vi "ConvertGoop3ToGoop4.vi"() -> (0 "error out":errorcluster)   [LabVIEW 2020]
uses:
  <resource>/Framework/Providers/Open_GDS/ClassProviders/Common/ConvertGoop3ToGoop4_SubVIs/ConvertGoop3ToGoop4_ClassType.ctl
  <resource>/Framework/Providers/Open_GDS/ClassProviders/Common/LvClass_class/GDSLvCLass_ClassSettingsType.ctl
  <resource>/Framework/Providers/Open_GDS/ClassProviders/Common/LvClass_class/GDSLvClass_PlugIn.ctl
  <resource>/Framework/Providers/Open_GDS/ClassProviders/Common/LvClass_class/GDSLvClass_PlugInTypes.ctl
  <vilib>/Utility/miscctls.llb/LVPositionTypeDef.ctl
  <resource>/Framework/Providers/Open_GDS/ClassProviders/Provider_BaseClassInterface/CreateClassData.ctl
  <resource>/Framework/Providers/Open_GDS/ClassProviders/Provider_EndevoGOOP300/Templates/EndevoTemplateNames.ctl
  <resource>/Framework/Providers/Open_GDS/ClassProviders/Provider_EndevoGOOP400/Templates/EndevoG4TemplateNames.ctl
  <resource>/Framework/Providers/Open_GDS/ClassProviders/Provider_EndevoGOOP400/ClassWriterGOOP400_class/ClassWriterGOOP400.lvclass
  <resource>/Framework/Providers/Open_GDS/ClassProviders/Common/ScriptingFunctions/Scripting_ConnectorPanePatternType.ctl
  <resource>/Framework/Providers/Open_GDS/ClassProviders/Provider_BaseClassInterface/AddDesignPatternData.ctl
  <resource>/Framework/Providers/Open_GDS/ClassProviders/Common/CommonVIs/CommonVIs_AttributeDataType.ctl
  <resource>/Framework/Providers/Open_GDS/ClassProviders/Provider_BaseClassInterface/ClassWriter_class/ClassWriter.lvclass
  <vilib>/Utility/miscctls.llb/LVPointTypeDef.ctl
  <vilib>/Utility/error.llb/DialogType.ctl
  <resource>/Framework/Providers/Open_GDS/ClassProviders/Common/ConvertGoop3ToGoop4_SubVIs/ConvertGoop3ToGoop4_LogType.ctl
  <vilib>/regexp/Match Regular Expression.xnode
panel:
  in  "Cancel":bool
  in  "Next":bool
  out "Tab":T1(tab)
  out "ErrorMessage":string
  in  "Current GOOP3 top directory":path
  in  "Toggle":bool
  in  "GOOP3 classes found":i32[](listbox)
  in  "ApplyDebuggingSupport":bool
  in  "ApplyPersistentPattern":bool
  in  "Project":path caption="This project will be created and used to update the classes in."
  in  "Progress":i32(listbox)=-1
  in  "Done":bool
  out "State":string="Idle"
  out "Timer":string
  # "1."
  # "Select Top folder to start a recursive search for GOOP3 classes and application VIs."
  # "2."
  # "These classes\nhave been found.\n\nDo you want to convert them?"
  # "3."
  # "Have you backed up all your VIs in the selected folder?"
  # "Have you checked that all files in\nthe selected folder are writeable?"
  # "4."
  # "Save VI dialog boxes!?!\nIt might pop up dialog boxes that asks you to save VIs that will be unloaded from memory, JUST press cancel for those."
  # "Revert dialog boxes!?!\nIt might pop up dialog boxes that prompts that changes has been done on disk, JUST press cancel for those."
  # "5."
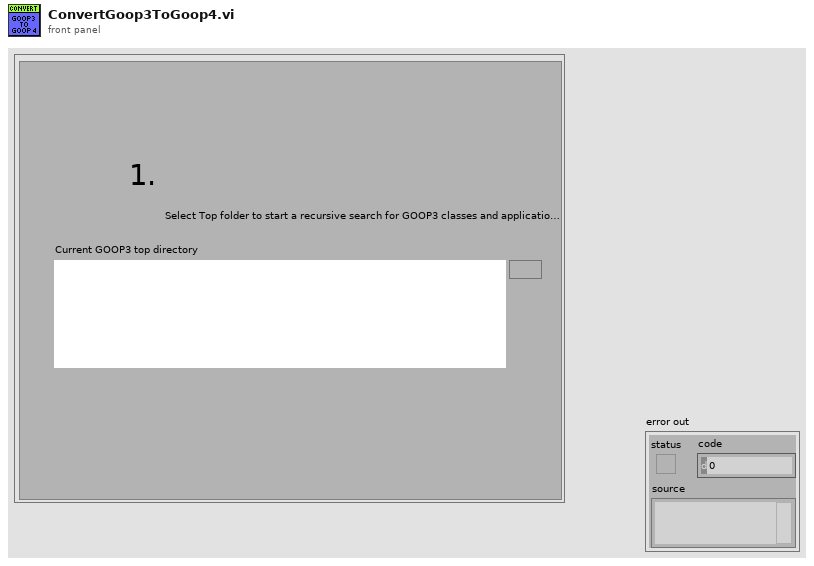
[diagram p1: front panel]
types:
  T1 = enum32{"SelectDir", "ClassesFound", "BackedUp", "Start?", "Converting"}
  T2 = typedef "ConvertGoop3ToGoop4_ClassType.ctl" = cluster{"NoOfInheritance":i32, "LvClassPath":path, "ClassName":string, "ClassPrefix":string, "IsLLB":bool, "ClassFolder":path, "ViRefs":refnum<vi>[], "ClassRef":refnum<vi>, "InheritsFrom":path, "RootClass":path, "ViPathes":path[], "AllInheritanceClasses":path[], "TemplateVersionUsed":string, "UsingClassAttributes":bool, "ClassSettings":T3, "HeaderIcon":u8[][], "GetAttViRefs":refnum<vi>[], "VIsModiifingData":refnum<vi>[], "Singleton":bool, "BrokenVIs":string[], "ObjectStatusUsed":bool, "DestrotCleanUpViName":string}
  T3 = typedef "GDSLvCLass_ClassSettingsType.ctl" = cluster{"ClassProviderName":string, "ClassTemplateUsed":string, "ClassTemplateVersion":string, "ClassDescription":string, "PlugIns":T4[], "ConnectorPanePattern":string}
  T4 = typedef "GDSLvClass_PlugIn.ctl" = cluster{"Type":T5, "ID":string, "Version":string, "Path":path, "Name":string, "Data":variant}
  T5 = typedef "GDSLvClass_PlugInTypes.ctl" = enum16{"DesignPattern", "MethodTypes"}
  T6 = typedef "LVPositionTypeDef.ctl" = cluster{"Left":i32, "Top":i32}
  T7 = cluster{"TopFolderPath":path, "Classes":T2[], "error":errorcluster, "Project":path, "ProjectRef":refnum<vi>, "My Computer":refnum<vi>, "AppRef":refnum<vi>, "CallParentMethod":cluster{"VIRef":refnum<vi>, "Position":T6}[], "CopyClasses":path, "TemplateVersions":string[], "LLBsToDelete":path[], "CopyClassesRef":refnum<vi>[], "CopyClassPaths":path[], "Deselect":bool, "SelectedClasses":i32[], "DeleteTheseFiles":path[], "Log":bool}
  T8 = enum8{"Enabled", "Disabled", "Disabled and Grayed Out"}
  T9 = cluster{"Current GOOP3 top directory":path, i32[]}
  T10 = typedef "ClassWriter.lvclass/CreateClassData.ctl" = cluster{"ClassName":string, "ClassFolder":path, "ClassDescription":string, "ClassTemplateOptions":string, "BaseClass(ProjectStringPath or LvClassFilePath)":variant, "ExtraCreateParameters":variant, "FolderSuffix":string}
  T11 = typedef "EndevoG4TemplateNames.ctl" = enum16{"G4BaseTemplate_Simple_4x4x4", "G4SubTemplate_Simple_4x4x4", "G4BaseTemplate_Simple_6x8x6", "G4SubTemplate_Simple_6x8x6", "G4BaseTemplate_Singleton_4x4x4", "G4SubTemplate_Singleton_4x4x4", "G4BaseTemplate_Singleton_6x8x6", "G4SubTemplate_Singleton_6x8x6", "G4InterfaceTemplate_6x8x6", "G4InterfaceTemplate_4x4x4", "G4BaseTemplate_Simple_5x6x5", "G4BaseTemplate_Singleton_5x6x5", "G4InterfaceTemplate_5x6x5", "G4SubTemplate_Simple_5x6x5", "G4SubTemplate_Singleton_5x6x5"}
  T12 = typedef "EndevoTemplateNames.ctl" = enum16{"BaseTemplate", "SubTemplate", "BaseTemplate_4x4x4", "SubTemplate_4x4x4", "SingletonTemplate"}
  T13 = cluster{"ID":string, "Path":path, "Name":string, "Desc":string, "Version":string, "DependenciesID":string[], "OnlyOne":bool}[]
  T14 = typedef "CommonVIs_AttributeDataType.ctl" = enum16{"UINT8", "INT8", "UINT16", "INT16", "UINT32", "INT32", "UINT64", "INT64", "SGL", "DBL", "EXT", "CSG", "CDB", "CXT", "TimeStamp", "STRING", "PATH", "BOOL", "ENUM", "RefNum", "VIRefNum", "LabVIEW Class", "Cluster", "Variant", "TypeDef", "Waveform", "LabVIEW Object", "Other", "void"}
  T15 = cluster{"ProcessName":cluster{"Name":string, "Array?":u16, "AttributeDataType":T14, "GetMethod":bool, "SetMethod":bool}[]}
  T16 = typedef "LVPointTypeDef.ctl" = cluster{"Horizontal":i16, "Vertical":i16}
  T17 = enum32{"invalid scope", "public", "private", "protected", "community"}
  T18 = typedef "ConvertGoop3ToGoop4_LogType.ctl" = enum16{"Enter", "Read"}
  T19 = typedef "eventvkey.ctl" = enum16{"ASCII", "Enter", "Return", "Shift", "Ctrl", "Alt", "Cmd", "Opt", "Caps", "NumLock", "Clear", "Break", "Up", "Down", "Left", "Right", "Insert", "Delete", "Home", "End", "PageUp", "PageDown", "Escape", "Help", "Pause", "ScrollLock", "F1", "F2", "F3", "F4", "F5", "F6", "F7", "F8", "F9", "F10", "F11", "F12", "F13", "F14", "F15", "F16", "F17", "F18", "F19", "F20", "F21", "F22", "F23", "F24", "Play", "VolumeUp", "VolumeDown", "Mute", "Two Byte Char"}
  T20 = enum32{"Bad", "Idle", "Run top level", "Running"}
  T21 = enum16{"Left Button", "Center Button", "Right Button", "Window Close"}
  T22 = typedef "Scripting_ConnectorPanePatternType.ctl" = u16
  T23 = typedef "GOOP_WireConfigurationType.ctl" = cluster{"Edge thickness":i32, "Edge color":u32, "Center thickness":i32, "Center pattern":T24, "CenterColor1":u32, "CenterColor2":u32, "Tunnels and terminals colors":u32}
  T24 = typedef "GOOP_WirePattern.ctl" = enum16{"Solid", "Large dash", "Small dash"}
  T25 = typedef "DesignPatternsData.ctl" = cluster{"Type":string, "Patterns":cluster{"ID":string, "Path":path, "Name":string, "Desc":string, "Version":string, "DependenciesID":string[], "OnlyOne":bool}[]}
  T26 = cluster{"ID":string, "Path":path, "Name":string, "Desc":string, "Version":string, "DependenciesID":string[], "OnlyOne":bool}
  T27 = typedef "AddDesignPatternData.ctl" = cluster{"Type":string, "ID":string, "Version":string, "VIPath":path, "Name":string, "Data":variant}
  T28 = enum32{"invalid VI type", "Standard VI", "Control VI", "Global VI", "Polymorphic VI", "Configuration VI", "SubSystem", "Facade VI", "Method VI", "Statechart Diagram VI"}
  T29 = typedef "DialogType.ctl" = u16
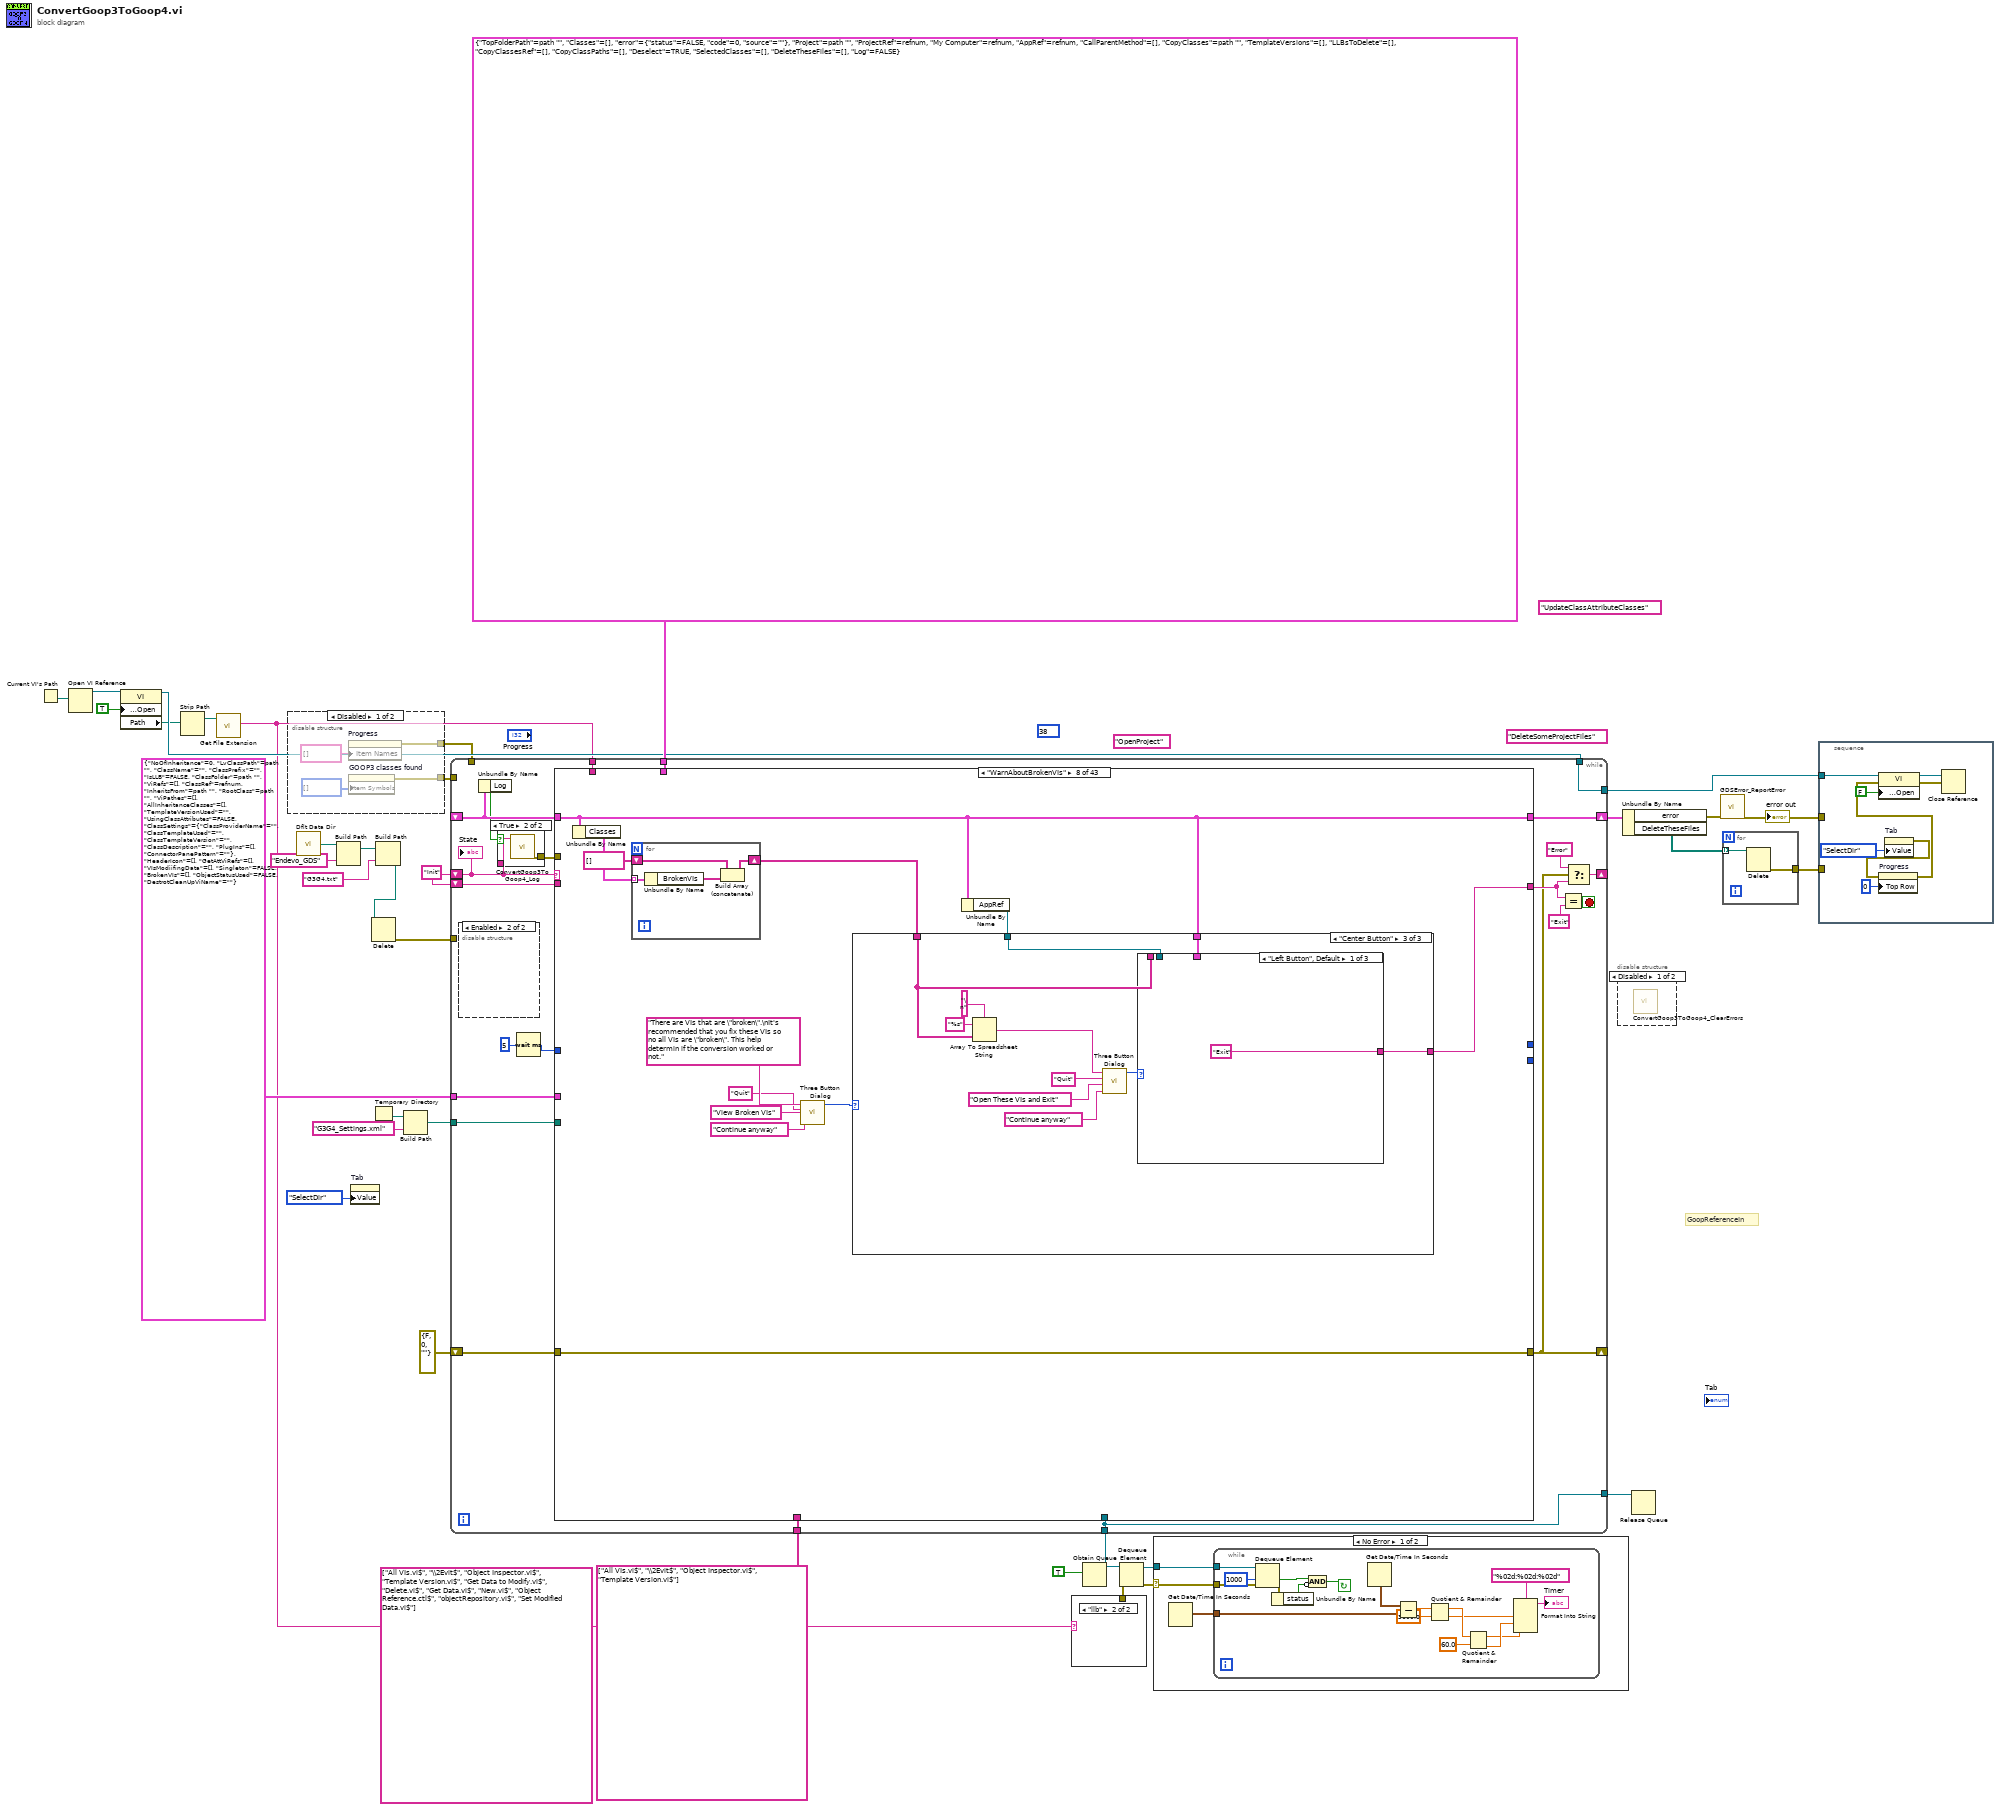
[diagram p0: block diagram]
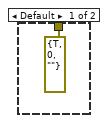
[diagram p2: hidden frame]
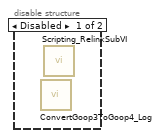
[diagram p7: hidden frame]
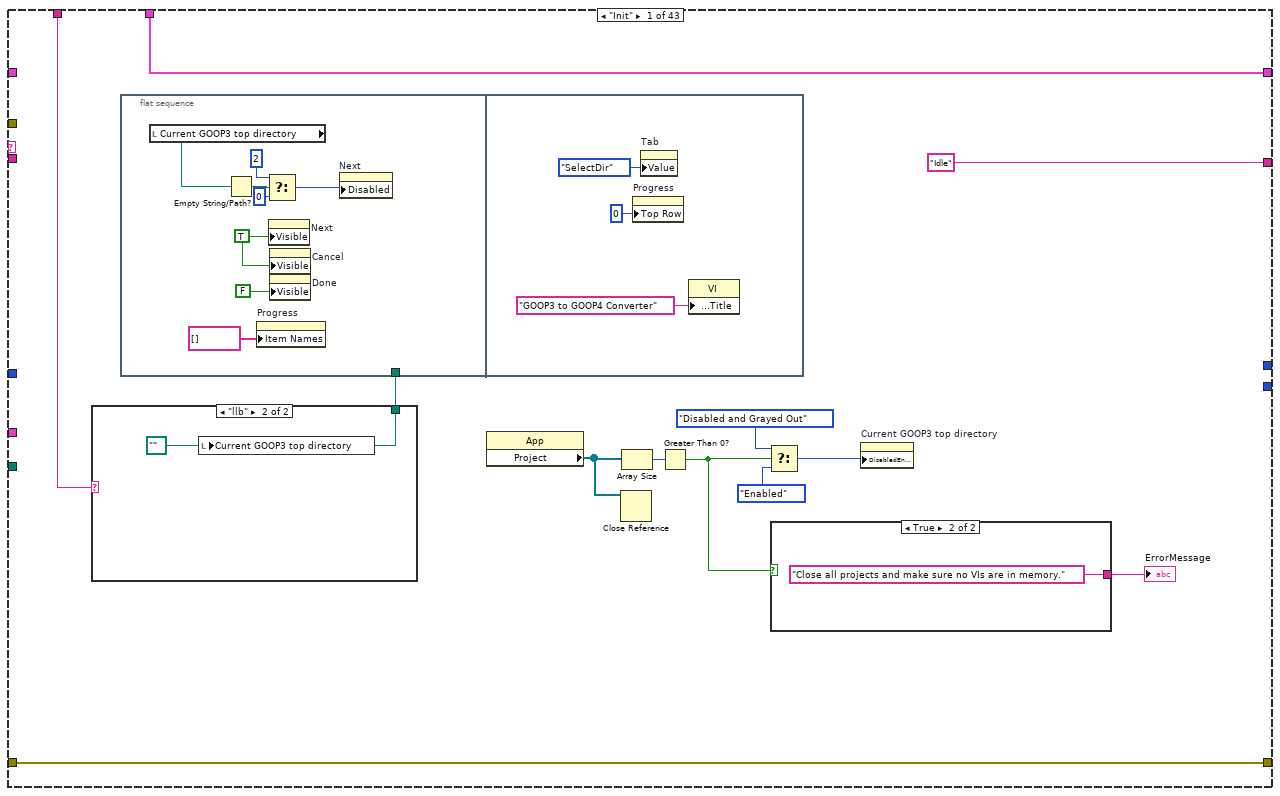
[diagram p8: hidden frame]
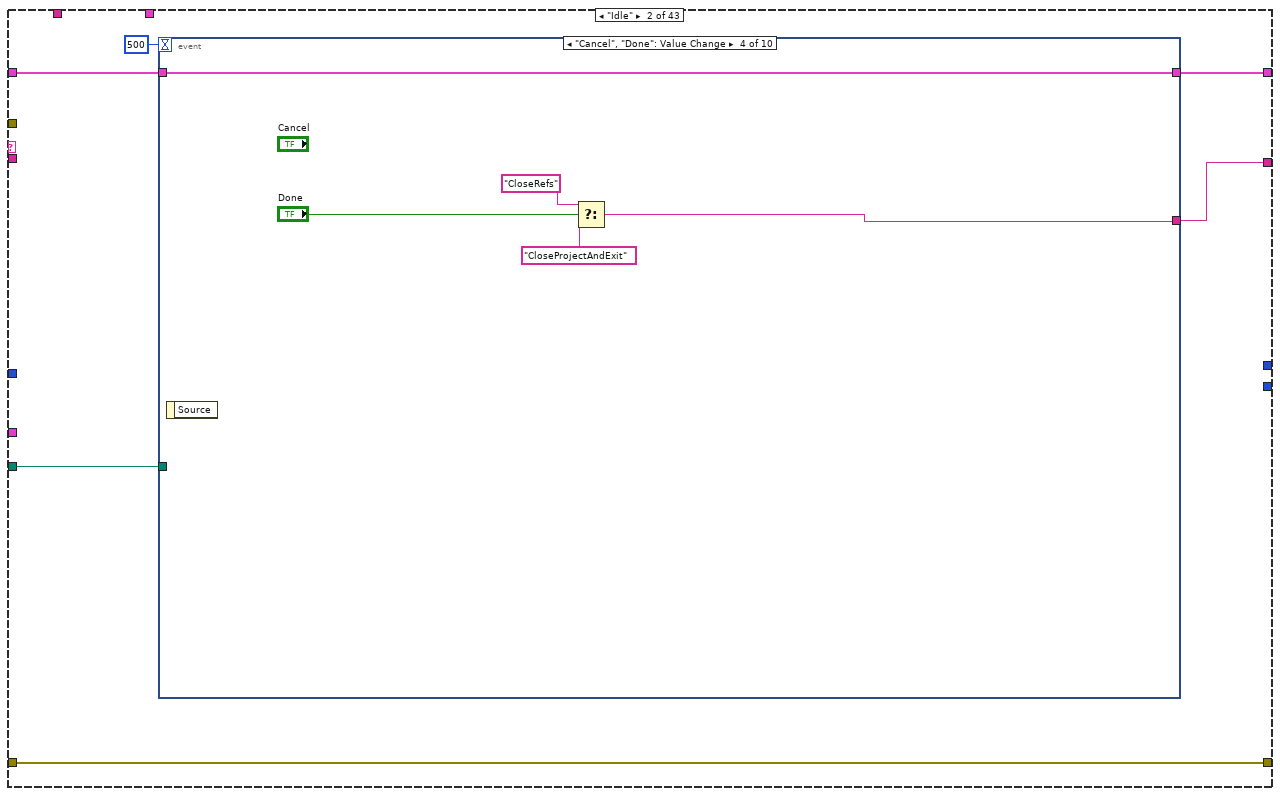
[diagram p11: hidden frame]
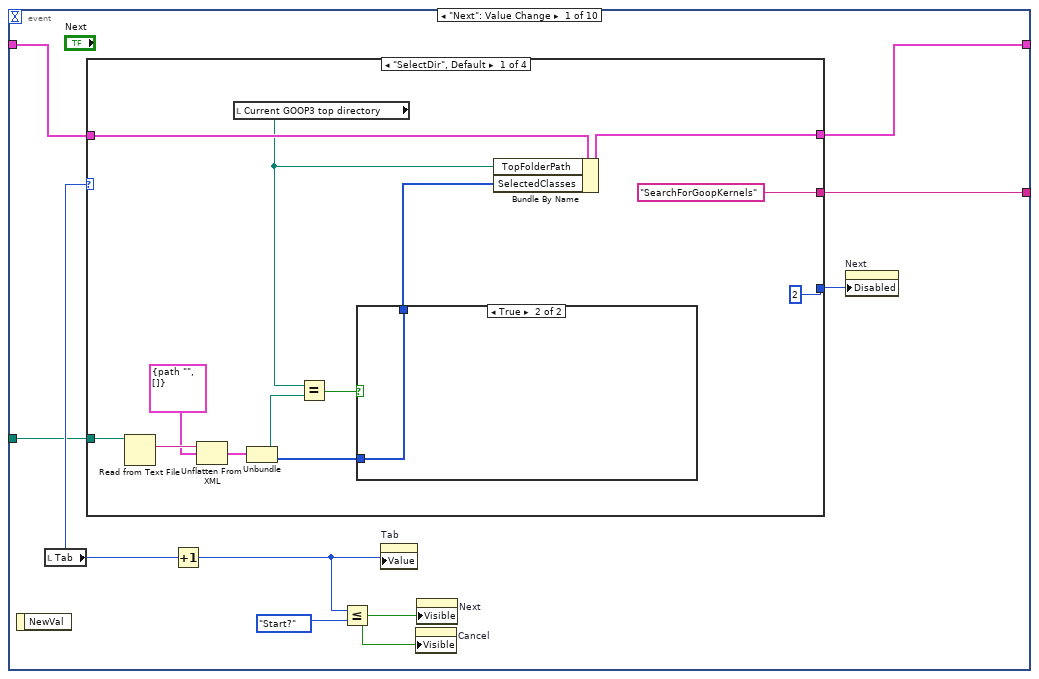
[diagram p12: hidden frame]
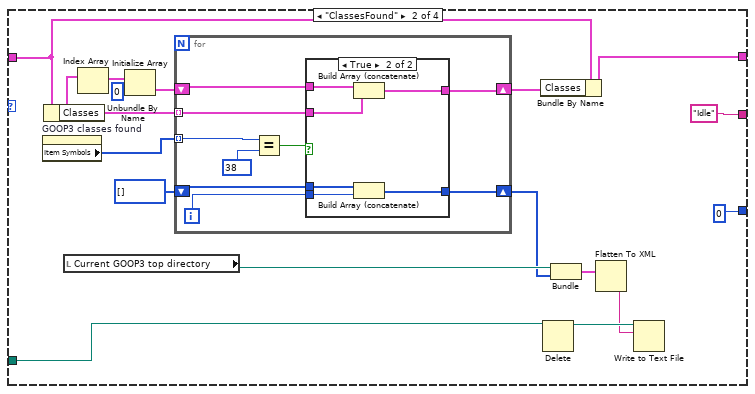
[diagram p14: hidden frame]
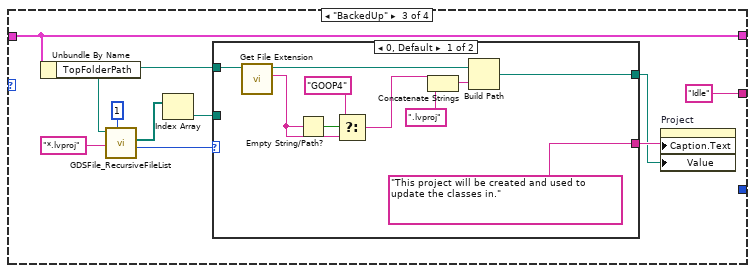
[diagram p16: hidden frame]
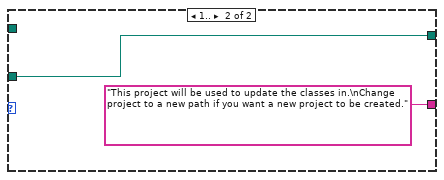
[diagram p17: hidden frame]
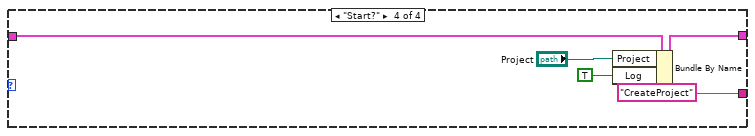
[diagram p18: hidden frame]
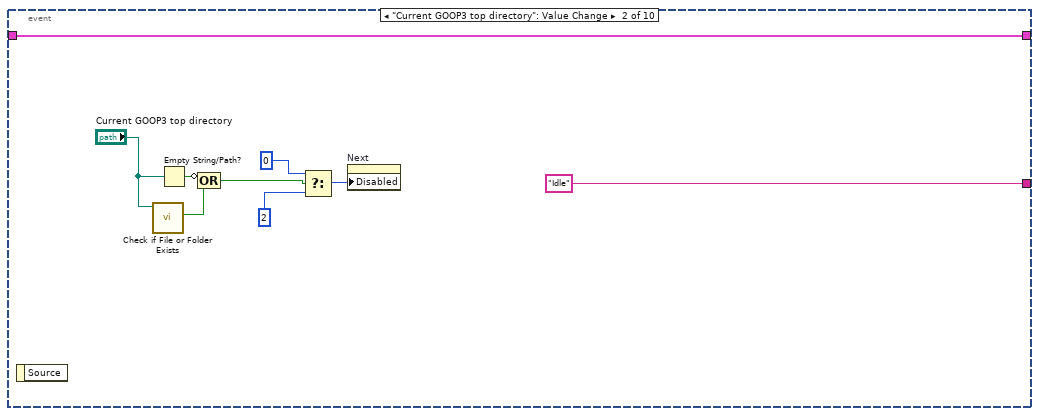
[diagram p19: hidden frame]
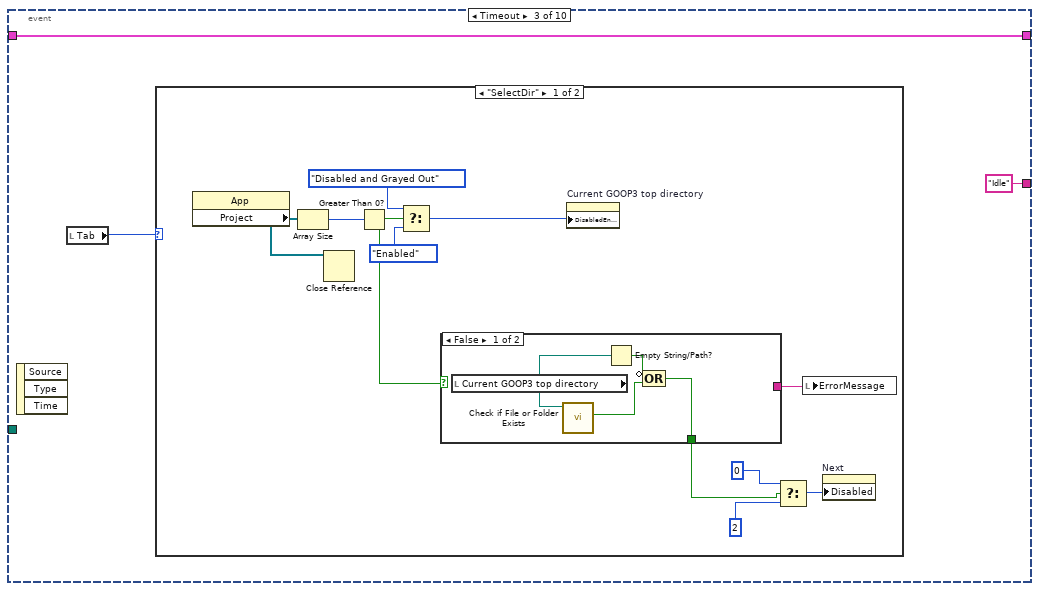
[diagram p20: hidden frame]
diagram:
  (unwired) "DeleteSomeProjectFiles"
  (unwired) "OpenProject"
  (unwired) 38
  (unwired) "UpdateClassAttributeClasses"
  (unwired) string[] ["All VIs.vi$", "\\2Evit$", "Object Inspector.vi$", "Template Version.vi$", "Get Data to Modify.vi$", "Delete.vi$", "Get Data.vi$", "New.vi$", "Object Reference.ctl$", "objectRepository.vi$", "Set Modified Data.vi$"] ("file names")
  w33 = "Init"
  # "GoopReferenceIn"
  n1 = Current VI's Path() -> (path=w29:path)
  n2 = Open VI Reference(vi path=w29) -> (vi reference=w28:refnum<vi>)  [unwired: 5 in, 1 out]
  n3 = property class="VI"(reference=w28, "Front Panel.Open"=TRUE ("Front Panel Window:Open")) -> (reference out=w27:refnum<vi>, "Path"=w15:path)  [unwired: 1 in, 1 out]
  n4 = Strip Path(path=w15) -> (stripped path=w14:path)  [unwired: 1 out]
  n5 = call <vilib>:"Get File Extension.vi"("file"=w14) -> ("lowercase file extension"=w3:string)  [unwired: 6 in, 4 out]
  n6 = disable-structure shown="Disabled" {
    disable-tunnel: [w38 _] -> w13
    disable-tunnel: [w37 _] -> w12
    frame Disabled {
      n7 = property on="Progress" class="LstBox (strict)"("Item Names"=string[] []) -> (error out=w37:errorcluster)  [unwired: 2 in, 1 out]
      n8 = property on="GOOP3 classes found" class="LstBox (strict)"("Item Symbols"=i32[] []) -> (error out=w38:errorcluster)  [unwired: 2 in, 1 out]
    }
    frame Enabled {
    }
  }
  n9 = call <vilib>:"Dflt Data Dir.vi"() -> ("App:Default Data Directory"=w9:path)
  n10 = Build Path(base path=w9, name or relative path="Endevo_GDS") -> (appended path=w7:path)
  n11 = property on="Tab" class="TabCtl (strict)"("Value"=T1."SelectDir" ("Tab")) -> ()  [unwired: 2 in, 2 out]
  n12 = Temporary Directory() -> (w22:path)
  n13 = Build Path(base path=w7, name or relative path="G3G4.txt") -> (appended path=w5:path)
  n14 = Delete(path (use dialog)=w5) -> (error out=w31:errorcluster)  [unwired: 4 in, 2 out]
  n15 = Build Path(base path=w22, name or relative path="G3G4_Settings.xml") -> (appended path=w21:path)
  n16 = case shown="\"llb\"" w3 {
    tunnel: [errorcluster {"status"=TRUE, "code"=0, "source"=""} ("error in (no error)") _] -> w4
    frame Default {
    }
    frame "llb" {
    }
  }
  n17 = Obtain Queue(element data type=TRUE) -> (queue out=w19:refnum<queue>)  [unwired: 4 in, 2 out]
  n18 = while {
    shift-right: [w51] -> _
    shift-left: errorcluster {"status"=FALSE, "code"=0, "source"=""} ("error IO") -> [w50]
    shift-right: [w63] -> _
    shift-left: w33 -> [w44]
    shift-right: [w58] -> w32
    shift-left: _ -> [w43]
    tunnel: T7 {"TopFolderPath"=path "", "Classes"=[], "error"={"status"=FALSE, "code"=0, "source"=""}, "Project"=path "", "ProjectRef"=refnum, "My Computer"=refnum, "AppRef"=refnum, "CallParentMethod"=[], "CopyClasses"=path "", "TemplateVersions"=[], "LLBsToDelete"=[], "CopyClassesRef"=[], "CopyClassPaths"=[], "Deselect"=TRUE, "SelectedClasses"=[], "DeleteTheseFiles"=[], "Log"=FALSE} -> [w57]
    tunnel: string[] ["All VIs.vi$", "\\2Evit$", "Object Inspector.vi$", "Template Version.vi$"] ("file names") -> [w56]
    shift-left: w33 -> [w55]
    tunnel: w31 -> [_]
    tunnel: w27 -> [w52]
    tunnel: [w52] -> w25
    tunnel: T2 {"NoOfInheritance"=0, "LvClassPath"=path "", "ClassName"="", "ClassPrefix"="", "IsLLB"=FALSE, "ClassFolder"=path "", "ViRefs"=[], "ClassRef"=refnum, "InheritsFrom"=path "", "RootClass"=path "", "ViPathes"=[], "AllInheritanceClasses"=[], "TemplateVersionUsed"="", "UsingClassAttributes"=FALSE, "ClassSettings"={"ClassProviderName"="", "ClassTemplateUsed"="", "ClassTemplateVersion"="", "ClassDescription"="", "PlugIns"=[], "ConnectorPanePattern"=""}, "HeaderIcon"=[], "GetAttViRefs"=[], "VIsModiifingData"=[], "Singleton"=FALSE, "BrokenVIs"=[], "ObjectStatusUsed"=FALSE, "DestrotCleanUpViName"=""} ("output cluster") -> [w49]
    tunnel: w21 -> [w48]
    tunnel: w19 -> [w46]
    tunnel: [w46] -> w18
    tunnel: w13 -> [_]
    tunnel: w12 -> [_]
    tunnel: w3 -> [w45]
    stop <- w62 stop-if-true
    n19 = disable-structure shown="Enabled" {
      frame Disabled {
        n20 = call <resource>:"ConvertGoop3ToGoop4_Log.vi"() -> ()  [unwired: 9 in, 3 out]
        n21 = call <resource>:"Scripting_RelinkSubVI.vi"() -> ()  [unwired: 10 in, 2 out]
      }
      frame Enabled {
      }
    }
    n22 = Unbundle By Name(w43) -> ("Log"=w42:bool)
    n23 = case shown="True" w42 {
      tunnel: [_ w65] -> w47
      tunnel: w44 -> [_ w64]
      frame False {
      }
      frame True {
        n24 = call <resource>:"ConvertGoop3ToGoop4_Log.vi"("Object"=w64) -> ("error out"=w65:errorcluster)  [unwired: 8 in, 2 out]
      }
    }
    n25 = Wait (ms)(milliseconds to wait=u32 5) -> (millisecond timer value=w53:u32)
    n26 = case shown="\"WarnAboutBrokenVIs\"" w44 {
      selector: w44 -> [_ _ _ _ _ _ _ _ _ _ _ _ _ _ _ _ _ _ _ _ _ _ _ _ _ _ _ _ _ _ _ _ _ _ _ _ _ _ _ _ _ _ w2354]
      tunnel: [w76 w93 w332 w506 w517 w554 w621 w714 w756 w786 w844 w897 w953 w1018 w1058 w1160 w1222 w1330 w1359 w1417 w1478 w1485 w1508 w1538 w1620 w1703 w1762 w1804 w1810 w1850 w1887 w1959 w1994 w2050 w2092 w2154 w2235 w2269 w2273 w2310 w2319 w2326 errorcluster {"status"=FALSE, "code"=0, "source"=""} ("error IO")] -> w51
      tunnel: ["Idle" w94 w327 "Idle" "AddClassesToProject" "AnalyseClasses" w612 w717 "FindGetObjectStatus" "FindGetAttributes" "FindNewVIs" "RenameVIsIfNeeded" "SaveAndCloseProject" "CreateGOOP4Classes" "RenameDestory" "ApplyDesignPatterns" "CloseCopyClasses" "CopyNewClassVIsToOldClasses" "ModifyClassPrivateData" "OpenMainProjectAgain" "Idle" "OpenClassReferences" "ReplaceGetAttToModifyToGetAttribute" "RewireGetAttributes" "RewireGetObjectStatus" "RemoveGetObjectStatus" "UpdateSubClass-GetAttributesWithUnbundleByName" "Exit" "CreateIP-Nodes" "UpdateObjectAttributes" "MakeVIsProtected" "UpdateNewViCallers" "UpdateDestory" "DeleteNotUsedClassItems" "DeleteSomeProjectFiles" "OpenProject" "Done" "CheckForBrokenVIs" w2276 "Idle" "Idle" "Exit" "Exit"] -> w59
      tunnel: [w75 w95 w349 w508 w531 w565 w622 w713 w760 w781 w846 w899 w948 w1030 w1068 w1155 w1219 w1341 w1363 w1419 w1480 w1502 w1514 w1534 w1618 w1699 w1764 w1806 w1812 w1852 w1889 w1961 w1996 w2052 w2088 w2157 w2234 w2268 w2279 w2306 w2321 w2327 w2343] -> w58
      tunnel: w43 -> [_ w96 w350 w508 w532 w561 w623 w713 w762 w782 w846 w899 w949 w1030 w1069 w1155 w1220 w1341 w1363 w1419 w1480 w1503 w1510 w1535 w1619 w1700 w1764 w1806 w1812 w1852 w1889 w1961 w1996 w2052 w2089 w2157 w2234 w2268 w2280 w2306 w2321 w2327 w2351]
      tunnel: w57 -> [w75 _ _ _ _ _ _ _ _ _ _ _ _ _ _ _ _ _ _ _ _ _ _ _ _ _ _ _ _ _ _ _ _ _ _ _ _ _ _ _ _ _ _]
      tunnel: w56 -> [_ _ _ _ _ _ _ _ _ _ _ _ _ _ _ _ _ _ _ _ _ _ _ _ _ _ _ _ _ _ _ _ _ _ _ _ _ _ _ _ _ _ _]
      tunnel: w55 -> [_ _ _ _ _ _ _ _ _ _ _ _ _ _ _ _ _ _ _ _ _ _ _ _ _ _ _ _ _ _ _ _ _ _ _ _ _ _ _ _ _ _ w2353]
      tunnel: w53 -> [_ _ _ _ _ _ _ _ _ _ _ _ _ _ _ _ _ _ _ _ _ _ _ _ _ _ _ _ _ _ _ _ _ _ _ _ _ _ _ _ _ _ _]
      tunnel: w50 -> [w76 w93 w348 w506 w520 w557 w621 w714 w756 w787 w845 w898 w954 w1026 w1059 w1154 w1226 w1348 w1360 w1418 w1478 w1492 w1507 w1539 w1621 w1704 w1763 w1804 w1811 w1851 w1888 w1960 w1995 w2051 w2093 w2156 w2241 w2269 w2273 w2310 w2319 w2326 w2331]
      tunnel: w49 -> [_ _ w340 _ _ _ _ _ _ _ _ _ _ _ _ _ _ _ _ _ _ _ _ _ _ _ _ _ _ _ _ _ _ _ _ _ _ _ _ _ _ _ _]
      tunnel: w48 -> [_ w92 _ _ _ _ _ _ _ _ _ _ _ _ _ _ _ _ _ _ _ _ _ _ _ _ _ _ _ _ _ _ _ _ _ _ _ _ _ _ _ _ _]
      tunnel: [_ _ _ _ w512 _ _ _ _ _ _ _ _ _ _ _ _ _ _ _ _ _ _ _ _ _ _ _ _ _ _ _ _ _ _ _ _ _ _ _ _ _ _] -> _
      tunnel: [_ _ _ _ _ _ _ _ _ _ _ _ _ _ _ _ _ _ _ _ _ w1482 _ _ _ _ _ _ _ _ _ _ _ _ _ _ _ _ _ _ _ _ _] -> _
      tunnel: w47 -> [_ _ _ _ _ _ _ _ _ _ _ _ _ _ _ _ _ _ _ _ _ _ _ _ _ _ _ _ _ _ _ _ _ _ _ _ _ _ _ _ _ _ _]
      tunnel: w46 -> [_ _ _ _ w511 _ _ _ _ _ _ _ _ _ _ _ _ _ _ _ _ _ _ _ _ _ _ _ _ _ _ _ _ _ _ _ _ w2259 _ _ _ _ w2333]
      tunnel: w45 -> [w74 _ _ _ _ _ _ _ _ _ _ _ _ _ _ _ _ _ _ _ _ _ _ _ _ _ _ _ _ _ _ _ _ _ _ _ _ _ _ _ _ _ _]
      frame "Init" {
        n27 = case shown="\"llb\"" w74 {
          tunnel: [_ w79] -> w73
          frame Default {
          }
          frame "llb" {
            w79 = path "" ("Current GOOP3 top directory")
            n28 = local write "Current GOOP3 top directory"(w79) -> ()
          }
        }
        n29 = flat-sequence {
          tunnel: w73 -> [_]
          frame #0 {
            w87 = TRUE ("Visible")
            n30 = local read "Current GOOP3 top directory"() -> (w84:path)
            n31 = Empty String/Path?(string/path=w84) -> (empty?=w83:bool)
            n32 = property on="Progress" class="LstBox (strict)"("Item Names"=string[] []) -> ()  [unwired: 2 in, 2 out]
            n33 = Select(t=u8 2 ("Disabled"), s=w83, f=u8 0) -> (s? t:f=w81:u8)
            n34 = property on="Next" class="Bool"("Visible"=w87) -> ()  [unwired: 2 in, 2 out]
            n35 = property on="Cancel" class="Bool"("Visible"=w87) -> ()  [unwired: 2 in, 2 out]
            n36 = property on="Done" class="Bool"("Visible"=FALSE) -> ()  [unwired: 2 in, 2 out]
            n37 = property on="Next" class="Bool"("Disabled"=w81) -> ()  [unwired: 2 in, 2 out]
          }
          frame #1 {
            n38 = property on="Progress" class="LstBox (strict)"("Top Row"=0) -> ()  [unwired: 2 in, 2 out]
            n39 = property on="Tab" class="TabCtl (strict)"("Value"=T1."SelectDir" ("Tab")) -> ()  [unwired: 2 in, 2 out]
            n40 = property class="VI"("Front Panel.Title"="GOOP3 to GOOP4 Converter" ("Front Panel Window:Title")) -> ()  [unwired: 2 in, 2 out]
          }
        }
        n41 = property class="App"() -> ("Project"=w72:refnum<vi>[])  [unwired: 2 in, 2 out]
        n42 = Close Reference(reference=w72) -> ()  [unwired: 1 in, 1 out]
        n43 = Array Size(array=w72) -> (size(s)=w71:i32)
        n44 = Greater Than 0?(x=w71) -> (x > 0?=w67:bool)
        n45 = Select(t=T8."Disabled and Grayed Out" ("Disabled"), s=w67, f=T8."Enabled" ("Disabled")) -> (s? t:f=w70:T8)
        n46 = case shown="True" w67 {
          tunnel: [_ "Close all projects and make sure no VIs are in memory."] -> w66
          frame False {
          }
          frame True {
          }
        }
        "ErrorMessage" <- w66
        n47 = property on="Current GOOP3 top directory" class="Path"("DisabledEnum"=w70) -> ()  [unwired: 2 in, 2 out]
      }
      frame "Idle" {
        n48 = event shown="[3] \"Cancel\", \"Done\": Value Change" {
          selector: _ -> [_ _ _ _ _ _ _ _ _ _]
          dyn-events: _ -> [_ _ _ _ _ _ _ _ _ _]
          timeout: 500 -> [_ _ _ _ _ _ _ _ _ _]
          tunnel: w96 -> [w103 w186 w191 w213 w216 w240 w262 w275 w318 w321]
          tunnel: [w102 w186 w191 w213 w215 w239 w261 w274 w318 w321] -> w95
          tunnel: [w101 "Idle" "Idle" ("t") w210 "Idle" "Idle" "Idle" "Idle" "Idle" "Idle"] -> w94
          tunnel: w92 -> [w97 _ _ _ _ _ _ _ _ _]
          event "Next": Value Change {
            n49 = event-data() -> ()  [unwired: 1 in, 1 out]
            n50 = local read "Tab"() -> (w104:T1)
            n51 = case shown="\"SelectDir\", Default" w104 {
              tunnel: w103 -> [w118 w128 w162 w177]
              tunnel: [w117 w134 w162 w180] -> w102
              tunnel: ["SearchForGoopKernels" "Idle" "Idle" "CreateProject"] -> w101
              tunnel: [u8 2 ("Disabled") u8 0 ("f") _ _] -> w100
              tunnel: w97 -> [w114 w122 _ _]
              frame "SelectDir", Default {
                n52 = Read from Text File(file (use dialog)=w114) -> (text=w113:string)  [unwired: 3 in, 3 out]
                n53 = Unflatten From XML(xml string=w113, type=T9 {"Current GOOP3 top directory"=path "", []} ("output cluster")) -> (value=w111:T9)  [unwired: 1 in, 1 out]
                n54 = local read "Current GOOP3 top directory"() -> (w110:path)
                n55 = Unbundle(w111) -> ("Current GOOP3 top directory"=w109:path, w106:i32[])
                n56 = Equal?(x=w110, y=w109) -> (x = y?=w108:bool)
                n57 = case shown="True" w108 {
                  tunnel: [_ w119] -> w107
                  tunnel: w106 -> [_ w119]
                  frame False {
                  }
                  frame True {
                  }
                }
                n58 = Bundle By Name(cluster=w118, "TopFolderPath"=w110, "SelectedClasses"=w107) -> (w117:T7)
              }
              frame "ClassesFound" {
                n59 = property on="GOOP3 classes found" class="LstBox (strict)"() -> ("Item Symbols"=w133:i32[])  [unwired: 2 in, 2 out]
                n60 = Unbundle By Name(w128) -> ("Classes"=w132:T2[])
                n61 = local read "Current GOOP3 top directory"() -> (w126:path)
                n62 = Index Array(array=w132) -> (element=w131:T2)  [unwired: 1 in]
                n63 = Initialize Array(w131, 0 ("dimension size")) -> (w129:T2[])
                n64 = for {
                  shift-right: [w142] -> w127
                  shift-left: w129 -> [w143]
                  tunnel: w132 -> [w141] mode=indexing
                  tunnel: w133 -> [w144] mode=indexing
                  shift-right: [w137] -> w124
                  shift-left: i32[] [] -> [w139]
                  i -> [w138]
                  n65 = Equal?(x=w144, y=38) -> (x = y?=w140:bool)
                  n66 = case shown="True" w140 {
                    tunnel: w143 -> [w147 w153]
                    tunnel: [w147 w152] -> w142
                    tunnel: w141 -> [_ w151]
                    tunnel: w139 -> [w146 w150]
                    tunnel: w138 -> [_ w149]
                    tunnel: [w146 w148] -> w137
                    frame False {
                    }
                    frame True {
                      n67 = Build Array (concatenate)(w153, w151) -> (w152:T2[])
                      n68 = Build Array (concatenate)(w150, w149) -> (w148:i32[])
                    }
                  }
                }
                n69 = Bundle By Name(cluster=w128, "Classes"=w127) -> (w134:T7)
                n70 = Delete(path (use dialog)=w122) -> (deleted path=w123:path)  [unwired: 4 in, 2 out]
                n71 = Bundle("Current GOOP3 top directory"=w126, w124) -> (w121:T9)  [unwired: 1 in]
                n72 = Flatten To XML(6:w121) -> (2:w120:string)
                n73 = Write to Text File(file (use dialog)=w123, text=w120) -> ()  [unwired: 2 in, 3 out]
              }
              frame "BackedUp" {
                n74 = Unbundle By Name(w162) -> ("TopFolderPath"=w156:path)
                n75 = call <resource>:"GDSFile_RecursiveFileList.vi"("pattern"="*.lvproj", "StopWhenNoOfFilesFound"=1, "Folder Path"=w156) -> ("Number of Files"=w158:i32, "All Files in Dir"=w159:path[])  [unwired: 4 in, 3 out]
                n76 = Index Array(array=w159) -> (element=w154:path)  [unwired: 1 in]
                n77 = case shown="0, Default" w158 {
                  tunnel: ["This project will be created and used to update the classes in." "This project will be used to update the classes in.\nChange project to a new path if you want a new project to be created."] -> w157
                  tunnel: w156 -> [w172 _]
                  tunnel: [w168 w174] -> w155
                  tunnel: w154 -> [_ w174]
                  frame 0, Default {
                    n78 = call <vilib>:"Get File Extension.vi"("file"=w172) -> ("lowercase file extension"=w166:string, "dup file"=w171:path)  [unwired: 6 in, 3 out]
                    n79 = Empty String/Path?(string/path=w166) -> (empty?=w167:bool)
                    n80 = Select(t="GOOP4", s=w167, f=w166) -> (s? t:f=w165:string)
                    n81 = Concatenate Strings(w165, ".lvproj" ("string")) -> (w169:string)
                    n82 = Build Path(base path=w171, name or relative path=w169) -> (appended path=w168:path)
                  }
                  frame 1.. {
                  }
                }
                n83 = property on="Project" class="Path"("Caption.Text"=w157, "Value"=w155) -> ()  [unwired: 2 in, 2 out]
              }
              frame "Start?" {
                n84 = Bundle By Name(cluster=w177, "Project"="Project", "Log"=TRUE) -> (w180:T7)
              }
            }
            n85 = Increment(x=w104) -> (x+1=w99:T1)
            n86 = Less Or Equal?(x=w99, y=T1."Start?" ("Tab")) -> (x <= y?=w105:bool)
            n87 = property on="Tab" class="TabCtl (strict)"("Value"=w99) -> ()  [unwired: 2 in, 2 out]
            n88 = property on="Cancel" class="Bool"("Visible"=w105) -> ()  [unwired: 2 in, 2 out]
            n89 = property on="Next" class="Bool"("Visible"=w105) -> ()  [unwired: 2 in, 2 out]
            n90 = property on="Next" class="Bool"("Disabled"=w100) -> ()  [unwired: 2 in, 2 out]
          }
          event "Current GOOP3 top directory": Value Change {
            n91 = event-data() -> ()  [unwired: 1 in, 1 out]
            n92 = call <vilib>:"Check if File or Folder Exists.vi"("path"="Current GOOP3 top directory") -> ("file or folder exists?"=w182:bool)  [unwired: 8 in, 2 out]
            n93 = Empty String/Path?(string/path="Current GOOP3 top directory") -> (empty?=w183:bool)
            n94 = Compound Arithmetic op=OR(invert w183, w182) -> (w181:bool)
            n95 = Select(t=u8 0, s=w181, f=u8 2 ("Disabled")) -> (s? t:f=w189:u8)
            n96 = property on="Next" class="Bool"("Disabled"=w189) -> ()  [unwired: 2 in, 2 out]
          }
          event Timeout {
            n97 = event-data() -> ()  [unwired: 1 in, 3 out]
            n98 = local read "Tab"() -> (w192:T1)
            n99 = case shown="\"SelectDir\"" w192 {
              frame "SelectDir" {
                n100 = property class="App"() -> ("Project"=w203:refnum<vi>[])  [unwired: 2 in, 2 out]
                n101 = Array Size(array=w203) -> (size(s)=w202:i32)
                n102 = Close Reference(reference=w203) -> ()  [unwired: 1 in, 1 out]
                n103 = Greater Than 0?(x=w202) -> (x > 0?=w197:bool)
                n104 = Select(t=T8."Disabled and Grayed Out" ("Disabled"), s=w197, f=T8."Enabled" ("Disabled")) -> (s? t:f=w201:T8)
                n105 = case shown="False" w197 {
                  tunnel: [_ "Close all projects and make sure no VIs are in memory."] -> w198
                  tunnel: [w204 _] -> w193
                  frame False {
                    n106 = local read "Current GOOP3 top directory"() -> (w206:path)
                    n107 = call <vilib>:"Check if File or Folder Exists.vi"("path"=w206) -> ("file or folder exists?"=w205:bool)  [unwired: 8 in, 2 out]
                    n108 = Empty String/Path?(string/path=w206) -> (empty?=w207:bool)
                    n109 = Compound Arithmetic op=OR(invert w207, w205) -> (w204:bool)
                  }
                  frame True {
                  }
                }
                n110 = property on="Current GOOP3 top directory" class="Path"("DisabledEnum"=w201) -> ()  [unwired: 2 in, 2 out]
                n111 = Select(t=u8 0, s=w193, f=u8 2 ("Disabled")) -> (s? t:f=w196:u8)
                n112 = local write "ErrorMessage"(w198) -> ()
                n113 = property on="Next" class="Bool"("Disabled"=w196) -> ()  [unwired: 2 in, 2 out]
              }
              frame Default {
              }
            }
          }
          event "Cancel", "Done": Value Change {
            n114 = event-data() -> ()  [unwired: 1 in, 1 out]
            n115 = Select(t="CloseRefs", s="Done", f="CloseProjectAndExit") -> (s? t:f=w210:string)
          }
          event "GOOP3 classes found": Value Change {
            n116 = event-data() -> ()  [unwired: 1 in, 6 out]
            n117 = property on="GOOP3 classes found" class="LstBox (strict)"() -> ("Item Symbols"=w227:i32[])  [unwired: 2 in, 2 out]
            n118 = Index Array(array="GOOP3 classes found") -> (element=w226:i32)  [unwired: 1 in]
            n119 = Empty Array?(array="GOOP3 classes found") -> (empty?=w225:bool)
            n120 = Select(t=T8."Enabled" ("Disabled"), s=w225, f=T8."Enabled" ("Disabled")) -> (s? t:f=w231:T8)
            n121 = Index Array(array=w227, index=w226) -> (element=w221:i32)
            n122 = Equal?(x=w221, y=38) -> (x = y?=w214:bool)
            n123 = Select(t="Deselect (Space)", s=w214, f="Select (Space)") -> (s? t:f=w217:string)
            n124 = Select(t="Select one or more classes", s=w225, f=w217) -> (s? t:f=w223:string)
            n125 = Build Array(w223) -> (w222:string[])
            n126 = Bundle By Name(cluster=w216, "Deselect"=w214) -> (w215:T7)
            n127 = property on="Toggle" class="Bool"("DisabledEnum"=w231, "Strings [4]"=w222) -> ()  [unwired: 2 in, 2 out]
          }
          event "Toggle": Value Change {
            n128 = event-data() -> ()  [unwired: 1 in, 6 out]
            n129 = local read "GOOP3 classes found"() -> (w245:i32[])
            n130 = Unbundle By Name(w240) -> ("Deselect"=w238:bool)
            n131 = property on="GOOP3 classes found" class="LstBox (strict)"() -> ("Item Symbols"=w246:i32[])  [unwired: 2 in, 2 out]
            n132 = Select(t=37, s=w238, f=38) -> (s? t:f=w242:i32)
            n133 = for {
              tunnel: w245 -> [w250] mode=indexing
              tunnel: w242 -> [w249]
              shift-right: [w248] -> w241
              shift-left: w246 -> [w251]
              n134 = in-place {
                in-place-border: w249 -> [w252]
                n135 = in-place-array #1(w251, w250) -> ()  [unwired: 1 out]
                n136 = in-place-array #1(w252) -> (w248:i32[])  [unwired: 1 out]
              }
            }
            n137 = Not(x=w238) -> (.not. x?=w235:bool)
            n138 = property on="GOOP3 classes found" class="LstBox (strict)"("Item Symbols"=w241) -> ()  [unwired: 2 in, 2 out]
            n139 = Select(t="Deselect (Space)", s=w235, f="Select (Space)") -> (s? t:f=w234:string)
            n140 = Build Array(w234) -> (w233:string[])
            n141 = Bundle By Name(cluster=w240, "Deselect"=w235) -> (w239:T7)
            n142 = property on="Toggle" class="Bool"("Strings [4]"=w233) -> ()  [unwired: 2 in, 2 out]
          }
          event "GOOP3 classes found": Double Click {
            n143 = event-data() -> ("Row"=w254:i32)  [unwired: 1 in]
            n144 = Unbundle By Name(w262) -> ("Deselect"=w260:bool)
            n145 = Build Array(w254) -> (w253:i32[])
            n146 = property on="GOOP3 classes found" class="LstBox (strict)"() -> ("Item Symbols"=w267:i32[])  [unwired: 2 in, 2 out]
            n147 = Select(t=37, s=w260, f=38) -> (s? t:f=w264:i32)
            n148 = for {
              tunnel: w253 -> [w271] mode=indexing
              tunnel: w264 -> [w270]
              shift-right: [w269] -> w263
              shift-left: w267 -> [w272]
              n149 = in-place {
                in-place-border: w270 -> [w273]
                n150 = in-place-array #2(w272, w271) -> ()  [unwired: 1 out]
                n151 = in-place-array #2(w273) -> (w269:i32[])  [unwired: 1 out]
              }
            }
            n152 = Not(x=w260) -> (.not. x?=w257:bool)
            n153 = property on="GOOP3 classes found" class="LstBox (strict)"("Item Symbols"=w263) -> ()  [unwired: 2 in, 2 out]
            n154 = Select(t="Deselect (Space)", s=w257, f="Select (Space)") -> (s? t:f=w256:string)
            n155 = Build Array(w256) -> (w255:string[])
            n156 = Bundle By Name(cluster=w262, "Deselect"=w257) -> (w261:T7)
            n157 = property on="Toggle" class="Bool"("Strings [4]"=w255) -> ()  [unwired: 2 in, 2 out]
          }
          event Key Down? {
            n158 = event-data() -> ("Char"=w276:i16, "VKey"=w277:T19)  [unwired: 1 in, 8 out]
            n159 = local read "Tab"() -> (w279:T1)
            n160 = case shown="\"ClassesFound\"" w279 {
              tunnel: w275 -> [_ w287]
              tunnel: [_ w284] -> w278
              tunnel: w277 -> [_ w286]
              tunnel: w276 -> [_ w285]
              tunnel: w275 -> [w281 w283]
              tunnel: [w281 w282] -> w274
              frame Default {
              }
              frame "ClassesFound" {
                n161 = case shown="\"ASCII\"" w286 {
                  tunnel: w287 -> [_ w293]
                  tunnel: w285 -> [_ w292]
                  tunnel: [_ w291] -> w284
                  tunnel: w283 -> [w288 w290]
                  tunnel: [w288 w289] -> w282
                  frame Default {
                  }
                  frame "ASCII" {
                    n162 = case shown="32" w292 {
                      tunnel: w293 -> [_ w310]
                      tunnel: [_ TRUE] -> w291
                      tunnel: w290 -> [w294 w297]
                      tunnel: [w294 w296] -> w289
                      frame 0, Default {
                      }
                      frame 32 {
                        n163 = local read "GOOP3 classes found"() -> (w308:i32[])
                        n164 = Unbundle By Name(w310) -> ("Deselect"=w295:bool)
                        n165 = property on="GOOP3 classes found" class="LstBox (strict)"() -> ("Item Symbols"=w309:i32[])  [unwired: 2 in, 2 out]
                        n166 = Select(t=37, s=w295, f=38) -> (s? t:f=w305:i32)
                        n167 = for {
                          tunnel: w308 -> [w313] mode=indexing
                          tunnel: w305 -> [w312]
                          shift-right: [w311] -> w304
                          shift-left: w309 -> [w314]
                          n168 = in-place {
                            in-place-border: w312 -> [w315]
                            n169 = in-place-array #3(w314, w313) -> ()  [unwired: 1 out]
                            n170 = in-place-array #3(w315) -> (w311:i32[])  [unwired: 1 out]
                          }
                        }
                        n171 = Not(x=w295) -> (.not. x?=w300:bool)
                        n172 = property on="GOOP3 classes found" class="LstBox (strict)"("Item Symbols"=w304) -> ()  [unwired: 2 in, 2 out]
                        n173 = Select(t="Deselect (Space)", s=w300, f="Select (Space)") -> (s? t:f=w299:string)
                        n174 = Build Array(w299) -> (w298:string[])
                        n175 = Bundle By Name(cluster=w297, "Deselect"=w300) -> (w296:T7)
                        n176 = property on="Toggle" class="Bool"("Strings [4]"=w298) -> ()  [unwired: 2 in, 2 out]
                      }
                    }
                  }
                }
              }
            }
            n177 = event-data("Discard?"=w278) -> ()  [unwired: 6 in, 1 out]
          }
          event "ApplyPersistentPattern": Value Change {
            n178 = event-data() -> ()  [unwired: 1 in, 6 out]
            n179 = case shown="False" "ApplyPersistentPattern" {
              selector: "ApplyPersistentPattern" -> [w319 _]
              frame False {
                n180 = local write "ApplyDebuggingSupport"(w319) -> ()
              }
              frame True {
              }
            }
          }
          event "ApplyDebuggingSupport": Value Change {
            n181 = event-data() -> ()  [unwired: 1 in, 6 out]
            n182 = case shown="True" "ApplyDebuggingSupport" {
              selector: "ApplyDebuggingSupport" -> [_ w323]
              frame False {
              }
              frame True {
                n183 = local write "ApplyPersistentPattern"(w323) -> ()
              }
            }
          }
        }
      }
      frame "SearchForGoopKernels" {
        n184 = Unbundle By Name(w350) -> ("TopFolderPath"=w352:path, "SelectedClasses"=w333:i32[])
        n185 = stacked-sequence {
          tunnel: w348 -> [w358]
          tunnel: [w358] -> w347
          frame #0 {
            n186 = property on="GOOP3 classes found" class="LstBox (strict)"("Item Names"=string[] ["Searching..."]) -> ()  [unwired: 2 in, 2 out]
          }
        }
        n187 = call <vilib>:"Recursive File List.vi"("pattern"="*GOOPKernel.vi", "error in (no error)"=w347, "Treat LLBs as Folders?"=TRUE, "Folder Path"=w352) -> ("error out"=w328:errorcluster, "All Files in Dir"=w346:path[])  [unwired: 3 in, 3 out]
        n188 = Sort 1D Array(array=w346) -> (sorted array=w341:path[])
        n189 = Unbundle By Name(w328) -> ("status"=w330:bool)
        n190 = for {
          tunnel: w341 -> [w390] mode=indexing
          tunnel: w340 -> [w385]
          tunnel: [w376] -> w339 mode=indexing
          tunnel: [w367] -> w338 mode=indexing
          tunnel: w333 -> [w374]
          shift-right: [w364] -> w325
          shift-left: T2[] [] -> [w365]
          i -> [w375]
          n191 = Strip Path(path=w390) -> (stripped path=w387:path, name=w362:string)
          n192 = Match Pattern(string=w362, regular expression="-DeleteMe-") -> (offset past match=w360:i32)  [unwired: 1 in, 3 out]
          n193 = xnode "Match Regular Expression"("input string"=w362, "regular expression"="GOOPKernel.vi$", "ignore case? (F)"=TRUE) -> ("before match"=w384:string)  [unwired: 3 in, 4 out]
          n194 = Empty Array?(array=w374) -> (empty?=w371:bool)
          n195 = Search 1D Array(1D array=w374, element=w375) -> (index of element=w373:i32)  [unwired: 1 in]
          n196 = Strip Path(path=w387) -> (stripped path=w386:path)  [unwired: 1 out]
          n197 = call <vilib>:"Has LLB Extension.vi"("path"=w387) -> ("path to VI library?"=w383:bool)
          n198 = Less Than 0?(x=w360) -> (x < 0?=w359:bool)
          n199 = Not(x=w371) -> (.not. x?=w366:bool)
          n200 = Less Than 0?(x=w373) -> (x < 0?=w372:bool)
          n201 = Match Pattern(string=w384, regular expression="[_\\s]$") -> (before substring=w376:string)  [unwired: 1 in, 3 out]
          n202 = Select(t=w387, s=w383, f=w386) -> (s? t:f=w379:path)
          n203 = And(x=w366, y=w372) -> (x .and. y?=w370:bool)
          n204 = List Folder(path=w379, pattern="*.lvclass") -> (filenames=w380:string[])  [unwired: 2 in, 3 out]
          n205 = Select(t=37, s=w370, f=38) -> (s? t:f=w367:i32)
          n206 = Index Array(array=w380) -> (element=w378:string)  [unwired: 1 in]
          n207 = Build Path(base path=w379, name or relative path=w378) -> (appended path=w377:path)
          n208 = Bundle By Name(cluster=w385, "LvClassPath"=w377, "ClassName"=w376, "ClassPrefix"=w384, "IsLLB"=w383, "ClassFolder"=w379) -> (w363:T2)
          n209 = case shown="True" w359 {
            tunnel: w365 -> [w391 w394]
            tunnel: [w391 w393] -> w364
            tunnel: w363 -> [_ w392]
            frame False {
            }
            frame True {
              n210 = Build Array (concatenate)(w394, w392) -> (w393:T2[])
            }
          }
        }
        n211 = Empty Array?(array=w341) -> (empty?=w331:bool)
        n212 = Or(x=w331, y=w330) -> (x .or. y?=w329:bool)
        n213 = Select(t=u8 2, s=w331, f=u8 0 ("Disabled")) -> (s? t:f=w342:u8)
        n214 = case shown="True" w329 {
          tunnel: [w354 _] -> w332
          tunnel: w328 -> [w354 _]
          tunnel: ["Idle" "Init"] -> w327
          frame False {
          }
          frame True {
            n215 = One Button Dialog(message="No classes found in that folder") -> ()  [unwired: 1 in, 1 out]
          }
        }
        n216 = property on="Next" class="Bool"("Disabled"=w342) -> ()  [unwired: 2 in, 2 out]
        n217 = Bundle By Name(cluster=w350, "Classes"=w325) -> (w349:T7)
        n218 = Build Array("Select one or more classes") -> (w335:string[])
        n219 = property on="GOOP3 classes found" class="LstBox (strict)"("Item Names"=w339, "Item Symbols"=w338, "Value"=i32[] [] ("GOOP3 classes found"), "Top Row"=0) -> ()  [unwired: 2 in, 2 out]
        n220 = property on="Toggle" class="Bool"("DisabledEnum"=T8."Disabled and Grayed Out" ("Disabled"), "Strings [4]"=w335) -> ()  [unwired: 2 in, 2 out]
      }
      frame "------ CONVERSION START -------" {
      }
      frame "CreateProject" {
        n221 = Unbundle By Name(w532) -> ("Project"=w523:path)
        n222 = Open Application Reference(8:w520) -> (0:w519:errorcluster, 3:w521:refnum<vi>)  [unwired: 3 in]
        n223 = call <vilib>:"Check if File or Folder Exists.vi"("path"=w523) -> ("file or folder exists?"=w522:bool)  [unwired: 8 in, 2 out]
        n224 = case shown="True" w522 {
          tunnel: [w539 w545] -> w529
          tunnel: [w538 w543] -> w528
          tunnel: [w537 w544] -> w524
          tunnel: w523 -> [w536 w547]
          tunnel: w521 -> [w535 w548]
          tunnel: w519 -> [w534 w546]
          tunnel: ["Creating New Project" "Open Existing Project"] -> w515
          frame False {
            n225 = invoke class="App" method="Project.New"(reference=w535, error in=w534) -> (reference out=w537:refnum<vi>, error out=w540:errorcluster, "Project:New"=w541:refnum<vi>)  [unwired: 1 in]
            n226 = invoke class="Project" method="Save"(reference=w541, error in=w540, "Path"=w536) -> (reference out=w538:refnum<vi>, error out=w539:errorcluster)  [unwired: 1 in, 2 out]
          }
          frame True {
            n227 = invoke class="App" method="Project.Open"(reference=w548, error in=w546, "Path"=w547) -> (reference out=w544:refnum<vi>, error out=w545:errorcluster, "Project:Open"=w543:refnum<vi>)  [unwired: 1 in, 1 out]
          }
        }
        n228 = control-ref of="Progress"() -> (w516:refnum<vi>)
        n229 = property class="Project"(reference=w528, error in=w529) -> (reference out=w527:refnum<vi>, error out=w526:errorcluster, "App Ref"=w514:refnum<vi>)
        n230 = call <resource>:"ConvertGoop3ToGoop4_UpdateProgressList.vi"("String"=w515, "Progress"=w516) -> ()  [unwired: 9 in, 1 out]
        n231 = Enqueue Element(queue=w511, element=TRUE) -> ()  [unwired: 2 in, 3 out]
        n232 = property class="App"(reference=w514) -> ("App.AllVIs"=w513:string[])  [unwired: 1 in, 2 out]
        n233 = property class="Project"(reference=w527, error in=w526) -> (error out=w518:errorcluster, "My Computer"=w525:refnum<vi>)  [unwired: 1 out]
        n234 = Array Size(array=w513) -> (size(s)=w512:i32)
        n235 = Bundle By Name(cluster=w532, "Log"=TRUE, "ProjectRef"=w527, "AppRef"=w514, "My Computer"=w525) -> (w531:T7)
        n236 = Close Reference(reference=w524, error in (no error)=w518) -> (error out=w517:errorcluster)
      }
      frame "AddClassesToProject" {
        w562 = TRUE ("ExcludeTargets")
        n237 = Unbundle By Name(w561) -> ("My Computer"=w555:refnum<vi>, "AppRef"=w549:refnum<vi>)
        n238 = Unbundle By Name(w561) -> ("Classes"=w560:T2[])
        n239 = invoke class="TargetItem" method="Get All Descendents"(reference=w555, error in=w557, "Type"="lvclass", "ExcludeBuilds"=w562, "ExcludeTargets"=w562) -> (error out=w558:errorcluster, "All Descendents"=w551:refnum<vi>[])  [unwired: 2 in, 5 out]
        n240 = for {
          tunnel: w551 -> [w575] mode=indexing
          tunnel: [w574] -> w559 mode=indexing
          shift-right: [w572] -> w556
          shift-left: w558 -> [w573]
          n241 = property class="ProjectItem"(reference=w575, error in=w573) -> (error out=w572:errorcluster, "Path"=w574:path)  [unwired: 1 out]
        }
        n242 = for {
          tunnel: w560 -> [w583] mode=indexing
          tunnel: w559 -> [w589]
          shift-right: [w580] -> w554
          shift-left: w556 -> [w587]
          tunnel: w555 -> [w586]
          tunnel: w551 -> [w584]
          tunnel: [w578] -> w553 mode=indexing
          tunnel: [w577] -> w550 mode=indexing
          tunnel: w549 -> [w576]
          n243 = Unbundle By Name(w583) -> ("LvClassPath"=w585:path)
          n244 = Search 1D Array(1D array=w589, element=w585) -> (index of element=w588:i32)  [unwired: 1 in]
          n245 = case shown="-1" w588 {
            selector: w588 -> [w591 _]
            tunnel: w587 -> [w593 w601]
            tunnel: [w593 w600] -> w582
            tunnel: w586 -> [_ w602]
            tunnel: w585 -> [_ w598]
            tunnel: w584 -> [w592 _]
            tunnel: [w590 w597] -> w579
            tunnel: w576 -> [_ w599]
            frame 0, Default {
              n246 = Index Array(array=w592, index=w591) -> (element=w590:refnum<vi>)
            }
            frame -1 {
              n247 = invoke class="TargetItem" method="AddFile"(reference=w602, error in=w601, "Path"=w598) -> (error out=w595:errorcluster, "AddFile"=w596:refnum<vi>)  [unwired: 1 in, 2 out]
              n248 = call <resource>:"CommonVIs_Wait.vi"("error in"=w595) -> ("error out"=w594:errorcluster)  [unwired: 9 in]
              n249 = case shown="No Error" w594 {
                selector: w594 -> [w604 _]
                tunnel: w601 -> [_ w609]
                tunnel: [w604 w605] -> w600
                tunnel: w599 -> [_ w608]
                tunnel: w598 -> [_ w607]
                tunnel: [w603 w606] -> w597
                tunnel: w596 -> [w603 _]
                frame No Error {
                }
                frame Error {
                  n250 = invoke class="App" method="LVClass.Open"(reference=w608, error in=w609, "Path"=w607) -> (error out=w605:errorcluster, "LVClass.Open"=w606:refnum<vi>)  [unwired: 1 in, 2 out]
                }
              }
            }
          }
          n251 = To More Specific Class(target class=refnum<vi> refnum ("ClassRef"), reference=w579, error in=w582) -> (specific class reference=w577:refnum<vi>, error out=w580:errorcluster)
          n252 = Bundle By Name(cluster=w583, "ClassRef"=w577) -> (w578:T2)
        }
        n253 = for {
          tunnel: w551 -> [w568] mode=indexing
          tunnel: w550 -> [w570]
          n254 = To More Specific Class(target class=refnum<vi> refnum ("ClassRef"), reference=w568) -> (specific class reference=w566:refnum<vi>)  [unwired: 1 in, 1 out]
          n255 = Search 1D Array(1D array=w570, element=w566) -> (index of element=w567:i32)  [unwired: 1 in]
          n256 = case shown="-1" w567 {
            tunnel: w566 -> [_ w571]
            frame Default {
            }
            frame -1 {
              n257 = Close Reference(reference=w571) -> ()  [unwired: 1 in, 1 out]
            }
          }
        }
        n258 = call <resource>:"ConvertGoop3ToGoop4_UpdateProgressList.vi"("String"="Adding classes to project if needed") -> ()  [unwired: 10 in, 1 out]
        n259 = Bundle By Name(cluster=w561, "Classes"=w553) -> (w565:T7)
      }
      frame "AnalyseClasses" {
        (unwired) "Base_GetObjectStatus.vi" ("Type")
        n260 = Unbundle By Name(w623) -> ("Classes"=w624:T2[])
        n261 = call <resource>:"ConvertGoop3ToGoop4_UpdateProgressList.vi"("String"="Analysing classes") -> ("error out"=w610:errorcluster)  [unwired: 10 in]
        n262 = for {
          tunnel: w624 -> [w642] mode=indexing
          tunnel: string[] ["GetObjectStatus.vi$"] ("file names") -> [w647]
          tunnel: string[] ["GetClassAttributes.vi$", "GetClassAttributesToModify.vi$", "SetModifiedClassAttributes.vi$"] ("file names") -> [w644]
          tunnel: [w640] -> w617 mode=indexing
          tunnel: [w626] -> w615 mode=indexing
          tunnel: w610 -> [_]
          n263 = Unbundle By Name(w642) -> ("ClassRef"=w639:refnum<vi>)
          n264 = property class="LVClassLibrary"(reference=w639) -> (reference out=w625:refnum<vi>, "Name"=w645:string)  [unwired: 1 in, 1 out]
          n265 = invoke class="LVClassLibrary" method="Get All Descendents"(reference=w639, "Type"="VI") -> ("All Descendents"=w648:refnum<vi>[])  [unwired: 5 in, 6 out]
          n266 = call <resource>:"GDSLvClass_ReadClassType.vi"("Class Refnum In"=w639) -> ("ClassSettings"=w633:T3)  [unwired: 16 in, 2 out]
          n267 = call <resource>:"GDSLvIcon_AnalyseViIcon.vi"("ViRef/LvCLassRef/LvLibRef/ViPath/2D_Image"=w639) -> ("HeaderIcon"=w638:u8[][])  [unwired: 6 in, 12 out]
          n268 = while {
            shift-right: [w652] -> w637
            shift-left: w625 -> [w658]
            shift-right: [w653] -> w635
            shift-left: path[] [] -> [w655]
            i -> [w650]
            stop <- w656 stop-if-true
            n269 = property class="LVClassLibrary"(reference=w658) -> (reference out=w651:refnum<vi>, error out=w657:errorcluster, "Parent"=w652:refnum<vi>)  [unwired: 1 in]
            n270 = case shown="1.." w650 {
              tunnel: w651 -> [_ w659]
              frame Default {
              }
              frame 1.. {
                n271 = Close Reference(reference=w659) -> ()  [unwired: 1 in, 1 out]
              }
            }
            n272 = property class="LVClassLibrary"(reference=w652, error in=w657) -> (error out=w656:errorcluster, "Path"=w654:path)  [unwired: 1 out]
            n273 = case shown="No Error" w656 {
              tunnel: w655 -> [w662 w663]
              tunnel: w654 -> [w661 _]
              tunnel: [w660 w663] -> w653
              frame No Error {
                n274 = Build Array (concatenate)(w662, w661) -> (w660:path[])
              }
              frame Error {
              }
            }
          }
          n275 = Close Reference(reference=w637) -> ()  [unwired: 1 in, 1 out]
          n276 = String Length(string=w645) -> (length=w646:i32)
          n277 = for {
            tunnel: w648 -> [w667] mode=indexing
            tunnel: w647 -> [w673]
            tunnel: w646 -> [w671]
            tunnel: w645 -> [w670]
            tunnel: w644 -> [w669]
            tunnel: [w668] -> w643 mode=indexing
            shift-right: [w666] -> w627
            shift-left: string[] [] -> [w665]
            n278 = property class="ProjectItem"(reference=w667) -> (reference out=w664:refnum<vi>, "Reference"=w676:refnum<vi>, "Name"=w674:string)  [unwired: 1 in, 1 out]
            n279 = for {
              tunnel: w674 -> [w712]
              tunnel: w673 -> [w711] mode=indexing
              tunnel: [w709] -> w675 mode=indexing
              n280 = Match Pattern(string=w712, regular expression=w711) -> (offset past match=w710:i32)  [unwired: 1 in, 3 out]
              n281 = Greater Or Equal To 0?(x=w710) -> (x >= 0?=w709:bool)
            }
            n282 = Or Array Elements(Boolean array=w675) -> (logical OR=w672:bool)
            n283 = Close Reference(reference=w664) -> ()  [unwired: 1 in, 1 out]
            n284 = case shown="False" w672 {
              tunnel: w676 -> [w689 w708]
              tunnel: w671 -> [w687 _]
              tunnel: w670 -> [w686 _]
              tunnel: w669 -> [w685 _]
              tunnel: [w683 _] -> w668
              tunnel: [w678 w707] -> w666
              tunnel: w665 -> [w677 w707]
              frame False {
                n285 = invoke class="VI" method="Get VI Dependencies"(reference=w689, "Include Standard VIs?"=TRUE) -> (reference out=w682:refnum<vi>, "Dependency Names"=w688:string[])  [unwired: 17 in, 17 out]
                n286 = for {
                  tunnel: w688 -> [w698] mode=indexing
                  tunnel: w687 -> [w701]
                  tunnel: w686 -> [w699]
                  tunnel: w685 -> [w697]
                  tunnel: [w694] -> w683
                  stop <- w694 stop-if-true
                  n287 = for {
                    tunnel: w698 -> [w706]
                    tunnel: w697 -> [w705] mode=indexing
                    tunnel: [w703] -> w696
                    stop <- w703 stop-if-true
                    n288 = Match Pattern(string=w706, regular expression=w705) -> (offset past match=w704:i32)  [unwired: 1 in, 3 out]
                    n289 = Greater Or Equal To 0?(x=w704) -> (x >= 0?=w703:bool)
                  }
                  n290 = String Subset(string=w698, length (rest)=w701) -> (substring=w700:string)  [unwired: 1 in]
                  n291 = Equal?(x=w699, y=w700) -> (x = y?=w695:bool)
                  n292 = case shown="True" w695 {
                    tunnel: w696 -> [_ w702]
                    tunnel: [_ w702] -> w694
                    frame False {
                    }
                    frame True {
                    }
                  }
                }
                n293 = property class="VI"(reference=w682) -> (reference out=w681:refnum<vi>, "Exec.State"=w680:T20, "Name"=w679:string)  [unwired: 1 in, 1 out]
                n294 = case shown="\"Bad\"" w680 {
                  tunnel: w679 -> [w692 _]
                  tunnel: [w691 w693] -> w678
                  tunnel: w677 -> [w690 w693]
                  frame "Bad" {
                    n295 = Build Array (concatenate)(w690, w692) -> (w691:string[])
                  }
                  frame "Idle", Default {
                  }
                }
                n296 = Close Reference(reference=w681) -> ()  [unwired: 1 in, 1 out]
              }
              frame True {
                n297 = Close Reference(reference=w708) -> ()  [unwired: 1 in, 1 out]
              }
            }
          }
          n298 = Unbundle By Name(w633) -> ("ClassTemplateUsed"=w632:string)
          n299 = Match Pattern(string=w632, regular expression="Singleton") -> (offset past match=w630:i32)  [unwired: 1 in, 3 out]
          n300 = Greater Or Equal To 0?(x=w630) -> (x >= 0?=w629:bool)
          n301 = Array Size(array=w635) -> (size(s)=w634:i32)
          n302 = Or Array Elements(Boolean array=w643) -> (logical OR=w641:bool)
          n303 = Bundle By Name(cluster=w642, "NoOfInheritance"=w634, "AllInheritanceClasses"=w635, "HeaderIcon"=w638, "ClassSettings"=w633, "Singleton"=w629, "UsingClassAttributes"=w641, "BrokenVIs"=w627) -> (w640:T2)
          n304 = Empty Array?(array=w627) -> (empty?=w626:bool)
        }
        n305 = Sort 1D Array(array=w617) -> (sorted array=w616:T2[])
        n306 = And Array Elements(Boolean array=w615) -> (logical AND=w614:bool)
        n307 = Select(t="UpdateClassAttributeClasses", s=w614, f="WarnAboutBrokenVIs") -> (s? t:f=w612:string)
        n308 = Bundle By Name(cluster=w623, "Classes"=w616) -> (w622:T7)
      }
      frame "WarnAboutBrokenVIs" {
        n309 = Unbundle By Name(w713) -> ("Classes"=w720:T2[])
        n310 = for {
          tunnel: w720 -> [w755] mode=indexing
          shift-right: [w753] -> w716
          shift-left: string[] [] -> [w752]
          n311 = Unbundle By Name(w755) -> ("BrokenVIs"=w754:string[])
          n312 = Build Array (concatenate)(w752, w754) -> (w753:string[])
        }
        n313 = call <vilib>:"Three Button Dialog.vi"("Right Button Text (\"Cancel\")"="Continue anyway" ("Right Button Text (\"Cancel\")"), "Center Button Text (\"No\")"="View Broken VIs" ("Center Button Text (\"No\")"), "Left Button Text (\"Yes\")"="Quit" ("Left Button Text (\"Yes\")"), "message"="There are VIs that are \"broken\".\nIt's recommended that you fix these VIs so no all VIs are \"broken\". This help determin if the conversion worked or not.") -> ("Which Button?"=w718:T21)  [unwired: 7 in]
        n314 = Unbundle By Name(w713) -> ("AppRef"=w715:refnum<vi>)
        n315 = case shown="\"Center Button\"" w718 {
          tunnel: ["Exit" "UpdateClassAttributeClasses" w730] -> w717
          tunnel: w716 -> [_ _ w728]
          tunnel: w715 -> [_ _ w729]
          tunnel: w713 -> [_ _ w727]
          frame "Left Button", Default {
          }
          frame "Right Button" {
          }
          frame "Center Button" {
            n316 = Array To Spreadsheet String(delimiter (Tab)="\n", array=w728, 3:"%s" ("format string")) -> (spreadsheet string=w732:string)
            n317 = call <vilib>:"Three Button Dialog.vi"("Right Button Text (\"Cancel\")"="Continue anyway" ("Right Button Text (\"Cancel\")"), "Center Button Text (\"No\")"="Open These VIs and Exit" ("Left Button Text (\"Yes\")"), "Left Button Text (\"Yes\")"="Quit" ("Left Button Text (\"Yes\")"), "message"=w732) -> ("Which Button?"=w731:T21)  [unwired: 7 in]
            n318 = case shown="\"Left Button\", Default" w731 {
              tunnel: ["Exit" "Exit" "UpdateClassAttributeClasses"] -> w730
              tunnel: w729 -> [_ w742 _]
              tunnel: w728 -> [_ w741 _]
              tunnel: w727 -> [_ w739 _]
              frame "Left Button", Default {
              }
              frame "Center Button" {
                n319 = for {
                  tunnel: w742 -> [w750]
                  tunnel: w741 -> [w749] mode=indexing
                  n320 = Open VI Reference(application reference (local)=w750, vi path=w749) -> (vi reference=w748:refnum<vi>, error out=w747:errorcluster)  [unwired: 4 in]
                  n321 = property class="VI"(reference=w748, error in=w747, "Front Panel.Open"=TRUE ("Front Panel Window:Open")) -> (reference out=w745:refnum<vi>, error out=w744:errorcluster)
                  n322 = Close Reference(reference=w745, error in (no error)=w744) -> ()  [unwired: 1 out]
                }
                n323 = Unbundle By Name(w739) -> ("ProjectRef"=w740:refnum<vi>)
                n324 = invoke class="Project" method="Open Window"(reference=w740) -> ()  [unwired: 2 in, 3 out]
              }
              frame "Right Button" {
              }
            }
          }
        }
      }
      frame "UpdateClassAttributeClasses" {
        n325 = Unbundle By Name(w762) -> ("Classes"=w759:T2[])
        n326 = for {
          tunnel: w759 -> [w768] mode=indexing
          shift-right: [w765] -> w757
          shift-left: path[] [] -> [w766]
          n327 = Unbundle By Name(w768) -> ("AllInheritanceClasses"=w764:path[], "UsingClassAttributes"=w767:bool)
          n328 = case shown="True" w767 {
            tunnel: w766 -> [w769 w772]
            tunnel: [w769 w771] -> w765
            tunnel: w764 -> [_ w770]
            frame False {
            }
            frame True {
              n329 = Build Array (concatenate)(w772, w770) -> (w771:path[])
            }
          }
        }
        n330 = for {
          tunnel: w759 -> [w780] mode=indexing
          tunnel: w757 -> [w778]
          tunnel: [w773] -> w761 mode=indexing
          n331 = Unbundle By Name(w780) -> ("LvClassPath"=w779:path, "UsingClassAttributes"=w775:bool)
          n332 = Search 1D Array(1D array=w778, element=w779) -> (index of element=w777:i32)  [unwired: 1 in]
          n333 = Greater Or Equal To 0?(x=w777) -> (x >= 0?=w776:bool)
          n334 = Or(x=w776, y=w775) -> (x .or. y?=w774:bool)
          n335 = Bundle By Name(cluster=w780, "UsingClassAttributes"=w774) -> (w773:T2)
        }
        n336 = Bundle By Name(cluster=w762, "Classes"=w761) -> (w760:T7)
      }
      frame "FindGetObjectStatus" {
        n337 = Unbundle By Name(w782) -> ("Classes"=w788:T2[])
        n338 = for {
          tunnel: w788 -> [w794] mode=indexing
          shift-right: [w796] -> w786
          shift-left: w787 -> [w797]
          tunnel: [w793] -> w783 mode=indexing
          n339 = Unbundle By Name(w794) -> ("ClassRef"=w798:refnum<vi>)
          n340 = invoke class="LVClassLibrary" method="Get All Descendents"(reference=w798, error in=w797, "Type"="VI") -> (error out=w795:errorcluster, "All Descendents"=w792:refnum<vi>[])  [unwired: 4 in, 5 out]
          n341 = for {
            tunnel: w792 -> [w811] mode=indexing
            shift-right: [w808] -> w796
            shift-left: w795 -> [w803]
            tunnel: [w803] -> w791
            shift-right: [w802] -> w789
            shift-left: FALSE -> [w800]
            n342 = property class="ProjectItem"(reference=w811, error in=w803) -> (error out=w809:errorcluster, "Reference"=w810:refnum<vi>, "Name"=w807:string)  [unwired: 1 out]
            n343 = Match Pattern(string=w807, regular expression="Destroy.vi$") -> (offset past match=w805:i32)  [unwired: 1 in, 3 out]
            n344 = Greater Or Equal To 0?(x=w805) -> (x >= 0?=w804:bool)
            n345 = case shown="False" w804 {
              tunnel: w810 -> [w819 w841]
              tunnel: w809 -> [w818 w842]
              tunnel: [w817 w842] -> w808
              tunnel: [w815 _] -> w801
              frame False {
                n346 = invoke class="VI" method="Get VI Dependencies"(reference=w819, error in=w818, "Include Standard VIs?"=TRUE) -> (reference out=w813:refnum<vi>, error out=w812:errorcluster, "Dependency Names"=w821:string[])  [unwired: 16 in, 16 out]
                n347 = for {
                  tunnel: w821 -> [w824] mode=indexing
                  tunnel: [w822] -> w814
                  tunnel: string[] ["GetObjectStatus.vi$"] -> [w823]
                  stop <- w822 stop-if-true
                  n348 = for {
                    tunnel: w824 -> [w827]
                    tunnel: w823 -> [w826] mode=indexing
                    tunnel: [w825] -> w822
                    stop <- w825 stop-if-true
                    n349 = Match Pattern(string=w827, regular expression=w826) -> (offset past match=w828:i32)  [unwired: 1 in, 3 out]
                    n350 = Greater Or Equal To 0?(x=w828) -> (x >= 0?=w825:bool)
                  }
                }
                n351 = case shown="True" w814 {
                  tunnel: w813 -> [w831 w834]
                  tunnel: [w830 w832] -> w817
                  tunnel: [_ w838] -> w815
                  tunnel: w812 -> [w829 w835]
                  frame False {
                    n352 = Close Reference(reference=w831, error in (no error)=w829) -> (error out=w830:errorcluster)
                  }
                  frame True {
                    n353 = call <resource>:"ConvertGoop3ToGoop4_Log.vi"("error in (no error)"=w835, "Object"=w834) -> ("error out"=w836:errorcluster)  [unwired: 7 in, 2 out]
                    n354 = call <resource>:"ConvertGoop3ToGoop4_UpdateGetObjectStatusCallers.vi"("error in (no error)"=w836, "RemoveWire"=TRUE, "ViRef"=w834) -> ("error out"=w840:errorcluster, "UsingObjectCallers"=w838:bool, "ViRefOut"=w839:refnum<vi>)  [unwired: 6 in]
                    n355 = Close Reference(reference=w839, error in (no error)=w840) -> (error out=w833:errorcluster)
                    n356 = call <resource>:"ConvertGoop3ToGoop4_ClearErrors.vi"("error in (no error)"=w833) -> ("error out"=w832:errorcluster)  [unwired: 9 in, 1 out]
                  }
                }
              }
              frame True {
                n357 = Close Reference(reference=w841) -> ()  [unwired: 1 in, 1 out]
              }
            }
            n358 = Or(x=w800, y=w801) -> (x .or. y?=w802:bool)
          }
          n359 = Close Reference(reference=w792, error in (no error)=w791) -> ()  [unwired: 1 out]
          n360 = Bundle By Name(cluster=w794, "ObjectStatusUsed"=w789) -> (w793:T2)
        }
        n361 = call <resource>:"ConvertGoop3ToGoop4_UpdateProgressList.vi"("String"="Find GetObjectStatus") -> ()  [unwired: 10 in, 1 out]
        n362 = Bundle By Name(cluster=w782, "Classes"=w783) -> (w781:T7)
      }
      frame "FindGetAttributes" {
        n363 = Unbundle By Name(w846) -> ("Classes"=w848:T2[])
        n364 = for {
          tunnel: w848 -> [w853] mode=indexing
          shift-right: [w851] -> w844
          shift-left: w845 -> [w850]
          n365 = Unbundle By Name(w853) -> ("ClassRef"=w852:refnum<vi>)
          n366 = invoke class="LVClassLibrary" method="Get All Descendents"(reference=w852, error in=w850, "Type"="VI") -> (error out=w849:errorcluster, "All Descendents"=w854:refnum<vi>[])  [unwired: 4 in, 5 out]
          n367 = for {
            tunnel: w854 -> [w865] mode=indexing
            shift-right: [w860] -> w851
            shift-left: w849 -> [w861]
            n368 = property class="ProjectItem"(reference=w865, error in=w861) -> (reference out=w864:refnum<vi>, error out=w862:errorcluster, "Reference"=w863:refnum<vi>, "Name"=w859:string)
            n369 = Match Pattern(string=w859, regular expression="GetObjectStatus.vi$") -> (offset past match=w857:i32)  [unwired: 1 in, 3 out]
            n370 = Greater Or Equal To 0?(x=w857) -> (x >= 0?=w856:bool)
            n371 = Close Reference(reference=w864) -> ()  [unwired: 1 in, 1 out]
            n372 = case shown="False" w856 {
              tunnel: w863 -> [w872 w894]
              tunnel: w862 -> [w871 w895]
              tunnel: [w870 w895] -> w860
              frame False {
                n373 = invoke class="VI" method="Get VI Dependencies"(reference=w872, error in=w871, "Include Standard VIs?"=TRUE) -> (reference out=w867:refnum<vi>, error out=w866:errorcluster, "Dependency Names"=w874:string[])  [unwired: 16 in, 16 out]
                n374 = for {
                  tunnel: w874 -> [w877] mode=indexing
                  tunnel: [w875] -> w869
                  tunnel: string[] ["GetAttributes\\2Evi$", "GetAttributesToModify\\2Evi$", "GetClassAttributes\\2Evi$", "GetClassAttributesToModify\\2Evi$"] -> [w876]
                  stop <- w875 stop-if-true
                  n375 = for {
                    tunnel: w877 -> [w880]
                    tunnel: w876 -> [w879] mode=indexing
                    tunnel: [w878] -> w875
                    stop <- w878 stop-if-true
                    n376 = Match Pattern(string=w880, regular expression=w879) -> (offset past match=w881:i32)  [unwired: 1 in, 3 out]
                    n377 = Greater Or Equal To 0?(x=w881) -> (x >= 0?=w878:bool)
                  }
                }
                n378 = case shown="True" w869 {
                  tunnel: w866 -> [w883 w889]
                  tunnel: w867 -> [w884 w887]
                  tunnel: [w882 w885] -> w870
                  frame False {
                    n379 = Close Reference(reference=w884, error in (no error)=w883) -> (error out=w882:errorcluster)
                  }
                  frame True {
                    n380 = call <resource>:"ConvertGoop3ToGoop4_Log.vi"("error in (no error)"=w889, "Object"=w887) -> ("error out"=w888:errorcluster)  [unwired: 7 in, 2 out]
                    n381 = call <resource>:"ConvertGoop3ToGoop4_InsertNodeAfterGetAttributes.vi"("error in (no error)"=w888, "ViRef"=w887) -> ("error out"=w892:errorcluster, "ViRefOut"=w893:refnum<vi>)  [unwired: 8 in]
                    n382 = invoke class="VI" method="Save.Instrument"(reference=w893, error in=w892) -> (reference out=w891:refnum<vi>, error out=w890:errorcluster)  [unwired: 4 in, 4 out]
                    n383 = Close Reference(reference=w891, error in (no error)=w890) -> (error out=w886:errorcluster)
                    n384 = call <resource>:"ConvertGoop3ToGoop4_ClearErrors.vi"("error in (no error)"=w886) -> ("error out"=w885:errorcluster)  [unwired: 9 in, 1 out]
                  }
                }
              }
              frame True {
                n385 = Close Reference(reference=w894) -> ()  [unwired: 1 in, 1 out]
              }
            }
          }
        }
        n386 = call <resource>:"ConvertGoop3ToGoop4_UpdateProgressList.vi"("String"="FindGetAttributeVIs") -> ()  [unwired: 10 in, 1 out]
      }
      frame "FindNewVIs" {
        n387 = Unbundle By Name(w899) -> ("Classes"=w901:T2[])
        n388 = for {
          tunnel: w901 -> [w906] mode=indexing
          shift-right: [w904] -> w897
          shift-left: w898 -> [w903]
          n389 = Unbundle By Name(w906) -> ("ClassRef"=w905:refnum<vi>)
          n390 = invoke class="LVClassLibrary" method="Get All Descendents"(reference=w905, error in=w903, "Type"="VI") -> (error out=w902:errorcluster, "All Descendents"=w907:refnum<vi>[])  [unwired: 4 in, 5 out]
          n391 = for {
            tunnel: w907 -> [w918] mode=indexing
            shift-right: [w913] -> w904
            shift-left: w902 -> [w914]
            n392 = property class="ProjectItem"(reference=w918, error in=w914) -> (reference out=w917:refnum<vi>, error out=w915:errorcluster, "Reference"=w916:refnum<vi>, "Name"=w912:string)
            n393 = Match Pattern(string=w912, regular expression="GetObjectStatus.vi$") -> (offset past match=w910:i32)  [unwired: 1 in, 3 out]
            n394 = Greater Or Equal To 0?(x=w910) -> (x >= 0?=w909:bool)
            n395 = Close Reference(reference=w917) -> ()  [unwired: 1 in, 1 out]
            n396 = case shown="False" w909 {
              tunnel: w916 -> [w925 w945]
              tunnel: w915 -> [w924 w946]
              tunnel: [w923 w946] -> w913
              frame False {
                n397 = invoke class="VI" method="Get VI Dependencies"(reference=w925, error in=w924, "Include Standard VIs?"=TRUE) -> (reference out=w920:refnum<vi>, error out=w919:errorcluster, "Dependency Names"=w927:string[])  [unwired: 16 in, 16 out]
                n398 = for {
                  tunnel: w927 -> [w930] mode=indexing
                  tunnel: "New\\2Evi$" -> [w929]
                  tunnel: [w928] -> w922
                  stop <- w928 stop-if-true
                  n399 = Match Pattern(string=w930, regular expression=w929) -> (offset past match=w931:i32)  [unwired: 1 in, 3 out]
                  n400 = Greater Or Equal To 0?(x=w931) -> (x >= 0?=w928:bool)
                }
                n401 = case shown="True" w922 {
                  tunnel: w919 -> [w933 w939]
                  tunnel: w920 -> [w934 w937]
                  tunnel: [w932 w935] -> w923
                  frame False {
                    n402 = Close Reference(reference=w934, error in (no error)=w933) -> (error out=w932:errorcluster)
                  }
                  frame True {
                    n403 = call <resource>:"ConvertGoop3ToGoop4_Log.vi"("error in (no error)"=w939, "Object"=w937) -> ("error out"=w938:errorcluster)  [unwired: 7 in, 2 out]
                    n404 = call <resource>:"ConvertGoop3ToGoop4_UpdateNewVICallers.vi"("error in (no error)"=w938, "InsertAlwaysCopy"=TRUE, "ViRef"=w937) -> ("error out"=w943:errorcluster, "ViRefOut"=w944:refnum<vi>)  [unwired: 7 in]
                    n405 = invoke class="VI" method="Save.Instrument"(reference=w944, error in=w943) -> (reference out=w942:refnum<vi>, error out=w941:errorcluster)  [unwired: 4 in, 4 out]
                    n406 = Close Reference(reference=w942, error in (no error)=w941) -> (error out=w936:errorcluster)
                    n407 = call <resource>:"ConvertGoop3ToGoop4_ClearErrors.vi"("error in (no error)"=w936) -> ("error out"=w935:errorcluster)  [unwired: 9 in, 1 out]
                  }
                }
              }
              frame True {
                n408 = Close Reference(reference=w945) -> ()  [unwired: 1 in, 1 out]
              }
            }
          }
        }
        n409 = call <resource>:"ConvertGoop3ToGoop4_UpdateProgressList.vi"("String"="Find New VIs") -> ()  [unwired: 10 in, 1 out]
      }
      frame "RenameVIsIfNeeded" {
        n410 = Unbundle By Name(w949) -> ("Classes"=w955:T2[])
        n411 = call <resource>:"ConvertGoop3ToGoop4_UpdateProgressList.vi"("String"="Rename VIs if needed") -> ("error out"=w950:errorcluster)  [unwired: 10 in]
        n412 = for {
          tunnel: w955 -> [w959] mode=indexing
          shift-right: [w963] -> w953
          shift-left: w954 -> [w962]
          tunnel: w950 -> [_]
          tunnel: [w958] -> w947 mode=indexing
          n413 = Unbundle By Name(w959) -> ("ClassRef"=w960:refnum<vi>)
          n414 = invoke class="LVClassLibrary" method="Get All Descendents"(reference=w960, error in=w962, "Type"="VI") -> (error out=w961:errorcluster, "All Descendents"=w964:refnum<vi>[])  [unwired: 4 in, 5 out]
          n415 = for {
            tunnel: w964 -> [w981] mode=indexing
            shift-right: [w976] -> w963
            shift-left: w961 -> [w977]
            tunnel: w960 -> [w974]
            shift-right: [w966] -> w956
            shift-left: "" ("Name") -> [w967]
            n416 = property class="ProjectItem"(reference=w981, error in=w977) -> (reference out=w980:refnum<vi>, error out=w978:errorcluster, "Reference"=w979:refnum<vi>, "Path"=w975:path, "Name"=w968:string)
            n417 = for {
              tunnel: string[] ["Destroy.vi$", "CleanUp.vi$"] -> [w983] mode=indexing
              tunnel: [w982] -> w969
              tunnel: w968 -> [w984]
              stop <- w982 stop-if-true
              n418 = Match Pattern(string=w984, regular expression=w983) -> (offset past match=w985:i32)  [unwired: 1 in, 3 out]
              n419 = Greater Or Equal To 0?(x=w985) -> (x >= 0?=w982:bool)
            }
            n420 = for {
              tunnel: w968 -> [w993]
              tunnel: string[] ["ObjectAttributes.ctl$", "ClassAttributes.ctl$"] -> [w992] mode=indexing
              tunnel: [w987] -> w972
              tunnel: [w986] -> w971
              stop <- w987 stop-if-true
              n421 = Match Pattern(string=w993, regular expression=w992) -> (before substring=w989:string, match substring=w986:string, offset past match=w988:i32)  [unwired: 1 in, 1 out]
              n422 = Greater Or Equal To 0?(x=w988) -> (x >= 0?=w991:bool)
              n423 = Empty String/Path?(string/path=w989) -> (empty?=w990:bool)
              n424 = Compound Arithmetic op=AND(invert w990, w991) -> (w987:bool)
            }
            n425 = Close Reference(reference=w980) -> ()  [unwired: 1 in, 1 out]
            n426 = Select(t=w968, s=w969, f=w967) -> (s? t:f=w966:string)
            n427 = case shown="True" w972 {
              tunnel: w979 -> [w994 w1001]
              tunnel: w978 -> [w995 w1003]
              tunnel: [w995 w1006] -> w976
              tunnel: w975 -> [_ w996]
              tunnel: w974 -> [_ w998]
              tunnel: w971 -> [_ w1004]
              frame False {
                n428 = Close Reference(reference=w994) -> ()  [unwired: 1 in, 1 out]
              }
              frame True {
                n429 = Strip Path(path=w996) -> (stripped path=w1008:path)  [unwired: 1 out]
                n430 = call <resource>:"ConvertGoop3ToGoop4_Log.vi"("error in (no error)"=w1003, "Object"=w1001) -> ("error out"=w1002:errorcluster)  [unwired: 7 in, 2 out]
                n431 = Build Path(base path=w1008, name or relative path=w1004) -> (appended path=w1007:path)
                n432 = invoke class="VI" method="Save.Instrument"(reference=w1001, error in=w1002, "Path to saved file"=w1007) -> (reference out=w1009:refnum<vi>, error out=w1000:errorcluster)  [unwired: 3 in, 4 out]
                n433 = call <resource>:"CommonVIs_Wait.vi"("error in"=w1000) -> ("error out"=w1005:errorcluster)  [unwired: 9 in]
                n434 = Close Reference(reference=w1009, error in (no error)=w1005) -> (error out=w999:errorcluster)
                n435 = stacked-sequence {
                  tunnel: w999 -> [w1012]
                  tunnel: w998 -> [w1011]
                  tunnel: [w1011] -> w997
                  tunnel: w996 -> [w1010]
                  frame #0 {
                    n436 = Delete(path (use dialog)=w1010, error in=w1012) -> ()  [unwired: 3 in, 3 out]
                  }
                }
                n437 = invoke class="LVClassLibrary" method="Save"(reference=w997, error in=w999) -> (error out=w1006:errorcluster)  [unwired: 2 in, 3 out]
              }
            }
          }
          n438 = Bundle By Name(cluster=w959, "DestrotCleanUpViName"=w956) -> (w958:T2)
        }
        n439 = Bundle By Name(cluster=w949, "Classes"=w947) -> (w948:T7)
      }
      frame "SaveAndCloseProject" {
        n440 = Unbundle By Name(w1030) -> ("ProjectRef"=w1035:refnum<vi>, "AppRef"=w1020:refnum<vi>, "My Computer"=w1029:refnum<vi>, "Classes"=w1028:T2[])
        n441 = property class="App"(reference=w1020, error in=w1026) -> (error out=w1025:errorcluster, "App.AllVIs"=w1024:string[])  [unwired: 1 out]
        n442 = Array Size(array=w1024) -> (size(s)=w1023:i32)
        n443 = call <resource>:"ConvertGoop3ToGoop4_UpdateProgressList.vi"("String"="Save and close object") -> ("error out"=w1016:errorcluster)  [unwired: 10 in]
        n444 = for {
          tunnel: w1028 -> [w1042] mode=indexing
          tunnel: w1025 -> [w1037]
          tunnel: w1023 -> [_]
          tunnel: w1016 -> [_]
          tunnel: [w1038] -> w1015 mode=indexing
          tunnel: [w1037] -> w1014
          n445 = Unbundle By Name(w1042) -> ("ClassRef"=w1038:refnum<vi>)
          n446 = invoke class="LVClassLibrary" method="Get All Descendents"(reference=w1038, "Type"="VI") -> ("All Descendents"=w1039:refnum<vi>[])  [unwired: 5 in, 6 out]
          n447 = for {
            tunnel: w1039 -> [w1048] mode=indexing
            tunnel: [w1044] -> w1040
            n448 = property class="ProjectItem"(reference=w1048) -> (error out=w1046:errorcluster, "Reference"=w1047:refnum<vi>)  [unwired: 1 in, 1 out]
            n449 = invoke class="VI" method="Save.Instrument"(reference=w1047, error in=w1046) -> (reference out=w1043:refnum<vi>, error out=w1045:errorcluster)  [unwired: 4 in, 4 out]
            n450 = Close Reference(reference=w1043, error in (no error)=w1045) -> (error out=w1044:errorcluster)
          }
          n451 = Close Reference(reference=w1039, error in (no error)=w1040) -> ()  [unwired: 1 out]
        }
        n452 = Close Reference(reference=w1015, error in (no error)=w1014) -> (error out=w1013:errorcluster)
        n453 = Close Reference(reference=w1029, error in (no error)=w1013) -> (error out=w1027:errorcluster)
        n454 = invoke class="Project" method="Save"(reference=w1035, error in=w1027) -> (reference out=w1034:refnum<vi>, error out=w1033:errorcluster)  [unwired: 2 in, 2 out]
        n455 = Close Reference(reference=w1034, error in (no error)=w1033) -> (error out=w1032:errorcluster)
        n456 = stacked-sequence {
          tunnel: w1032 -> [w1049]
          tunnel: [w1049] -> w1021
          frame #0 {
            n457 = Wait (ms)(milliseconds to wait=u32 500) -> ()  [unwired: 1 out]
          }
        }
        n458 = property class="App"(reference=w1020, error in=w1021) -> (error out=w1018:errorcluster, "App.AllVIs"=w1022:string[])  [unwired: 1 out]
        n459 = Array Size(array=w1022) -> (size(s)=w1019:i32)
        n460 = stacked-sequence {
          tunnel: w1019 -> [_]
          frame #0 {
            n461 = Wait (ms)(milliseconds to wait=u32 500) -> ()  [unwired: 1 out]
          }
        }
      }
      frame "CreateGOOP4Classes" {
        (unwired) EndevoG4TemplateNames."G4BaseTemplate_Simple_4x4x4" ("TemplateNames")
        (unwired) EndevoTemplateNames."SubTemplate" ("TemplateNames")
        n462 = Unbundle By Name(w1069) -> ("Classes"=w1055:T2[], "AppRef"=w1060:refnum<vi>)
        n463 = Temporary Directory() -> (w1079:path)
        n464 = invoke class="App" method="Project.New"(reference=w1060, error in=w1059) -> (error out=w1072:errorcluster, "Project:New"=w1080:refnum<vi>)  [unwired: 1 in, 1 out]
        n465 = for {
          tunnel: w1055 -> [w1083] mode=indexing
          tunnel: [w1082] -> w1054 mode=indexing
          tunnel: [w1081] -> w1053 mode=indexing
          n466 = Unbundle By Name(w1083) -> ("ClassFolder"=w1081:path, "LvClassPath"=w1082:path)
        }
        n467 = Build Path(base path=w1079, name or relative path="G3G4_folder") -> (appended path=w1077:path)
        n468 = Delete(path (use dialog)=w1077, entire hierarchy (F)=TRUE) -> (deleted path=w1074:path)  [unwired: 3 in, 2 out]
        n469 = Create Folder(path (use dialog)=w1074, error in=w1072) -> (created path=w1056:path, error out=w1071:errorcluster)  [unwired: 1 in, 1 out]
        n470 = Build Path(base path=w1056, name or relative path="G3G4_Temp.lvproj") -> (appended path=w1066:path)
        n471 = invoke class="Project" method="Save"(reference=w1080, error in=w1071, "Path"=w1066) -> (reference out=w1064:refnum<vi>, error out=w1063:errorcluster)  [unwired: 1 in, 2 out]
        n472 = property class="Project"(reference=w1064, error in=w1063) -> (reference out=w1057:refnum<vi>, error out=w1062:errorcluster, "My Computer"=w1061:refnum<vi>)
        n473 = call <resource>:"ConvertGoop3ToGoop4_UpdateProgressList.vi"("String"="Create GOOP4 classes") -> ("error out"=w1051:errorcluster)  [unwired: 10 in]
        n474 = for {
          tunnel: T10 {"ClassName"="", "ClassFolder"=path "", "ClassDescription"="", "ClassTemplateOptions"="", "BaseClass(ProjectStringPath or LvClassFilePath)"=variant, "ExtraCreateParameters"=variant, "FolderSuffix"=""} ("CreateClassData") -> [w1122]
          tunnel: w1061 -> [w1121]
          tunnel: w1055 -> [w1120] mode=indexing
          shift-right: [w1091] -> w1058
          shift-left: w1062 -> [w1094]
          tunnel: w1056 -> [w1118]
          tunnel: [w1116] -> w1067 mode=indexing
          tunnel: [w1115] -> w1065 mode=indexing
          tunnel: w1056 -> [w1105]
          tunnel: w1054 -> [w1104]
          tunnel: w1053 -> [w1103]
          tunnel: w1051 -> [_]
          (unwired) T22 2 items=["4x4x4", "5x6x5", "6x8x6"] ("PatternIn")
          (unwired) T22 0 items=["4x4x4", "5x6x5", "6x8x6"] ("PatternIn")
          w1114 = refnum<class "ClassWriterGOOP400.lvclass"> refnum  # ClassWriterGOOP400.lvclass
          (unwired) 0 ("y")
          n475 = Unbundle By Name(w1120) -> ("ClassName"=w1112:string, "ClassFolder"=w1088:path, "ClassSettings.ClassTemplateUsed"=w1087:string, "HeaderIcon"=w1113:u8[][], "AllInheritanceClasses"=w1106:path[])
          n476 = Empty Array?(array=w1106) -> (empty?=w1107:bool)
          n477 = Match Pattern(string=w1087, regular expression="Singelton") -> (offset past match=w1085:i32)  [unwired: 1 in, 3 out]
          n478 = call <resource>:"BaseProvider_ConfigurationMemory.vi"("error in (no error)"=w1094, "Action"=enum16{"Read", "Load", "Save", "Set"}."Read") -> ("PatternOut"=w1099:T22, "WireConfigurationOut"=w1095:T23, "IconOut"=w1096:string, "error out"=w1097:errorcluster)  [unwired: 11 in, 3 out]
          n479 = Format Into String(format string="Creating Copy Class: %s", w1112) -> (resulting string=w1102:string)  [unwired: 2 in, 1 out]
          n480 = Strip Path(path=w1088) -> (name=w1119:string)  [unwired: 1 out]
          n481 = call <resource>:"ConvertGoop3ToGoop4_UpdateProgressList.vi"("String"=w1102) -> ("error out"=w1084:errorcluster)  [unwired: 10 in]
          n482 = case shown="-1" w1085 {
            tunnel: [EndevoG4TemplateNames."G4BaseTemplate_Singleton_6x8x6" ("TemplateNames") w1128] -> w1110
            tunnel: [w1125 w1127] -> w1090
            tunnel: w1087 -> [_ w1126]
            tunnel: w1084 -> [_ _]
            frame 0, Default {
              w1125 = T22 2 items=["4x4x4", "5x6x5", "6x8x6"] ("PatternIn")
            }
            frame -1 {
              n483 = Scan From String(input string=w1126, default 1=EndevoTemplateNames."BaseTemplate" ("TemplateNames")) -> (output 1=w1129:T12)  [unwired: 3 in, 3 out]
              n484 = case shown="\"SingletonTemplate\"" w1129 {
                tunnel: [EndevoG4TemplateNames."G4BaseTemplate_Simple_6x8x6" ("TemplateNames") EndevoG4TemplateNames."G4BaseTemplate_Singleton_6x8x6" ("TemplateNames") EndevoG4TemplateNames."G4SubTemplate_Simple_6x8x6" ("TemplateNames") EndevoG4TemplateNames."G4BaseTemplate_Simple_4x4x4" ("TemplateNames") EndevoG4TemplateNames."G4SubTemplate_Simple_4x4x4" ("TemplateNames")] -> w1128
                tunnel: [w1131 w1133 w1135 w1137 w1139] -> w1127
                frame "BaseTemplate", Default {
                  w1131 = T22 2 items=["4x4x4", "5x6x5", "6x8x6"] ("PatternIn")
                }
                frame "SingletonTemplate" {
                  w1133 = T22 2 items=["4x4x4", "5x6x5", "6x8x6"] ("PatternIn")
                }
                frame "SubTemplate" {
                  w1135 = T22 2 items=["4x4x4", "5x6x5", "6x8x6"] ("PatternIn")
                }
                frame "BaseTemplate_4x4x4" {
                  w1137 = T22 0 items=["4x4x4", "5x6x5", "6x8x6"] ("PatternIn")
                }
                frame "SubTemplate_4x4x4" {
                  w1139 = T22 0 items=["4x4x4", "5x6x5", "6x8x6"] ("PatternIn")
                }
              }
            }
          }
          n485 = call <resource>:"BaseProvider_ConfigurationMemory.vi"("WireConfiguration"=w1095, "Icon"=w1096, "error in (no error)"=w1097, "Action"=enum16{"Read", "Load", "Save", "Set"}."Set", "PatternIn"=w1090) -> ("error out"=w1093:errorcluster)  [unwired: 8 in, 6 out]
          n486 = Format Into String(w1110) -> (resulting string=w1101:string)  [unwired: 3 in, 1 out]
          n487 = Build Path(base path=w1118, name or relative path=w1119) -> (appended path=w1111:path)
          n488 = Bundle By Name(cluster=w1122, "ClassName"=w1112, "ClassFolder"=w1111, "ClassTemplateOptions"=w1101) -> (w1109:T10)
          n489 = case shown="True" w1107 {
            tunnel: w1109 -> [w1151 w1152]
            tunnel: [w1150 w1152] -> w1108
            tunnel: w1106 -> [w1149 _]
            tunnel: w1105 -> [w1148 _]
            tunnel: w1104 -> [w1147 _]
            tunnel: w1103 -> [w1145 _]
            frame False {
              n490 = Index Array(array=w1149) -> (element=w1146:path)  [unwired: 1 in]
              n491 = Search 1D Array(1D array=w1147, element=w1146) -> (index of element=w1144:i32)  [unwired: 1 in]
              n492 = Index Array(array=w1145, index=w1144) -> (element=w1143:path)
              n493 = Strip Path(path=w1143) -> (name=w1142:string)  [unwired: 1 out]
              n494 = Build Path(base path=w1148, name or relative path=w1142) -> (appended path=w1141:path)
              n495 = Bundle By Name(cluster=w1151, "BaseClass(ProjectStringPath or LvClassFilePath)"=w1141) -> (w1150:T10)
            }
            frame True {
            }
          }
          n496 = call-dynamic "CreateClass.vi"("ClassWriterGOOP400.lvclass"=w1114, "ProjectTreePosition(String or Project Item Ref)"=w1121, "CreateClassData"=w1108, "error in (no error)"=w1093, "KeepLvClassRefOpen(False)"=TRUE, "HeaderToApply (take from VIRef or /use 2D-8bit header, Ignored if not wired)"=w1113) -> ("LVClassLibraryRefnum"=w1115:refnum<vi>, "TemplateVersionUsed"=w1116:string, "error out"=w1092:errorcluster)  [unwired: 10 in, 1 out]
          n497 = call <resource>:"BaseProvider_ConfigurationMemory.vi"("WireConfiguration"=w1095, "Icon"=w1096, "error in (no error)"=w1092, "Action"=enum16{"Read", "Load", "Save", "Set"}."Set", "PatternIn"=w1099) -> ("error out"=w1091:errorcluster)  [unwired: 8 in, 6 out]
        }
        n498 = Bundle By Name(cluster=w1069, "CopyClasses"=w1056, "CopyClassesRef"=w1065, "TemplateVersions"=w1067, "ProjectRef"=w1057) -> (w1068:T7)
        n499 = Close Reference(reference=w1061, error in (no error)=w1058) -> ()  [unwired: 1 out]
      }
      frame "RenameDestory" {
        (unwired) EndevoG4TemplateNames."G4BaseTemplate_Simple_4x4x4" ("TemplateNames")
        (unwired) EndevoTemplateNames."SubTemplate" ("TemplateNames")
        n500 = Unbundle By Name(w1155) -> ("Classes"=w1159:T2[], "CopyClassesRef"=w1153:refnum<vi>[])
        n501 = call <resource>:"ConvertGoop3ToGoop4_UpdateProgressList.vi"("String"="Rename Class Clone Destroy?") -> ("error out"=w1157:errorcluster)  [unwired: 10 in]
        n502 = for {
          tunnel: T10 {"ClassName"="", "ClassFolder"=path "", "ClassDescription"="", "ClassTemplateOptions"="", "BaseClass(ProjectStringPath or LvClassFilePath)"=variant, "ExtraCreateParameters"=variant, "FolderSuffix"=""} ("CreateClassData") -> [_]
          tunnel: w1159 -> [w1170] mode=indexing
          shift-right: [w1168] -> w1160
          shift-left: w1154 -> [w1164]
          tunnel: w1157 -> [_]
          tunnel: w1153 -> [w1169] mode=indexing
          n503 = Unbundle By Name(w1170) -> ("DestrotCleanUpViName"=w1162:string)  [unwired: 1 out]
          n504 = for {
            tunnel: string[] ["Destroy.vi$", "CleanUp.vi$"] -> [w1174] mode=indexing
            tunnel: [w1173] -> w1167
            tunnel: [w1171] -> w1166
            tunnel: w1162 -> [w1175]
            stop <- w1173 stop-if-true
            n505 = Match Pattern(string=w1175, regular expression=w1174) -> (before substring=w1172:string, offset past match=w1176:i32)  [unwired: 1 in, 2 out]
            n506 = Greater Or Equal To 0?(x=w1176) -> (x >= 0?=w1173:bool)
            n507 = Empty String/Path?(string/path=w1172) -> (empty?=w1171:bool)
          }
          n508 = Compound Arithmetic op=AND(w1167, invert w1166) -> (w1163:bool)
          n509 = case shown="True" w1163 {
            tunnel: w1164 -> [w1177 w1190]
            tunnel: w1169 -> [_ w1180]
            tunnel: w1162 -> [_ w1181]
            tunnel: [w1177 w1178] -> w1168
            frame False {
            }
            frame True {
              n510 = invoke class="LVClassLibrary" method="Get All Descendents"(reference=w1180, error in=w1190) -> (error out=w1188:errorcluster, "All Descendents"=w1182:refnum<vi>[])  [unwired: 5 in, 5 out]
              n511 = for {
                tunnel: w1182 -> [w1212] mode=indexing
                shift-right: [w1210] -> w1184
                shift-left: w1188 -> [w1211]
                tunnel: [w1208] -> w1187
                tunnel: [w1207] -> w1186
                tunnel: [w1206] -> w1183
                stop <- w1207 stop-if-true
                n512 = property class="ProjectItem"(reference=w1212, error in=w1211) -> (reference out=w1206:refnum<vi>, error out=w1210:errorcluster, "Name"=w1208:string)
                n513 = for {
                  tunnel: string[] ["Destroy.vi$", "CleanUp.vi$"] -> [w1214] mode=indexing
                  tunnel: [w1213] -> w1207
                  tunnel: w1208 -> [w1215]
                  stop <- w1213 stop-if-true
                  n514 = Match Pattern(string=w1215, regular expression=w1214) -> (offset past match=w1216:i32)  [unwired: 1 in, 3 out]
                  n515 = Greater Or Equal To 0?(x=w1216) -> (x >= 0?=w1213:bool)
                }
              }
              n516 = Format Into String(format string="Rename %s to %s", w1187, w1181) -> (resulting string=w1185:string)  [unwired: 2 in, 1 out]
              n517 = case shown="True" w1186 {
                tunnel: w1185 -> [_ w1205]
                tunnel: w1184 -> [w1191 w1204]
                tunnel: w1183 -> [_ w1203]
                tunnel: w1181 -> [_ w1198]
                tunnel: w1180 -> [_ w1195]
                tunnel: [w1191 w1192] -> w1179
                frame False {
                }
                frame True {
                  n518 = property class="ProjectItem"(reference=w1203, error in=w1204) -> (error out=w1201:errorcluster, "Reference"=w1202:refnum<vi>, "Path"=w1200:path)  [unwired: 1 out]
                  n519 = call <resource>:"ConvertGoop3ToGoop4_UpdateProgressList.vi"("String"=w1205) -> ()  [unwired: 10 in, 1 out]
                  n520 = Strip Path(path=w1200) -> (stripped path=w1199:path)  [unwired: 1 out]
                  n521 = Build Path(base path=w1199, name or relative path=w1198) -> (appended path=w1197:path)
                  n522 = invoke class="VI" method="Save.Instrument"(reference=w1202, error in=w1201, "Path to saved file"=w1197) -> (reference out=w1193:refnum<vi>, error out=w1196:errorcluster)  [unwired: 3 in, 4 out]
                  n523 = invoke class="LVClassLibrary" method="Save"(reference=w1195, error in=w1196) -> (error out=w1194:errorcluster)  [unwired: 2 in, 3 out]
                  n524 = Close Reference(reference=w1193, error in (no error)=w1194) -> (error out=w1192:errorcluster)
                }
              }
              n525 = Close Reference(reference=w1182, error in (no error)=w1179) -> (error out=w1178:errorcluster)
            }
          }
        }
      }
      frame "ApplyDesignPatterns" {
        n526 = call <resource>:"BaseProvider_DesignPattern_GetPatterns.vi"("error in (no error)"=w1226) -> ("DesignPatterns"=w1238:T25[], "error out"=w1225:errorcluster)  [unwired: 17 in]
        n527 = Unbundle By Name(w1220) -> ("CopyClassesRef"=w1239:refnum<vi>[], "Classes"=w1240:T2[])
        n528 = for {
          tunnel: w1238 -> [w1247] mode=indexing
          shift-right: [w1244] -> w1229
          shift-left: string[] [] -> [w1245]
          shift-right: [w1243] -> w1233
          shift-left: T13 [] -> [w1242]
          n529 = Unbundle By Name(w1247) -> ("Patterns"=w1246:T13)
          n530 = for {
            tunnel: w1246 -> [w1250] mode=indexing
            shift-right: [w1253] -> w1244
            shift-left: w1245 -> [w1252]
            shift-right: [w1248] -> w1243
            shift-left: w1242 -> [w1249]
            n531 = Unbundle By Name(w1250) -> ("ID"=w1251:string)
            n532 = Build Array (concatenate)(w1252, w1251) -> (w1253:string[])
            n533 = Build Array (concatenate)(w1249, w1250) -> (w1248:T13)
          }
        }
        n534 = Search 1D Array(1D array=w1229, element="ClassAttributeEndevoGOOP4") -> (index of element=w1234:i32)  [unwired: 1 in]
        n535 = Search 1D Array(1D array=w1229, element="PersistentEndevoGOOP4") -> (index of element=w1231:i32)  [unwired: 1 in]
        n536 = Search 1D Array(1D array=w1229, element="DebuggingEndevoGOOP4") -> (index of element=w1227:i32)  [unwired: 1 in]
        n537 = Index Array(array=w1233, index #1=w1234, index #2=w1231, index #3=w1227) -> (element #1=w1232:T26, element #2=w1224:T26, element #3=w1223:T26)
        n538 = call <resource>:"ConvertGoop3ToGoop4_UpdateProgressList.vi"("String"="Apply design pattern") -> ("error out"=w1217:errorcluster)  [unwired: 10 in]
        n539 = for {
          tunnel: w1240 -> [w1282] mode=indexing
          tunnel: w1239 -> [w1267] mode=indexing
          tunnel: w1232 -> [w1287]
          tunnel: w1224 -> [w1278]
          tunnel: w1223 -> [w1273]
          shift-right: [w1269] -> w1222
          shift-left: w1225 -> [w1261]
          tunnel: [w1266] -> w1221 mode=indexing
          tunnel: w1217 -> [_]
          w1272 = T27 {"Type"="", "ID"="", "Version"="", "VIPath"=path "", "Name"="", "Data"=variant} ("AddDesignPatternData")
          n540 = local read "ApplyPersistentPattern"() -> (w1264:bool)
          n541 = Unbundle By Name(w1282) -> ("ObjectStatusUsed"=w1262:bool, "UsingClassAttributes"=w1283:bool, "ClassName"=w1260:string)
          n542 = Concatenate Strings(w1260, ":" ("string")) -> (w1257:string)
          n543 = Unbundle By Name(w1287) -> ("ID"=w1258:string, "Version"=w1284:string, "Path"=w1285:path, "Name"=w1286:string)
          n544 = Or(x=w1264, y=w1262) -> (x .or. y?=w1263:bool)
          n545 = Bundle By Name(cluster=w1272, "ID"=w1258, "Version"=w1284, "VIPath"=w1285, "Name"=w1286, "Data"=T15 {"ProcessName"=[]} ("output cluster")) -> (w1288:T27)
          n546 = case shown="True" w1283 {
            tunnel: w1261 -> [w1317 w1322]
            tunnel: w1267 -> [_ w1326]
            tunnel: w1288 -> [_ w1324]
            tunnel: [w1317 w1323] -> w1277
            tunnel: w1257 -> [_ w1320]
            tunnel: w1258 -> [_ w1319]
            frame False {
            }
            frame True {
              n547 = Concatenate Strings(w1320, w1319) -> (w1318:string)
              n548 = call <resource>:"ConvertGoop3ToGoop4_Log.vi"("error in (no error)"=w1322, "Object"=w1318) -> ("error out"=w1321:errorcluster)  [unwired: 7 in, 2 out]
              n549 = call-dynamic "AddDesignPattern.vi"("ClassWriter.lvclass"=refnum<class "ClassWriter.lvclass"> refnum, "ClassItemRefIn"=w1326, "AddDesignPatternData"=w1324, "error in (no error)"=w1321) -> ("error out"=w1323:errorcluster)  [unwired: 13 in, 2 out]
            }
          }
          n550 = Unbundle By Name(w1278) -> ("ID"=w1256:string, "Version"=w1281:string, "Path"=w1280:path, "Name"=w1279:string)
          n551 = Bundle By Name(cluster=w1272, "ID"=w1256, "Version"=w1281, "VIPath"=w1280, "Name"=w1279, "Data"=cluster{"StartAsPersitent":bool} {"StartAsPersitent"=FALSE} ("output cluster")) -> (w1276:T27)
          n552 = Unbundle By Name(w1273) -> ("ID"=w1254:string, "Version"=w1255:string, "Path"=w1274:path, "Name"=w1275:string)
          n553 = Bundle By Name(cluster=w1272, "ID"=w1254, "Version"=w1255, "VIPath"=w1274, "Name"=w1275, "Data"=cluster{"Settings":bool} {"Settings"=FALSE} ("output cluster")) -> (w1271:T27)
          n554 = case shown="True" w1263 {
            tunnel: w1277 -> [w1289 w1294]
            tunnel: w1276 -> [_ w1305]
            tunnel: [w1289 w1301] -> w1269
            tunnel: w1267 -> [_ w1304]
            tunnel: w1271 -> [_ w1299]
            tunnel: w1262 -> [_ w1298]
            tunnel: w1257 -> [_ w1291]
            tunnel: w1256 -> [_ w1292]
            tunnel: w1254 -> [_ w1290]
            frame False {
            }
            frame True {
              n555 = Concatenate Strings(w1291, w1292) -> (w1295:string)
              n556 = local read "ApplyDebuggingSupport"() -> (w1297:bool)
              n557 = call <resource>:"ConvertGoop3ToGoop4_Log.vi"("error in (no error)"=w1294, "Object"=w1295) -> ("error out"=w1293:errorcluster)  [unwired: 7 in, 2 out]
              n558 = Or(x=w1297, y=w1298) -> (x .or. y?=w1296:bool)
              n559 = call-dynamic "AddDesignPattern.vi"("ClassWriter.lvclass"=refnum<class "ClassWriter.lvclass"> refnum, "ClassItemRefIn"=w1304, "AddDesignPatternData"=w1305, "error in (no error)"=w1293) -> ("ClassWriter.lvclass"=w1302:refnum<class "ClassWriter.lvclass">, "ClassItemRefOut"=w1303:refnum<vi>, "error out"=w1300:errorcluster)  [unwired: 13 in]
              n560 = case shown="True" w1296 {
                tunnel: w1303 -> [_ w1316]
                tunnel: w1302 -> [_ w1315]
                tunnel: [w1307 w1314] -> w1301
                tunnel: w1300 -> [w1307 w1311]
                tunnel: w1299 -> [_ w1313]
                tunnel: w1291 -> [_ w1309]
                tunnel: w1290 -> [_ w1308]
                frame False {
                }
                frame True {
                  n561 = Concatenate Strings(w1309, w1308) -> (w1312:string)
                  n562 = call <resource>:"ConvertGoop3ToGoop4_Log.vi"("error in (no error)"=w1311, "Object"=w1312) -> ("error out"=w1310:errorcluster)  [unwired: 7 in, 2 out]
                  n563 = call-dynamic "AddDesignPattern.vi"("ClassWriter.lvclass"=w1315, "ClassItemRefIn"=w1316, "AddDesignPatternData"=w1313, "error in (no error)"=w1310) -> ("error out"=w1314:errorcluster)  [unwired: 13 in, 2 out]
                }
              }
            }
          }
          n564 = property class="LVClassLibrary"(reference=w1267) -> ("Path"=w1266:path)  [unwired: 1 in, 2 out]
        }
        n565 = Bundle By Name(cluster=w1220, "CopyClassPaths"=w1221) -> (w1219:T7)
      }
      frame "CloseCopyClasses" {
        n566 = Unbundle By Name(w1341) -> ("ProjectRef"=w1335:refnum<vi>, "AppRef"=w1327:refnum<vi>, "CopyClassesRef"=w1350:refnum<vi>[])
        n567 = property class="App"(reference=w1327, error in=w1348) -> (error out=w1347:errorcluster, "App.AllVIs"=w1349:string[])  [unwired: 1 out]
        n568 = Close Reference(reference=w1350, error in (no error)=w1347) -> (error out=w1346:errorcluster)
        n569 = Array Size(array=w1349) -> (size(s)=w1343:i32)
        n570 = stacked-sequence {
          tunnel: w1346 -> [w1354]
          tunnel: [w1354] -> w1344
          tunnel: w1343 -> [_]
          frame #0 {
            n571 = Wait (ms)(milliseconds to wait=u32 500) -> ()  [unwired: 1 out]
          }
        }
        n572 = property class="App"(reference=w1327, error in=w1344) -> (error out=w1337:errorcluster, "App.AllVIs"=w1345:string[])  [unwired: 1 out]
        n573 = invoke class="Project" method="Save"(reference=w1335, error in=w1337) -> (reference out=w1338:refnum<vi>, error out=w1339:errorcluster)  [unwired: 2 in, 2 out]
        n574 = Array Size(array=w1345) -> (size(s)=w1342:i32)
        n575 = Close Reference(reference=w1338, error in (no error)=w1339) -> (error out=w1336:errorcluster)
        n576 = stacked-sequence {
          tunnel: w1336 -> [w1352]
          tunnel: [w1352] -> w1333
          tunnel: w1342 -> [_]
          frame #0 {
            n577 = Wait (ms)(milliseconds to wait=u32 500) -> ()  [unwired: 1 out]
          }
        }
        n578 = call <resource>:"ConvertGoop3ToGoop4_UpdateProgressList.vi"("String"="Close copy classes") -> ()  [unwired: 10 in, 1 out]
        n579 = property class="App"(reference=w1327, error in=w1333) -> (reference out=w1329:refnum<vi>, error out=w1331:errorcluster, "App.AllVIs"=w1334:string[])
        n580 = Close Reference(reference=w1329, error in (no error)=w1331) -> (error out=w1330:errorcluster)
        n581 = Array Size(array=w1334) -> (size(s)=w1332:i32)
        n582 = stacked-sequence {
          tunnel: w1332 -> [_]
          frame #0 {
            n583 = Wait (ms)(milliseconds to wait=u32 500) -> ()  [unwired: 1 out]
          }
        }
      }
      frame "CopyNewClassVIsToOldClasses" {
        n584 = Unbundle By Name(w1363) -> ("Classes"=w1362:T2[], "CopyClassPaths"=w1361:path[])
        n585 = call <resource>:"ConvertGoop3ToGoop4_UpdateProgressList.vi"("String"="Copy new class VIs to main project") -> ("error out"=w1356:errorcluster)  [unwired: 10 in]
        n586 = for {
          tunnel: w1362 -> [w1379] mode=indexing
          tunnel: w1361 -> [w1368] mode=indexing
          shift-right: [w1370] -> w1359
          shift-left: w1360 -> [w1372]
          tunnel: w1356 -> [_]
          n587 = Unbundle By Name(w1379) -> ("IsLLB"=w1374:bool, "LvClassPath"=w1366:path, "UsingClassAttributes"=w1364:bool)
          n588 = Strip Path(path=w1368) -> (stripped path=w1367:path)  [unwired: 1 out]
          n589 = case shown="True" w1364 {
            tunnel: [string[] ["New.vi$", "GetObjectStatus.vi$", "GetAttributes.vi$", "CreateReference.vi$", "GetClassAttributes.vi$"] ("VINames") string[] ["New.vi$", "GetObjectStatus.vi$", "GetAttributes.vi$", "CreateReference.vi$"] ("VINames")] -> w1377
            frame True {
            }
            frame False {
            }
          }
          n590 = call <vilib>:"Recursive File List.vi"("pattern"="*.vi", "error in (no error)"=w1372, "Folder Path"=w1367) -> ("error out"=w1371:errorcluster, "All Files in Dir"=w1375:path[])  [unwired: 4 in, 3 out]
          n591 = To Lower Case(string=w1377) -> (all lower case string=w1376:string[])
          n592 = Strip Path(path=w1366) -> (stripped path=w1365:path)  [unwired: 1 out]
          n593 = for {
            tunnel: w1375 -> [w1399]
            tunnel: w1376 -> [w1405] mode=indexing
            tunnel: w1375 -> [w1404]
            tunnel: [w1403] -> w1369 mode=indexing
            n594 = for {
              tunnel: w1405 -> [w1411]
              tunnel: [w1409] -> w1402 mode=indexing
              tunnel: w1399 -> [w1408] mode=indexing
              n595 = Strip Path(path=w1408) -> (name=w1407:string)  [unwired: 1 out]
              n596 = To Lower Case(string=w1407) -> (all lower case string=w1406:string)
              n597 = Match Pattern(string=w1406, regular expression=w1411) -> (offset past match=w1410:i32)  [unwired: 1 in, 3 out]
              n598 = Greater Or Equal To 0?(x=w1410) -> (x >= 0?=w1409:bool)
            }
            n599 = Search 1D Array(1D array=w1402, element=TRUE) -> (index of element=w1400:i32)  [unwired: 1 in]
            n600 = Index Array(array=w1404, index=w1400) -> (element=w1403:path)
          }
          n601 = case shown="False" w1374 {
            tunnel: w1365 -> [w1397 w1398]
            tunnel: [w1395 w1398] -> w1373
            frame False {
              n602 = Build Path(base path=w1397, name or relative path="utils") -> (appended path=w1395:path)
            }
            frame True {
            }
          }
          n603 = for {
            tunnel: w1373 -> [w1386]
            shift-right: [w1384] -> w1370
            shift-left: w1371 -> [w1385]
            tunnel: w1369 -> [w1383] mode=indexing
            n604 = Empty String/Path?(string/path=w1383) -> (empty?=w1382:bool)
            n605 = case shown="False" w1382 {
              tunnel: w1386 -> [w1389 _]
              tunnel: w1385 -> [w1393 w1394]
              tunnel: [w1392 w1394] -> w1384
              tunnel: w1383 -> [w1390 _]
              frame False {
                w1391 = u16 0 items=["overwrite", "ask first", "don't overwrite"] ("overwrite")
                n606 = Strip Path(path=w1390) -> (name=w1387:string)  [unwired: 1 out]
                n607 = Build Path(base path=w1389, name or relative path=w1387) -> (appended path=w1388:path)
                n608 = call <vilib>:"Librarian Copy.vi"("source"=w1390, "error in (no error)"=w1393, "overwrite"=w1391, "destination"=w1388) -> ("error out"=w1392:errorcluster)  [unwired: 6 in, 1 out]
              }
              frame True {
              }
            }
          }
        }
      }
      frame "ModifyClassPrivateData" {
        n609 = Unbundle By Name(w1419) -> ("Classes"=w1416:T2[], "CopyClassPaths"=w1412:path[])
        n610 = call <resource>:"ConvertGoop3ToGoop4_UpdateProgressList.vi"("String"="Modify Class Private Data") -> ("error out"=w1414:errorcluster)  [unwired: 10 in]
        n611 = for {
          shift-right: [w1432] -> w1417
          shift-left: w1418 -> [w1428]
          tunnel: w1416 -> [w1436] mode=indexing
          tunnel: w1414 -> [_]
          tunnel: w1412 -> [w1429] mode=indexing
          w1421 = string[] ["<Property Name=\"EndevoGOOP_ClassProvider\" Type=\"Str\">", "<Property Name=\"EndevoGOOP_TemplateUsed\" Type=\"Str\">", "<Property Name=\"EndevoGOOP_TemplateVersion\" Type=\"Str\">", "<Property Name=\"EndevoGOOP_PlugIns\" Type=\"Bin\">"]
          (unwired) "<Property Name=\"EndevoGOOP_TemplateVersion\" Type=\"Str\">1.0.0.4</Property>" ("regular expression")
          (unwired) "<Property Name=\"EndevoGOOP_TemplateUsed\" Type=\"Str\">G4BaseTemplate_Simple_4x4x4</Property>" ("regular expression")
          (unwired) "<Property Name=\"EndevoGOOP_ClassProvider\" Type=\"Str\">EndevoGOOP400</Property>" ("regular expression")
          n612 = Unbundle By Name(w1436) -> ("LvClassPath"=w1430:path, "IsLLB"=w1434:bool)
          n613 = Read from Text File(file (use dialog)=w1429, error in=w1428) -> (text=w1426:string, error out=w1427:errorcluster)  [unwired: 2 in, 2 out]
          n614 = case shown="True" w1434 {
            tunnel: w1430 -> [w1470 w1474]
            tunnel: w1427 -> [w1471 w1476]
            tunnel: [w1471 w1475] -> w1435
            tunnel: [w1470 w1473] -> w1431
            frame False {
            }
            frame True {
              n615 = call <vilib>:"Generate Temporary File Path.vi"("Temporary File Extension (tmp)"="lvclass") -> ("Unique Temporary File Path"=w1473:path)  [unwired: 9 in, 1 out]
              n616 = call <vilib>:"Copy In Or Out Of VI Library.vi"("source"=w1474, "destination"=w1473, "error in (no error)"=w1476, "safe copy (T)"=FALSE) -> ("error out"=w1475:errorcluster)  [unwired: 2 in, 5 out]
            }
          }
          n617 = for {
            tunnel: w1421 -> [w1459] mode=indexing
            tunnel: w1426 -> [w1461]
            tunnel: [w1456] -> w1420 mode=indexing
            w1457 = "</Property>" ("regular expression")
            n618 = Match Pattern(string=w1461, regular expression=w1459) -> (after substring=w1460:string)  [unwired: 1 in, 3 out]
            n619 = Match Pattern(string=w1460, regular expression=w1457) -> (before substring=w1458:string)  [unwired: 1 in, 3 out]
            n620 = Concatenate Strings(w1459, w1458, w1457) -> (w1456:string)
          }
          n621 = Read from Text File(file (use dialog)=w1431, error in=w1435) -> (text=w1441:string, error out=w1437:errorcluster)  [unwired: 2 in, 2 out]
          n622 = Build Array (concatenate)("<Property Name=\"NI.LVClass.FlattenedPrivateDataCTL\"" ("regular expression"), w1421) -> (w1424:string[])
          n623 = Build Array (concatenate)("<Property Name=\"NI.LVClass.FlattenedPrivateDataCTL\" Type=\"Bin\">#1#!!!!!!!)!\"1!&amp;!!!-!%!!!@````]!!!!\"!!%!!\"=F5F.31QU+!!.-6E.$4%*76Q!!%S1!!!1\"!!!!)!!!%Q1!!!!2!!!!!1R#98.F,GRW9WRB=X-!!!!!!!\"Y#1#!!!!Q!!!I!!!!!!!!\"!!$!$Q!P!!@1)!#!!!!!!%!!1!'`````Q!!!!!!!!!!!!!!!+!W1#RZ#Z6+LKP@)9*Q0O%!!!!-!!!!%!!!!!$\"M+DSX:XB4I\"H;IY+&lt;R:FV\"W-W9]!MA4JA!G9\\0B#@A!!1!!!!!!!!!!!%!!!!!!!!!!!!!!!!!!!!!!!!!!`!!&amp;-6E.$&amp;5*B=W5O&lt;(:D&lt;'&amp;T=TJ#98.F,G.U&lt;!!!!!!!!1!#6EF-1A!!!!\"16%AQ!!!!\"1!\"!!%!!!!!!A!$!!!!!!)!!1!!!!!!'A!,!!)1!\"!\"%!!1\"\"!!-!!1#\"!!%!A1!\"!!!!!!!!\"$!!!\"&amp;(C=9W$!\"0_\"!%AR-D!Q.Q\"J6H4R`V#!23P&amp;!.F=&lt;(91&lt;S]D5\"X4%S#$'9B:Q.ZB90I!R$_164&amp;DU1E!\"?!A4!!!!!!E!!&amp;73524&amp;5*B=W5O&lt;(:D&lt;'&amp;T=TJ#98.F,G.U&lt;!!!!!!!!!!$!!!!J!!!!/RYH+NE9'$).,9QW]#!!-HZ+;EA_A91PW;)DYO+D)Y^0#'U/U?&amp;)TAQ+#S]OU2&amp;J&lt;N'2;/8L&lt;0V!$-$1S^\\:_M2).W^&amp;=4LXANGWX?&lt;7@\\&lt;Q1AUII2V\"]CU5F9Q$YNRJ1Q\\N)!SH7Y;/Z4!N-//3D$N%PI#J,-X295&amp;JGU\"E(]1;!\\)K0^!!**H:'\"G;'@I:ZC/Z!&gt;H@R&gt;8*#\\9,Q$:'$HQ!!!!#QE!A#1!!!-Z,D!!!!!!!)$`````A!!!!9('/Y'\"+5)\"A=]T!9%J#A'\"S8/\"A!!!!@````_!!!!\"A!!!!9!!!!'!!!!\"A!!!!9!!!!'!!!)\"A!!/!9!!0A'!!(Y\"A!$_!9!!`A'!!0Y\"A!$_!9!!`A'!!0TBA!$R_9!!R_'!!\"`\"A!\"`!9!!0!'!!!!\"`````Q!!!A$`````````````````````]2%2%2%2%2%2%2%2%2%2(`%2%2``%2`R%@`R``%2%2`R%2%@%@(R(R]2%@%2%2%@]2%2(`]2``]2`R(`%2%2(`%2%2]2]@%@%2(R]2%2%2`R%2%@`R(R(R``%@`R%2%@]2%2%2%2%2%2%2%2%2%2(``````````````````````T-T-T-T-T-T-T-T-T-T-`]T-T-T-T-T%4-T-T-T-T0`-T-T-T-T'\\OR-T-T-T-T`T-T-T-T'\\%2'\\%T-T-T-`]T-T-T'\\%2%2%&lt;M4-T-T0`-T-T/\\%2%2%2%2OT-T-T`T-T-TOR%2%2%2%@MT-T-`]T-T-\\O\\%2%2%@`\\-T-T0`-T-T/\\O\\M2%@``_T-T-T`T-T-TO\\O\\O\\````MT-T-`]T-T-\\O\\O\\P````\\-T-T0`-T-T/\\O\\O\\````_T-T-T`T-T-TO\\O\\O`````MT-T-`]T-T-\\O\\O\\P````\\-T-T0`-T-T/\\O\\O\\````_T-T-T`T-T-TO\\O\\O````\\P`]T-`]T-T-TO\\O\\P``\\O````T0`-T-T-T/\\O\\`\\O````T-T`T-T-T-T-\\O\\M@````-T-`]T-T-T-T-TM@````-T-T0`-T-T-T-T-T-```-T-T-T`T-T-T-T-T-T-T-T-T-T-``````````````````````Q!!\"!$```````````````````````````````````````````]&amp;\"15&amp;\"15&amp;\"15&amp;\"15&amp;\"15&amp;\"15&amp;\"15&amp;\"15&amp;\"15&amp;\"18``Q5&amp;\"15&amp;\"@```Q5&amp;\"@``\"15&amp;````\"@```Q5&amp;\"15&amp;\"@``\"15&amp;\"15&amp;`Q5&amp;`Q8`\"18`\"@]&amp;\"15&amp;`Q5&amp;\"15&amp;\"15&amp;``]&amp;\"15&amp;\"18```]&amp;\"@````]&amp;\"@``\"18``Q5&amp;\"15&amp;\"18``Q5&amp;\"15&amp;\"@]&amp;\"@]&amp;`Q5&amp;`Q5&amp;\"18`\"@]&amp;\"15&amp;\"15&amp;\"@``\"15&amp;\"15&amp;````\"18`\"18`\"@```Q5&amp;````\"15&amp;\"15&amp;``]&amp;\"15&amp;\"15&amp;\"15&amp;\"15&amp;\"15&amp;\"15&amp;\"15&amp;\"15&amp;\"15&amp;\"18`````````````````````````````````````````````$Q]0$Q]0$Q]0$Q]0$Q]0$Q]0$Q]0$Q]0$Q]0$Q]0``]0$Q]0$Q]0$Q]0$Q]0$Q5&amp;$Q]0$Q]0$Q]0$Q]0$Q```Q]0$Q]0$Q]0$Q]0$Q6:,VF:\"1]0$Q]0$Q]0$Q]0$```$Q]0$Q]0$Q]0$Q6:,Q5&amp;\"16:7150$Q]0$Q]0$Q]0``]0$Q]0$Q]0$Q6:,Q5&amp;\"15&amp;\"15&amp;76E&amp;$Q]0$Q]0$Q```Q]0$Q]0$Q^:,Q5&amp;\"15&amp;\"15&amp;\"15&amp;\"6F:$Q]0$Q]0$```$Q]0$Q]0$S]P\"15&amp;\"15&amp;\"15&amp;\"15&amp;L6E0$Q]0$Q]0``]0$Q]0$Q]0,VF:,Q5&amp;\"15&amp;\"15&amp;L;WN,Q]0$Q]0$Q```Q]0$Q]0$Q]P76F:73]&amp;\"15&amp;L;WNL;UP$Q]0$Q]0$```$Q]0$Q]0$S^:76F:76EP7;WNL;WNL3]0$Q]0$Q]0``]0$Q]0$Q]0,VF:76F:76GNL;WNL;WN,Q]0$Q]0$Q```Q]0$Q]0$Q]P76F:76F:7;WNL;WNL;UP$Q]0$Q]0$```$Q]0$Q]0$S^:76F:76F:L;WNL;WNL3]0$Q]0$Q]0``]0$Q]0$Q]0,VF:76F:76GNL;WNL;WN,Q]0$Q]0$Q```Q]0$Q]0$Q]P76F:76F:7;WNL;WNL;UP$Q]0$Q]0$```$Q]0$Q]0$VF:76F:76F:L;WNL;WN76GML+Q0$Q]0``]0$Q]0$Q]0$S]P76F:76GNL;WN76EPL+SML+SM$Q```Q]0$Q]0$Q]0$Q]P76F:7;WN76EPL+SML+SM$Q]0$```$Q]0$Q]0$Q]0$Q]0,VF:76E&amp;L+SML+SML!]0$Q]0``]0$Q]0$Q]0$Q]0$Q]0$S]&amp;L+SML+SML!]0$Q]0$Q```Q]0$Q]0$Q]0$Q]0$Q]0$Q]0L+SML!]0$Q]0$Q]0$```$Q]0$Q]0$Q]0$Q]0$Q]0$Q]0$Q]0$Q]0$Q]0$Q]0````````````````````````````````````````````!!!!!A!\"!!!!!!!E!!&amp;'5%B1&amp;5*B=W5O&lt;(:D&lt;'&amp;T=TJ#98.F,G.U&lt;!!!!!!!!!!$!!!$CQ!!\"Z^YH+V647M4523^&lt;T+NEZD3FVKVQ&gt;:]]*)7.4&lt;YV1^K'X5C6&amp;3U6&gt;'K;'R3&amp;=2)%[5L&gt;4%)821%I23FY+J&lt;&amp;VXIIAO2\\';D&amp;13L%0U(CB1,&gt;D,?._FE*EFN2=TC]:,==_ZZ^ZRZ!\\$B'7U3#H\"@!U)8=8.=!V&gt;3*1#ZC!1L(XK7`!,3[#5;R+3T^*.1)-U;O*.K7)L+Y`!.3`8H?CO]*]0U+Z&lt;75C]SO43I4[J&lt;0=&gt;9HL)8T7S]RK3EM*V/E)*QHPF_3B.+'LO\"UM:84Y15A-A\"563#JR+X5QLDPTIDEN?A&gt;'J!:&lt;6OF/6&lt;E2&amp;&lt;PT%IB:UE+039F)#5&lt;4!\\/WO\"0%61W*$2C2A3\"#\"\\B:VL9\"JEN38$]LM-D-P!9*_^:B`:6XD#N8.1*834L&amp;+%)GZMZ=A=;_+UW+KY'RIUMPRBS3N^43[1ON0+3S\"!=F=E`:6_D_-^*\\E,2GU$'M&amp;5%OIG&gt;\"#`$GKQ1V'&amp;K]!HL/P9LQ_G$#&gt;%UYE?\\M22QQGH0%\\\"MG*K(3NE-2&gt;M/8,L&lt;C;&lt;'P7H2`T$NR+:D0`/[-V\\C7T+HURE%^5G(:26&lt;Q=@!'^GZ!-;191?[,=00!UT-T-Y!VQN;#^#N\\*]#5?2/A9H3E.07M0D8;XB^?(QZ+5TV`E!1^W#,&lt;-$6G&lt;X9'9^N&amp;*477&lt;X```-(M!IX;`),-3B$=[NE&lt;_/)MD+,.9$&gt;%&amp;]$5QH9B\\9-YO9/',/L:`:LKL-=GR&amp;:C=H*SMTWVX+L%B)-&lt;0+7XV:8_&lt;*8&gt;:`Q$Y9MC8X&amp;.KBK,&amp;;[O\"2`9Z&gt;P.C&amp;'\\$\"./$]([/[?7U(`,8!YZI-$K2'+ETYIM'&amp;J#J[^\\#]KSS5,G\"QS$SF\\D&amp;//4]`D[@%V?161!H!1V&amp;1'0`6'6'SI7DHW!KV7Y-BT'QPSQM'=^118+]PQD9=22LGZO;1$6?0$U]J5#]J/0QZ8`&amp;-&lt;H!L@K-EQ&amp;=;8,&amp;J7!JS_OJ3\\E#!L_7F4J_FZC+K16==.D8.K+&lt;NX^6=_XMVV]L5&lt;.4A%KL\"K&gt;=8T8RN0H9-8+DGY]*H6(0XU80WG\"C#;HA84L15,89U^OWW`7\\&lt;0G,N@\\[TN=5Y8V\\F'L(F_=`8S!4G/81\"1E-A,QWYCZ?*)_S(=%!0\"\\(/?&gt;,W`%G@J-&amp;1KY0*?N5@.)Z]$T49,\"^J?%X\\_1-A^5NR/IU8%&gt;Z*7[2J;4(XI@4?T\"UPP7W6NY,I;'&gt;0@6,4&lt;U\\V*&lt;5!!!!!\"!!!!#I!!!!!!!!!!!!!!!!!!!!E!!&amp;#2%B1&amp;5*B=W5O&lt;(:D&lt;'&amp;T=TJ#98.F,G.U&lt;!!!!!!!!!!$!!!!9A!!!(*YH'.A9-A4E'$[RV$XFY&amp;*Y#O1)@W8A6H1D`%X!Q/HH]\"B)-UI)!E5FPX,Q#[I$2&lt;70K,,Q1!&amp;KGS-(*)=BQ5ZQ$)=,2I-````Z`B[Z\"J=R2%@/&amp;.FFDS(\"!!59BE!!!!!!!!%!!!!\"Q!!!FU!!!!(!!!!)6^O;6^-98.U3WZP&gt;WZ0&gt;WZJ&lt;G&gt;-6E.M98.T1WRV=X2F=AE!A!!!!!!\"!!A!-0````]!!1!!!!!!01!!!!)!#5!(!!.3:79!,%\"1!!%!!#.(.%*B=W65:7VQ&lt;'&amp;U:6^4;7VQ&lt;'6@.HAY?$9O&lt;(:D&lt;'&amp;T=Q!\"!!%!!!!!!!!!'ER71WRB=X.1=GFW982F2'&amp;U962B9E^S:'6S#1#!!!!!!!)!\"1!(!!!-!%!!!@````]!!!!\"!!%!!!!\"!!!!!!!!!!!!!!!&lt;4&amp;:$&lt;'&amp;T=V\"S;8:B&gt;'6%982B6'FN:8.U97VQ#1#!!!!!!!%!\"1!(!!!\"!!$);&lt;$K!!!!!!!!!#:-6E.M98.T5(*J&gt;G&amp;U:52B&gt;'&amp;-98.U18\"Q&lt;'FF:&amp;2J&lt;76T&gt;'&amp;N=!E!A!!!!!!\"!!5!\"Q!!!1!!S'GQ[A!!!!!!!!!;4&amp;:$&lt;'&amp;T=V\"S;8:B&gt;'6%982B6(FQ:52F=W-*!)!!!!!!!1!)!$$`````!!%!!!!!!$U!!!!#!!F!\"Q!$5G6G!#R!5!!\"!!!D2T2#98.F6'6N='RB&gt;'6@5WFN='RF8T:Y/(AW,GRW9WRB=X-!!1!\"!!!!!!!!!\"Z-6E.M98.T5(*J&gt;G&amp;U:52B&gt;'&amp;%:GRU2'&amp;U96.J?G5*!)!!!!!!!1!&amp;!!-!!!%!!!!!!!1!!!!!!!!!'ER71WRB=X.1=GFW982F2'&amp;U952G&lt;(2%982B#1#!!!!!!!)!#5!(!!.3:79!,%\"1!!%!!#.(.%*B=W65:7VQ&lt;'&amp;U:6^4;7VQ&lt;'6@.HAY?$9O&lt;(:D&lt;'&amp;T=Q!\"!!%!!!!!!!!!!!!!!!!!!!1!!Q!.!!!!\"!!!!)U!!!!I!!!!!A!!\"!!!!!!5!!!!!!!!!!!!!!!!!!!!!!!!!!!!!!!!!!!!!!!!!)!!!!!!!1!!!!!!!!!!!!!!!!!!!)!-EAE!!!!!!!.-!F66B5!!4A!*!!!!!A!!!!!!!!!!!!!!!!!!!!!!!!!!!!!!!!!!!!!!!!!!!!!!!!!!!!!!!!!!!!!!!+OK+D[LKCI_K[IK0KOK+DY!!!!!!!.-!A!!!$]!!!!!!!!!!!!!!E%!!!/0?*S.5MNSUU!1&lt;&amp;O7XY\\NR#'1&amp;_96)%\"Y\"/[KW/8#\"R+8&lt;?#+MLN+K7KN&amp;&gt;J6SK9Y]%F]\"N`#D4M(2J+./8,;G:[?W&gt;\\:\"P!'&amp;;=%;SQ]P-7P(`\\XHQ$S^4.8CR.ZT;3L&gt;4F.G*%Y&gt;E&lt;)!1=^'7MDIK\\SOCGD'U&lt;_N7N%F\\P'225-S0UGJAU,F();_:,#-DZ26#&gt;EB$Q+6%[JO%H56)5HLV\"WPFFK&lt;$*!+!]NOD4JL;\"KR&gt;T$U8_*M&amp;'CKV*KQ_)?`RO&lt;_4J7=BW,O=%G#3OC2B)XU%1,\\;8!L]2I/HG5/60$A)MZ5(/+M0WQJQ+U(2MVP1B9X^?B&gt;\"&gt;%N6'B?:(\\8AN/6\"M&amp;4\\I';$AZ&amp;*E+TO.:EFAI%8\\6HVSME_G\\)869+(!^_1*M58/&gt;=`5R]IXI+3[!09)[\"*U,1:TY]M.Q9NT)R#%S+&lt;YGD4ZTD9J3+76@4ZALX3C::K'OQDZN[-,TN$\"*CY7;_1@:);!NZI)FW-B%3TA6++4J*\\);.,&lt;%6,A9C]`J_WSJ[!L[.0JS4[A-#`L_4'?;%OYI5GT)Z^AG9#-\"\"J';D5W19#GL/P-VEQ.;AA&lt;*M.'+AZAW/0#F&amp;.(:QIB-&lt;F8(F^.&amp;+*+^9&gt;&gt;*4&amp;6I-8+$GP6I\\/JF_VFF=VW:KF8N-+NVVL6%T+LKE!]/U-%W&lt;G#(\\(E,O^D$0G'(O)UO\\O!O\\O%_(O!)$`%)DX'-*XC+:TD\"=\\R97DZ(JM`]5[#Y1'?4TDQZL%2/W])L]NEJI;&gt;Y46%&gt;_!-ZA=&amp;7!!!!!!!!8Q!\"!!)!!Q!%!!!!3!!/\"!!!!!!/!/=!VA!!!%]!$A1!!!!!$A$H!.9!!!\"7!!Y%!!!!!!Y!ZQ$7!!!!89!!B!#!!!!/!/=!VA:597BP&lt;7%'6'&amp;I&lt;WVB\"F2B;'^N91%Q!&amp;*45E-.#A!$4&amp;:$1UR#6F=!!\"-E!!!%!1!!!#!!!\"-%!!!!!!!!!!!!!!!A!!!!.!!!!`A!!!!&gt;4%F#4A!!!!!!!!&amp;M4&amp;:45A!!!!!!!!'!5F242Q!!!!!!!!'54%FW;1!!!!!!!!'I1U^/5!!!!!!!!!']6%UY-!!!!!!!!!(12%:%5Q!!!!!!!!(E4%FE=Q!!!!!!!!(Y6EF$2!!!!!!!!!)-&gt;G6S=Q!!!!!!!!)A35.04A!!!!!!!!)U;7.M.!!!!!!!!!*);7.M/!!!!!!!!!*=1V\"$-A!!!!!!!!*Q4%FG=!!!!!!!!!+%2F\")9A!!!!!!!!+92F\"421!!!!!!!!+M36\"45A!!!!!!!!,!1UZ46!!!!!!!!!,54&amp;\"*4A!!!!!!!!,I4%FC:!!!!!!!!!,]1E2)9A!!!!!!!!-11E2421!!!!!!!!-E6EF55Q!!!!!!!!-Y2&amp;2)5!!!!!!!!!.-466*2!!!!!!!!!.A3%F46!!!!!!!!!.U5&amp;*5)!!!!!!!!!/)6E.55!!!!!!!!!/=2F2\"1A!!!!!!!!/Q!!!!!0````]!!!!!!!!!!!!!!!!!!!!!!!!!!!!!!!!!!!!9!!!!!!!!!!$`````!!!!!!!!!*1!!!!!!!!!!0````]!!!!!!!!!K!!!!!!!!!!!`````Q!!!!!!!!$M!!!!!!!!!!$`````!!!!!!!!!01!!!!!!!!!!0````]!!!!!!!!\"&amp;!!!!!!!!!!!`````Q!!!!!!!!&amp;=!!!!!!!!!!$`````!!!!!!!!!91!!!!!!!!!\"0````]!!!!!!!!#,!!!!!!!!!!!`````Q!!!!!!!!)]!!!!!!!!!!$`````!!!!!!!!!M!!!!!!!!!!!0````]!!!!!!!!%R!!!!!!!!!!!`````Q!!!!!!!!D)!!!!!!!!!!$`````!!!!!!!!#.!!!!!!!!!!!0````]!!!!!!!!)_!!!!!!!!!!!`````Q!!!!!!!!S)!!!!!!!!!!$`````!!!!!!!!$*!!!!!!!!!!!0````]!!!!!!!!-F!!!!!!!!!!!`````Q!!!!!!!!S9!!!!!!!!!!$`````!!!!!!!!$*Q!!!!!!!!!!0````]!!!!!!!!-R!!!!!!!!!!!`````Q!!!!!!!!UM!!!!!!!!!!$`````!!!!!!!!$41!!!!!!!!!!0````]!!!!!!!!0G!!!!!!!!!!!`````Q!!!!!!!!_A!!!!!!!!!!$`````!!!!!!!!$[A!!!!!!!!!!0````]!!!!!!!!0V!!!!!!!!!!!`````Q!!!!!!!\"\"9!!!!!!!!!)$`````!!!!!!!!%K!!!!!!#%*B=W5O9X2M!!!!!!</Property>", w1420) -> (w1422:string[])
          n624 = for {
            tunnel: w1424 -> [w1445] mode=indexing
            tunnel: w1422 -> [w1444] mode=indexing
            shift-right: [w1446] -> w1438
            shift-left: w1441 -> [w1442]
            n625 = Match Pattern(string=w1442, regular expression=w1445) -> (before substring=w1447:string, after substring=w1448:string, offset past match=w1443:i32)  [unwired: 1 in, 1 out]
            n626 = case shown="Default" w1443 {
              tunnel: w1448 -> [_ w1455]
              tunnel: w1447 -> [_ w1454]
              tunnel: [w1449 w1452] -> w1446
              tunnel: w1444 -> [_ w1450]
              tunnel: w1442 -> [w1449 _]
              frame -1 {
              }
              frame Default {
                n627 = Match Pattern(string=w1455, regular expression="</Property>") -> (after substring=w1453:string)  [unwired: 1 in, 3 out]
                n628 = Concatenate Strings(w1454, w1450, w1453) -> (w1452:string)
              }
            }
          }
          n629 = Delete(path (use dialog)=w1431, error in=w1437) -> (deleted path=w1439:path, error out=w1440:errorcluster)  [unwired: 3 in, 1 out]
          n630 = Write to Text File(file (use dialog)=w1439, text=w1438, error in=w1440) -> (error out=w1433:errorcluster)  [unwired: 1 in, 2 out]
          n631 = case shown="True" w1434 {
            tunnel: w1433 -> [w1462 w1469]
            tunnel: [w1462 w1463] -> w1432
            tunnel: w1431 -> [_ w1465]
            tunnel: w1430 -> [_ w1468]
            frame False {
            }
            frame True {
              w1466 = u16 0 items=["overwrite", "ask first", "don't overwrite"] ("overwrite")
              n632 = call <vilib>:"Copy In Or Out Of VI Library.vi"("source"=w1465, "destination"=w1468, "error in (no error)"=w1469, "safe copy (T)"=FALSE, "overwrite"=w1466, "remove original (F)"=TRUE) -> ("error out"=w1463:errorcluster)  [unwired: 5 out]
            }
          }
        }
      }
      frame "-------------------------------------------" {
      }
      frame "OpenMainProjectAgain" {
        n633 = Unbundle By Name(w1503) -> ("Project"=w1483:path)
        n634 = call <resource>:"ConvertGoop3ToGoop4_UpdateProgressList.vi"("error in (no error)"=w1492, "String"="Open Main project") -> ("error out"=w1491:errorcluster)  [unwired: 9 in]
        n635 = Open Application Reference(8:w1491) -> (0:w1495:errorcluster, 3:w1496:refnum<vi>)  [unwired: 3 in]
        n636 = invoke class="App" method="Project.Open"(reference=w1496, error in=w1495, "Path"=w1483) -> (reference out=w1497:refnum<vi>, error out=w1500:errorcluster, "Project:Open"=w1488:refnum<vi>)  [unwired: 1 in, 1 out]
        n637 = disable-structure shown="Enabled" {
          disable-tunnel: w1488 -> [w1505 w1506]
          disable-tunnel: [w1504 w1506] -> w1487
          frame Disabled {
            n638 = invoke class="Project" method="Open Window"(reference=w1505) -> (reference out=w1504:refnum<vi>)  [unwired: 2 in, 2 out]
          }
          frame Enabled {
          }
        }
        n639 = property class="Project"(reference=w1487, error in=w1500) -> (reference out=w1499:refnum<vi>, error out=w1498:errorcluster, "App Ref"=w1489:refnum<vi>)
        n640 = property class="App"(reference=w1489) -> ("App.AllVIs"=w1490:string[])  [unwired: 1 in, 2 out]
        n641 = Array Size(array=w1490) -> (size(s)=w1482:i32)
        n642 = property class="Project"(reference=w1499, error in=w1498) -> (error out=w1494:errorcluster, "My Computer"=w1486:refnum<vi>)  [unwired: 1 out]
        n643 = Bundle By Name(cluster=w1503, "ProjectRef"=w1499, "AppRef"=w1489, "My Computer"=w1486) -> (w1502:T7)
        n644 = Format Into String(format string="Project Opened:%s, %d VIs", w1483, w1482) -> (resulting string=w1481:string)  [unwired: 2 in, 1 out]
        n645 = Close Reference(reference=w1497, error in (no error)=w1494) -> (error out=w1485:errorcluster)
        n646 = call <resource>:"ConvertGoop3ToGoop4_Log.vi"("error in (no error)"=w1485, "Object"=w1481) -> ()  [unwired: 7 in, 3 out]
      }
      frame "OpenClassReferences" {
        n647 = Unbundle By Name(w1510) -> ("Classes"=w1516:T2[], "AppRef"=w1513:refnum<vi>)
        n648 = for {
          tunnel: w1516 -> [w1526] mode=indexing
          tunnel: [w1527] -> w1515 mode=indexing
          tunnel: w1513 -> [w1525]
          shift-right: [w1523] -> w1509
          shift-left: w1507 -> [w1522]
          n649 = Unbundle By Name(w1526) -> ("LvClassPath"=w1519:path, "ClassName"=w1520:string)
          n650 = invoke class="App" method="LVClass.Open"(reference=w1525, "Path"=w1519) -> (error out=w1521:errorcluster, "LVClass.Open"=w1524:refnum<vi>)  [unwired: 2 in, 2 out]
          n651 = case shown="Error" w1521 {
            tunnel: w1520 -> [_ w1530]
            tunnel: w1519 -> [_ w1528]
            frame No Error {
            }
            frame Error {
              n652 = Format Into String(format string="OpenClassError:%s,%s", w1530, w1528) -> (resulting string=w1529:string)  [unwired: 2 in, 1 out]
              n653 = call <resource>:"ConvertGoop3ToGoop4_Log.vi"("Object"=w1529) -> ()  [unwired: 8 in, 3 out]
            }
          }
          n654 = Bundle By Name(cluster=w1526, "ClassRef"=w1524) -> (w1527:T2)
          n655 = Select(t=w1521, s=w1521, f=w1522) -> (s? t:f=w1523:errorcluster)
        }
        n656 = Unbundle By Name(w1510) -> ("ProjectRef"=w1511:refnum<vi>)
        n657 = Bundle By Name(cluster=w1510, "Classes"=w1515) -> (w1514:T7)
        n658 = Merge Errors(w1507, w1509) -> (w1508:errorcluster)
        n659 = disable-structure shown="Disabled" {
          disable-tunnel: w1511 -> [w1518 _]
          disable-tunnel: w1508 -> [w1517 _]
          frame Disabled {
            n660 = invoke class="Project" method="Open Window"(reference=w1518, error in=w1517) -> ()  [unwired: 1 in, 3 out]
          }
          frame Enabled {
          }
        }
      }
      frame "ReplaceGetAttToModifyToGetAttribute" {
        n661 = Unbundle By Name(w1535) -> ("Classes"=w1540:T2[])
        n662 = call <resource>:"ConvertGoop3ToGoop4_UpdateProgressList.vi"("String"="Replace GetAttributyeToModify To GetAttribute") -> ("error out"=w1532:errorcluster)  [unwired: 10 in]
        n663 = for {
          tunnel: w1540 -> [w1548] mode=indexing
          shift-right: [w1555] -> w1538
          shift-left: w1539 -> [w1554]
          tunnel: [w1546] -> w1536 mode=indexing
          tunnel: w1532 -> [_]
          n664 = Unbundle By Name(w1548) -> ("ClassRef"=w1556:refnum<vi>)
          n665 = Unbundle By Name(w1548) -> ("LvClassPath"=w1552:path)
          n666 = invoke class="LVClassLibrary" method="Get All Descendents"(reference=w1556, error in=w1554, "Type"="VI") -> (error out=w1553:errorcluster, "All Descendents"=w1557:refnum<vi>[])  [unwired: 4 in, 5 out]
          n667 = Strip Path(path=w1552) -> (stripped path=w1544:path)  [unwired: 1 out]
          n668 = call <vilib>:"Recursive File List.vi"("pattern"="*GetAttributes.vi" ("regular expression"), "Folder Path"=w1544) -> ("All Files in Dir"=w1550:path[])  [unwired: 5 in, 4 out]
          n669 = call <vilib>:"Recursive File List.vi"("pattern"="*GetClassAttributes.vi" ("regular expression"), "Folder Path"=w1544) -> ("All Files in Dir"=w1543:path[])  [unwired: 5 in, 4 out]
          n670 = Index Array(array=w1550) -> (element=w1549:path)  [unwired: 1 in]
          n671 = Index Array(array=w1543) -> (element=w1542:path)  [unwired: 1 in]
          n672 = for {
            tunnel: w1557 -> [w1572] mode=indexing
            shift-right: [w1567] -> w1555
            shift-left: w1553 -> [w1568]
            tunnel: w1549 -> [w1562]
            shift-right: [w1561] -> w1547
            shift-left: refnum<vi>[] [] -> [w1560]
            tunnel: w1542 -> [w1559]
            n673 = property class="ProjectItem"(reference=w1572, error in=w1568) -> (reference out=w1571:refnum<vi>, error out=w1569:errorcluster, "Reference"=w1570:refnum<vi>, "Name"=w1566:string)
            n674 = Match Pattern(string=w1566, regular expression="GetObjectStatus.vi$") -> (offset past match=w1564:i32)  [unwired: 1 in, 3 out]
            n675 = Greater Or Equal To 0?(x=w1564) -> (x >= 0?=w1563:bool)
            n676 = Close Reference(reference=w1571) -> ()  [unwired: 1 in, 1 out]
            n677 = case shown="False" w1563 {
              tunnel: w1570 -> [w1584 w1612]
              tunnel: w1569 -> [w1583 w1613]
              tunnel: [w1580 w1613] -> w1567
              tunnel: w1562 -> [w1578 _]
              tunnel: [w1577 w1611] -> w1561
              tunnel: w1560 -> [w1576 w1611]
              tunnel: w1559 -> [w1573 _]
              frame False {
                n678 = invoke class="VI" method="Get VI Dependencies"(reference=w1584, error in=w1583, "Include Standard VIs?"=TRUE) -> (reference out=w1581:refnum<vi>, error out=w1582:errorcluster, "Dependency Names"=w1586:string[])  [unwired: 16 in, 16 out]
                n679 = for {
                  tunnel: w1586 -> [w1591] mode=indexing
                  tunnel: "GetAttributesToModify\\2Evi$" ("regular expression") -> [w1594]
                  tunnel: [w1589] -> w1579
                  tunnel: "GetClassAttributesToModify\\2Evi$" ("regular expression") -> [w1588]
                  stop <- w1589 stop-if-true
                  n680 = Match Pattern(string=w1591, regular expression=w1594) -> (offset past match=w1593:i32)  [unwired: 1 in, 3 out]
                  n681 = Match Pattern(string=w1591, regular expression=w1588) -> (offset past match=w1592:i32)  [unwired: 1 in, 3 out]
                  n682 = Greater Or Equal To 0?(x=w1593) -> (x >= 0?=w1587:bool)
                  n683 = Greater Or Equal To 0?(x=w1592) -> (x >= 0?=w1590:bool)
                  n684 = Or(x=w1587, y=w1590) -> (x .or. y?=w1589:bool)
                }
                n685 = case shown="True" w1579 {
                  tunnel: w1582 -> [w1597 w1603]
                  tunnel: w1581 -> [w1598 w1601]
                  tunnel: [w1596 w1599] -> w1580
                  tunnel: w1578 -> [_ w1605]
                  tunnel: [w1595 w1608] -> w1577
                  tunnel: w1576 -> [w1595 w1606]
                  tunnel: w1573 -> [_ w1604]
                  frame False {
                    n686 = Close Reference(reference=w1598, error in (no error)=w1597) -> (error out=w1596:errorcluster)
                  }
                  frame True {
                    n687 = call <resource>:"ConvertGoop3ToGoop4_Log.vi"("error in (no error)"=w1603, "Object"=w1601) -> ("error out"=w1602:errorcluster)  [unwired: 7 in, 2 out]
                    n688 = call <resource>:"ConvertGoop3ToGoop4_ReplaceGetAttToModify.vi"("error in (no error)"=w1602, "GetClassAttributeVI"=w1604, "GetAttributeVI"=w1605, "ViRef"=w1601) -> ("error out"=w1609:errorcluster, "ViRefOut"=w1610:refnum<vi>)  [unwired: 6 in]
                    n689 = invoke class="VI" method="Save.Instrument"(reference=w1610, error in=w1609) -> (reference out=w1607:refnum<vi>, error out=w1600:errorcluster)  [unwired: 4 in, 4 out]
                    n690 = Build Array (concatenate)(w1606, w1607) -> (w1608:refnum<vi>[])
                    n691 = call <resource>:"ConvertGoop3ToGoop4_ClearErrors.vi"("error in (no error)"=w1600) -> ("error out"=w1599:errorcluster)  [unwired: 9 in, 1 out]
                  }
                }
              }
              frame True {
                n692 = Close Reference(reference=w1612) -> ()  [unwired: 1 in, 1 out]
              }
            }
          }
          n693 = Bundle By Name(cluster=w1548, "VIsModiifingData"=w1547) -> (w1546:T2)
        }
        n694 = Bundle By Name(cluster=w1535, "Classes"=w1536) -> (w1534:T7)
      }
      frame "RewireGetAttributes" {
        n695 = Unbundle By Name(w1619) -> ("Classes"=w1622:T2[])
        n696 = call <resource>:"ConvertGoop3ToGoop4_UpdateProgressList.vi"("String"="Rewire GetAttribute VIs") -> ("error out"=w1615:errorcluster)  [unwired: 10 in]
        n697 = for {
          N -> [w1625]
          tunnel: w1622 -> [w1624] mode=indexing
          shift-right: [w1633] -> w1620
          shift-left: w1621 -> [w1632]
          tunnel: [w1628] -> w1617 mode=indexing
          tunnel: w1615 -> [_]
          i -> [w1627]
          n698 = Unbundle By Name(w1624) -> ("ClassName"=w1623:string)
          n699 = Unbundle By Name(w1624) -> ("ClassRef"=w1634:refnum<vi>)
          n700 = invoke class="LVClassLibrary" method="Get All Descendents"(reference=w1634, error in=w1632, "Type"="VI") -> (error out=w1631:errorcluster, "All Descendents"=w1635:refnum<vi>[])  [unwired: 4 in, 5 out]
          n701 = Increment(x=w1627) -> (x+1=w1626:i32)
          n702 = for {
            N -> [w1642]
            tunnel: w1635 -> [w1661] mode=indexing
            shift-right: [w1656] -> w1633
            shift-left: w1631 -> [w1657]
            shift-right: [w1650] -> w1629
            shift-left: refnum<vi>[] [] -> [w1652]
            tunnel: w1626 -> [w1641]
            tunnel: w1625 -> [w1640]
            tunnel: w1623 -> [w1639]
            i -> [w1643]
            n703 = property class="ProjectItem"(reference=w1661, error in=w1657) -> (reference out=w1660:refnum<vi>, error out=w1658:errorcluster, "Reference"=w1659:refnum<vi>, "Name"=w1651:string)
            n704 = Match Pattern(string=w1651, regular expression="GetObjectStatus.vi$") -> (offset past match=w1654:i32)  [unwired: 1 in, 3 out]
            n705 = Greater Or Equal To 0?(x=w1654) -> (x >= 0?=w1653:bool)
            n706 = Increment(x=w1643) -> (x+1=w1637:i32)
            n707 = Close Reference(reference=w1660) -> ()  [unwired: 1 in, 1 out]
            n708 = Divide(x=w1637, y=w1642) -> (x/y=w1649:dbl)
            n709 = Multiply(x=w1649, y=100.0) -> (x*y=w1645:dbl)
            n710 = Format Into String(format string="Rewire GetAttribute VIs %d of %d (%d%%) : %s", w1641, w1640, w1645, w1639) -> (resulting string=w1646:string)  [unwired: 2 in, 1 out]
            n711 = call <resource>:"ConvertGoop3ToGoop4_UpdateProgressList.vi"("UpdateLastLine(False)"=TRUE, "String"=w1646) -> ("error out"=w1638:errorcluster)  [unwired: 9 in]
            n712 = case shown="False" w1653 {
              tunnel: w1659 -> [w1672 w1696]
              tunnel: w1658 -> [w1671 w1697]
              tunnel: [w1668 w1697] -> w1656
              tunnel: w1652 -> [w1667 w1695]
              tunnel: [w1666 w1695] -> w1650
              tunnel: w1638 -> [_ _]
              frame False {
                n713 = invoke class="VI" method="Get VI Dependencies"(reference=w1672, error in=w1671, "Include Standard VIs?"=TRUE) -> (reference out=w1669:refnum<vi>, error out=w1670:errorcluster, "Dependency Names"=w1665:string[])  [unwired: 16 in, 16 out]
                n714 = for {
                  tunnel: w1665 -> [w1678] mode=indexing
                  tunnel: "GetAttributes.vi$" -> [w1681]
                  tunnel: [w1676] -> w1664
                  tunnel: "GetClassAttributes.vi$" -> [w1675]
                  stop <- w1676 stop-if-true
                  n715 = Match Pattern(string=w1678, regular expression=w1681) -> (offset past match=w1680:i32)  [unwired: 1 in, 3 out]
                  n716 = Match Pattern(string=w1678, regular expression=w1675) -> (offset past match=w1679:i32)  [unwired: 1 in, 3 out]
                  n717 = Greater Or Equal To 0?(x=w1680) -> (x >= 0?=w1674:bool)
                  n718 = Greater Or Equal To 0?(x=w1679) -> (x >= 0?=w1677:bool)
                  n719 = Or(x=w1674, y=w1677) -> (x .or. y?=w1676:bool)
                }
                n720 = case shown="True" w1664 {
                  tunnel: w1670 -> [w1684 w1690]
                  tunnel: w1669 -> [w1685 w1688]
                  tunnel: [w1683 w1686] -> w1668
                  tunnel: w1667 -> [w1682 w1693]
                  tunnel: [w1682 w1691] -> w1666
                  frame False {
                    n721 = Close Reference(reference=w1685, error in (no error)=w1684) -> (error out=w1683:errorcluster)
                  }
                  frame True {
                    n722 = call <resource>:"ConvertGoop3ToGoop4_Log.vi"("error in (no error)"=w1690, "Object"=w1688) -> ("error out"=w1689:errorcluster)  [unwired: 7 in, 2 out]
                    n723 = call <resource>:"ConvertGoop3ToGoop4_RewireGetAttributes.vi"("error in (no error)"=w1689, "ViRef"=w1688) -> ("error out"=w1694:errorcluster, "ViRefOut"=w1692:refnum<vi>)  [unwired: 8 in]
                    n724 = invoke class="VI" method="Save.Instrument"(reference=w1692, error in=w1694) -> (error out=w1687:errorcluster)  [unwired: 4 in, 5 out]
                    n725 = Build Array (concatenate)(w1693, w1692) -> (w1691:refnum<vi>[])
                    n726 = call <resource>:"ConvertGoop3ToGoop4_ClearErrors.vi"("error in (no error)"=w1687) -> ("error out"=w1686:errorcluster)  [unwired: 9 in, 1 out]
                  }
                }
              }
              frame True {
                n727 = Close Reference(reference=w1696) -> ()  [unwired: 1 in, 1 out]
              }
            }
          }
          n728 = Bundle By Name(cluster=w1624, "GetAttViRefs"=w1629) -> (w1628:T2)
        }
        n729 = Bundle By Name(cluster=w1619, "Classes"=w1617) -> (w1618:T7)
      }
      frame "RewireGetObjectStatus" {
        n730 = Unbundle By Name(w1700) -> ("Classes"=w1705:T2[])
        n731 = for {
          tunnel: w1705 -> [w1711] mode=indexing
          shift-right: [w1713] -> w1703
          shift-left: w1704 -> [w1714]
          tunnel: [w1710] -> w1701 mode=indexing
          n732 = Unbundle By Name(w1711) -> ("ClassRef"=w1715:refnum<vi>)
          n733 = invoke class="LVClassLibrary" method="Get All Descendents"(reference=w1715, error in=w1714, "Type"="VI") -> (error out=w1712:errorcluster, "All Descendents"=w1709:refnum<vi>[])  [unwired: 4 in, 5 out]
          n734 = for {
            tunnel: w1709 -> [w1728] mode=indexing
            shift-right: [w1725] -> w1713
            shift-left: w1712 -> [w1720]
            tunnel: [w1720] -> w1708
            shift-right: [w1719] -> w1706
            shift-left: FALSE -> [w1717]
            n735 = property class="ProjectItem"(reference=w1728, error in=w1720) -> (error out=w1726:errorcluster, "Reference"=w1727:refnum<vi>, "Name"=w1724:string)  [unwired: 1 out]
            n736 = Match Pattern(string=w1724, regular expression="Destroy.vi$") -> (offset past match=w1722:i32)  [unwired: 1 in, 3 out]
            n737 = Greater Or Equal To 0?(x=w1722) -> (x >= 0?=w1721:bool)
            n738 = case shown="False" w1721 {
              tunnel: w1727 -> [w1736 w1758]
              tunnel: w1726 -> [w1735 w1759]
              tunnel: [w1734 w1759] -> w1725
              tunnel: [w1732 _] -> w1718
              frame False {
                n739 = invoke class="VI" method="Get VI Dependencies"(reference=w1736, error in=w1735, "Include Standard VIs?"=TRUE) -> (reference out=w1730:refnum<vi>, error out=w1729:errorcluster, "Dependency Names"=w1738:string[])  [unwired: 16 in, 16 out]
                n740 = for {
                  tunnel: w1738 -> [w1741] mode=indexing
                  tunnel: [w1739] -> w1731
                  tunnel: string[] ["GetObjectStatus.vi$"] -> [w1740]
                  stop <- w1739 stop-if-true
                  n741 = for {
                    tunnel: w1741 -> [w1744]
                    tunnel: w1740 -> [w1743] mode=indexing
                    tunnel: [w1742] -> w1739
                    stop <- w1742 stop-if-true
                    n742 = Match Pattern(string=w1744, regular expression=w1743) -> (offset past match=w1745:i32)  [unwired: 1 in, 3 out]
                    n743 = Greater Or Equal To 0?(x=w1745) -> (x >= 0?=w1742:bool)
                  }
                }
                n744 = case shown="True" w1731 {
                  tunnel: w1729 -> [w1747 w1753]
                  tunnel: w1730 -> [w1748 w1751]
                  tunnel: [w1746 w1749] -> w1734
                  tunnel: [_ w1755] -> w1732
                  frame False {
                    n745 = Close Reference(reference=w1748, error in (no error)=w1747) -> (error out=w1746:errorcluster)
                  }
                  frame True {
                    n746 = call <resource>:"ConvertGoop3ToGoop4_Log.vi"("error in (no error)"=w1753, "Object"=w1751) -> ("error out"=w1752:errorcluster)  [unwired: 7 in, 2 out]
                    n747 = call <resource>:"ConvertGoop3ToGoop4_UpdateGetObjectStatusCallers.vi"("error in (no error)"=w1752, "RemoveWire"=FALSE, "ViRef"=w1751) -> ("error out"=w1757:errorcluster, "UsingObjectCallers"=w1755:bool, "ViRefOut"=w1756:refnum<vi>)  [unwired: 6 in]
                    n748 = Close Reference(reference=w1756, error in (no error)=w1757) -> (error out=w1750:errorcluster)
                    n749 = call <resource>:"ConvertGoop3ToGoop4_ClearErrors.vi"("error in (no error)"=w1750) -> ("error out"=w1749:errorcluster)  [unwired: 9 in, 1 out]
                  }
                }
              }
              frame True {
                n750 = Close Reference(reference=w1758) -> ()  [unwired: 1 in, 1 out]
              }
            }
            n751 = Or(x=w1717, y=w1718) -> (x .or. y?=w1719:bool)
          }
          n752 = Close Reference(reference=w1709, error in (no error)=w1708) -> ()  [unwired: 1 out]
          n753 = Bundle By Name(cluster=w1711, "ObjectStatusUsed"=w1706) -> (w1710:T2)
        }
        n754 = call <resource>:"ConvertGoop3ToGoop4_UpdateProgressList.vi"("String"="Find GetObjectStatus") -> ()  [unwired: 10 in, 1 out]
        n755 = Bundle By Name(cluster=w1700, "Classes"=w1701) -> (w1699:T7)
      }
      frame "RemoveGetObjectStatus" {
        n756 = Unbundle By Name(w1764) -> ("Classes"=w1765:T2[])
        n757 = for {
          tunnel: w1765 -> [w1773] mode=indexing
          shift-right: [w1771] -> w1762
          shift-left: w1763 -> [w1770]
          (unwired) T28."invalid VI type" ("VI Type")
          n758 = Unbundle By Name(w1773) -> ("ObjectStatusUsed"=w1766:bool, "ClassRef"=w1772:refnum<vi>)
          n759 = invoke class="LVClassLibrary" method="Get All Descendents"(reference=w1772, error in=w1770, "Type"="VI") -> (error out=w1767:errorcluster, "All Descendents"=w1768:refnum<vi>[])  [unwired: 4 in, 5 out]
          n760 = for {
            tunnel: w1768 -> [w1785] mode=indexing
            shift-right: [w1774] -> w1771
            shift-left: w1767 -> [w1783]
            tunnel: w1766 -> [w1775]
            n761 = property class="ProjectItem"(reference=w1785, error in=w1783) -> (reference out=w1784:refnum<vi>, error out=w1779:errorcluster, "Reference"=w1780:refnum<vi>)
            n762 = property class="VI"(reference=w1780, error in=w1779) -> (reference out=w1777:refnum<vi>, error out=w1778:errorcluster, "VIType"=w1776:T28)
            n763 = Close Reference(reference=w1784) -> ()  [unwired: 1 in, 1 out]
            n764 = case shown="\"Standard VI\"" w1776 {
              tunnel: [w1786 w1789] -> w1782
              tunnel: [w1787 w1795] -> w1781
              tunnel: w1778 -> [w1786 w1793]
              tunnel: w1777 -> [w1787 w1791]
              tunnel: w1775 -> [_ w1790]
              frame "invalid VI type", Default {
              }
              frame "Standard VI" {
                n765 = call <resource>:"ConvertGoop3ToGoop4_Log.vi"("error in (no error)"=w1793, "Object"=w1791) -> ("error out"=w1792:errorcluster)  [unwired: 7 in, 2 out]
                n766 = call <resource>:"ConvertGoop3ToGoop4_RemoveGetObjectStatus.vi"("error in (no error)"=w1792, "RelinkOnly"=w1790, "ViRef"=w1791) -> ("error out"=w1796:errorcluster, "Modified"=w1794:bool, "ViRefOut"=w1797:refnum<vi>)  [unwired: 6 in]
                n767 = case shown="True" w1794 {
                  tunnel: [w1798 w1803] -> w1788
                  tunnel: w1797 -> [w1799 w1802]
                  tunnel: w1796 -> [w1798 w1801]
                  tunnel: [w1799 w1800] -> w1795
                  frame False {
                  }
                  frame True {
                    n768 = invoke class="VI" method="Save.Instrument"(reference=w1802, error in=w1801) -> (reference out=w1800:refnum<vi>, error out=w1803:errorcluster)  [unwired: 4 in, 4 out]
                  }
                }
                n769 = call <resource>:"ConvertGoop3ToGoop4_ClearErrors.vi"("error in (no error)"=w1788) -> ("error out"=w1789:errorcluster)  [unwired: 9 in, 1 out]
              }
            }
            n770 = Close Reference(reference=w1781, error in (no error)=w1782) -> (error out=w1774:errorcluster)
          }
        }
        n771 = call <resource>:"ConvertGoop3ToGoop4_UpdateProgressList.vi"("String"="FindGetAttributeVIs") -> ()  [unwired: 10 in, 1 out]
      }
      frame "------------------------------------------------" {
      }
      frame "UpdateSubClass-GetAttributesWithUnbundleByName" {
        n772 = Unbundle By Name(w1812) -> ("Classes"=w1813:T2[])
        n773 = call <resource>:"ConvertGoop3ToGoop4_UpdateProgressList.vi"("String"="Update Sub classes Get Attribute callers") -> ("error out"=w1807:errorcluster)  [unwired: 10 in]
        n774 = for {
          N -> [w1819]
          tunnel: w1813 -> [w1826] mode=indexing
          shift-right: [w1825] -> w1810
          shift-left: w1811 -> [w1824]
          tunnel: w1807 -> [_]
          i -> [w1814]
          n775 = Unbundle By Name(w1826) -> ("GetAttViRefs"=w1821:refnum<vi>[], "AllInheritanceClasses"=w1823:path[])
          n776 = Empty Array?(array=w1823) -> (empty?=w1822:bool)
          n777 = Increment(x=w1814) -> (x+1=w1820:i32)
          n778 = Format Into String(format string="Update Sub classes Get Attribute callers %d of %d", w1820, w1819) -> (resulting string=w1817:string)  [unwired: 2 in, 1 out]
          n779 = call <resource>:"ConvertGoop3ToGoop4_UpdateProgressList.vi"("UpdateLastLine(False)"=TRUE, "String"=w1817) -> ("error out"=w1815:errorcluster)  [unwired: 9 in]
          n780 = case shown="True" w1822 {
            tunnel: w1821 -> [w1827 w1839]
            tunnel: [w1829 w1840] -> w1825
            tunnel: w1824 -> [w1830 w1841]
            tunnel: w1823 -> [w1828 _]
            tunnel: w1815 -> [_ _]
            frame False {
              # "Also remove Always Copy"
              n781 = for {
                tunnel: w1827 -> [w1833] mode=indexing
                shift-right: [w1831] -> w1829
                shift-left: w1830 -> [w1835]
                tunnel: w1828 -> [w1836]
                n782 = call <resource>:"ConvertGoop3ToGoop4_Log.vi"("error in (no error)"=w1835, "Object"=w1833) -> ("error out"=w1834:errorcluster)  [unwired: 7 in, 2 out]
                n783 = call <resource>:"ConvertGoop3ToGoop4_UpdateGetAttributes.vi"("error in (no error)"=w1834, "BaseClasses"=w1836, "ViRef"=w1833) -> ("error out"=w1837:errorcluster, "ViRefOut"=w1838:refnum<vi>)  [unwired: 7 in]
                n784 = invoke class="VI" method="Save.Instrument"(reference=w1838, error in=w1837) -> (error out=w1832:errorcluster)  [unwired: 4 in, 5 out]
                n785 = call <resource>:"ConvertGoop3ToGoop4_ClearErrors.vi"("error in (no error)"=w1832) -> ("error out"=w1831:errorcluster)  [unwired: 9 in, 1 out]
              }
            }
            frame True {
              # "Also remove Always Copy"
              n786 = for {
                tunnel: w1839 -> [w1842] mode=indexing
                shift-right: [w1846] -> w1840
                shift-left: w1841 -> [w1845]
                n787 = call <resource>:"ConvertGoop3ToGoop4_RemoveAlwaysCopy.vi"("error in (no error)"=w1845, "ViRef"=w1842) -> ("error out"=w1844:errorcluster, "ViRefOut"=w1843:refnum<vi>)  [unwired: 8 in]
                n788 = invoke class="VI" method="Save.Instrument"(reference=w1843, error in=w1844) -> (error out=w1846:errorcluster)  [unwired: 4 in, 5 out]
              }
            }
          }
        }
      }
      frame "CreateIP-Nodes" {
        n789 = Unbundle By Name(w1852) -> ("Classes"=w1853:T2[])
        n790 = call <resource>:"ConvertGoop3ToGoop4_UpdateProgressList.vi"("String"="Create IP Nodes") -> ("error out"=w1848:errorcluster)  [unwired: 10 in]
        n791 = for {
          N -> [w1855]
          tunnel: w1853 -> [w1861] mode=indexing
          shift-right: [w1860] -> w1850
          shift-left: w1851 -> [w1859]
          tunnel: w1848 -> [_]
          i -> [w1857]
          n792 = Unbundle By Name(w1861) -> ("ClassName"=w1854:string, "VIsModiifingData"=w1858:refnum<vi>[])  [unwired: 1 out]
          n793 = Increment(x=w1857) -> (x+1=w1856:i32)
          n794 = for {
            N -> [w1875]
            tunnel: w1858 -> [w1879] mode=indexing
            shift-right: [w1862] -> w1860
            shift-left: w1859 -> [w1880]
            tunnel: w1856 -> [w1868]
            tunnel: w1855 -> [w1867]
            tunnel: w1854 -> [w1865]
            i -> [w1877]
            n795 = call <resource>:"ConvertGoop3ToGoop4_Log.vi"("error in (no error)"=w1880, "Object"=w1879) -> ("error out"=w1870:errorcluster)  [unwired: 7 in, 2 out]
            n796 = Increment(x=w1877) -> (x+1=w1876:i32)
            n797 = Divide(x=w1876, y=w1875) -> (x/y=w1874:dbl)
            n798 = Multiply(x=w1874, y=100.0) -> (x*y=w1866:dbl)
            n799 = Format Into String(format string="Create IP Nodes %d of %d (%d%%) : %s", w1868, w1867, w1866, w1865) -> (resulting string=w1871:string)  [unwired: 2 in, 1 out]
            n800 = call <resource>:"ConvertGoop3ToGoop4_UpdateProgressList.vi"("error in (no error)"=w1870, "UpdateLastLine(False)"=TRUE, "String"=w1871) -> ("error out"=w1869:errorcluster)  [unwired: 8 in]
            n801 = call <resource>:"ConvertGoop3ToGoop4_CreateInPlacementNode.vi"("error in (no error)"=w1869, "ViRefIn"=w1879) -> ("error out"=w1878:errorcluster, "ViRefOut"=w1881:refnum<vi>)  [unwired: 8 in]
            n802 = invoke class="VI" method="Save.Instrument"(reference=w1881, error in=w1878) -> (error out=w1863:errorcluster)  [unwired: 4 in, 5 out]
            n803 = call <resource>:"ConvertGoop3ToGoop4_ClearErrors.vi"("error in (no error)"=w1863) -> ("error out"=w1862:errorcluster)  [unwired: 9 in, 1 out]
          }
        }
      }
      frame "UpdateObjectAttributes" {
        n804 = Unbundle By Name(w1889) -> ("AppRef"=w1884:refnum<vi>, "Classes"=w1885:T2[])
        n805 = call <resource>:"ConvertGoop3ToGoop4_UpdateProgressList.vi"("String"="Update Object Attribute") -> ("error out"=w1882:errorcluster)  [unwired: 10 in]
        n806 = for {
          tunnel: w1885 -> [w1896] mode=indexing
          shift-right: [w1893] -> w1887
          shift-left: w1888 -> [w1894]
          tunnel: w1884 -> [w1890]
          tunnel: w1882 -> [_]
          n807 = Unbundle By Name(w1896) -> ("ClassRef"=w1895:refnum<vi>, "AllInheritanceClasses"=w1892:path[])
          n808 = Empty Array?(array=w1892) -> (empty?=w1891:bool)
          n809 = case shown="False" w1891 {
            tunnel: w1895 -> [w1916 _]
            tunnel: w1894 -> [w1915 w1954]
            tunnel: [w1897 w1954] -> w1893
            tunnel: w1890 -> [w1912 _]
            frame False {
              w1925 = refnum<vi> refnum  # Cluster
              n810 = call <resource>:"GDSLvClass_GetClassMethod.vi"("Class Refnum In"=w1916, "VINames"=string[] ["ObjectAttributes.ctl"], "error in (no error)"=w1915) -> ("ViPaths"=w1911:path[], "error out"=w1913:errorcluster)  [unwired: 13 in, 2 out]
              n811 = Index Array(array=w1911) -> (element=w1910:path)  [unwired: 1 in]
              n812 = Open VI Reference(application reference (local)=w1912, vi path=w1910, error in (no error)=w1913) -> (vi reference=w1906:refnum<vi>, error out=w1908:errorcluster)  [unwired: 3 in]
              n813 = call <resource>:"ConvertGoop3ToGoop4_Log.vi"("error in (no error)"=w1908, "Object"=w1906) -> ("error out"=w1907:errorcluster)  [unwired: 7 in, 2 out]
              n814 = property class="VI"(reference=w1906, error in=w1907, "Front Panel.Open"=FALSE ("Front Panel Window:Open")) -> (reference out=w1917:refnum<vi>, error out=w1924:errorcluster, "Panel"=w1901:refnum<vi>)
              n815 = property class="Pnl"(reference=w1901, error in=w1924) -> (error out=w1927:errorcluster, "Controls[]"=w1904:refnum<vi>[])  [unwired: 1 out]
              n816 = Index Array(array=w1904) -> (element=w1926:refnum<vi>)  [unwired: 1 in]
              n817 = Array Size(array=w1904) -> (size(s)=w1903:i32)
              n818 = To More Specific Class(target class=w1925, reference=w1926, error in=w1927) -> (specific class reference=w1900:refnum<vi>, error out=w1923:errorcluster)
              n819 = property class="Clust"(reference=w1900, error in=w1923) -> (error out=w1922:errorcluster, "Controls[]"=w1909:refnum<vi>[])  [unwired: 1 out]
              n820 = for {
                tunnel: w1909 -> [w1953] mode=indexing
                tunnel: [w1948] -> w1921
                shift-right: [w1947] -> w1918
                shift-left: w1922 -> [w1949]
                tunnel: [w1946] -> w1920
                i -> [w1948]
                stop <- w1946 stop-if-true
                n821 = property class="Ctl"(reference=w1953, error in=w1949) -> (error out=w1947:errorcluster, "Label.Text"=w1952:string)  [unwired: 1 out]
                n822 = Search 1D Array(1D array=string[] ["Base class", "Base"], element=w1952) -> (index of element=w1950:i32)  [unwired: 1 in]
                n823 = Greater Or Equal To 0?(x=w1950) -> (x >= 0?=w1946:bool)
              }
              n824 = Index Array(array=w1909, index=w1921) -> (element=w1919:refnum<vi>)
              n825 = case shown="True" w1920 {
                tunnel: w1919 -> [_ w1945]
                tunnel: w1918 -> [w1940 w1944]
                tunnel: [w1940 w1942] -> w1899
                tunnel: w1917 -> [_ w1941]
                frame False {
                }
                frame True {
                  n826 = invoke class="Ctl" method="Delete"(reference=w1945, error in=w1944) -> (error out=w1943:errorcluster)  [unwired: 1 in, 2 out]
                  n827 = invoke class="VI" method="Save.Instrument"(reference=w1941, error in=w1943) -> (error out=w1942:errorcluster)  [unwired: 4 in, 5 out]
                }
              }
              n828 = case shown="1" w1903 {
                tunnel: [w1928 w1929] -> w1902
                tunnel: w1899 -> [w1928 w1937]
                tunnel: w1900 -> [_ w1936]
                frame 0, Default {
                }
                frame 1 {
                  w1938 = refnum<vi> refnum  # Boolean
                  w1939 = 21012 items=[".NET Refnum"=3441, "Absolute Value"=1054, "Access Rights"=1412, "ActiveX Container"=2072, "Add"=1050, "Add Array Elements"=1903, "Agitator"=3831, "AllSpoll"=1960, "And"=1061, "And Array Elements"=1911, "Append True/False String"=1511, "Application Refnum"=3412, "Array"=3300, "Array 1"=21608, "Array Constant"=2070, "Array Max & Min"=1907, "Array Size"=1809, "Array Subset"=2044, "Array To Cluster"=1168, "Array To Spreadsheet String"=1540, "Array of Strings to Path"=1422, "Atmospheric Tank"=3070, "Atmospheric Tank 1"=21751, "Automation Close"=8001, "Automation Open"=8000, "Automation Refnum"=3410, "Avogadro Constant (1/mol)"=2030, "Base 10 Logarithm Of e"=2022, "Bin"=3073, "Bin 1"=21755, "Bluetooth Close Connection"=9148, "Bluetooth Create Listener"=9151, "Bluetooth Discover"=9152, "Bluetooth Network Connection Refnum"=3468, "Bluetooth Open Connection"=9153, "Bluetooth Read"=9149, "Bluetooth Wait On Listener"=9147, "Bluetooth Write"=9150, "Boolean Array To Number"=1815, "Boolean To (0,1)"=1167, "Build Array"=2041, "Build Cluster Array"=2047, "Build Path"=1419, "Build Waveform"=2066, "Bundle"=2049, "Bundle By Name"=2057, "Byte Array To String"=1609, "Byte Stream File Refnum"=3408, "Call By Reference Node"=3901, "Call Chain"=1999, "Call Library Function Node"=2062, "Cancel Button"=3131, "Cancel Button 1"=21739, "Cancel Notification"=9107, "Carriage Return Constant"=2010, "Case Structure"=2001, "Cast Unit Bases"=1079, "Check Valve"=3833, "Checkbox"=3117, "Class Specifier Constant"=2094, "Classic Radio Buttons"=22003, "Close File"=1405, "Close Reference"=8011, "Cluster"=21607, "Cluster 1"=3400, "Cluster Constant"=2071, "Cluster To Array"=1169, "Code Interface Node"=2050, "Color Box"=3013, "Color Box Constant"=2120, "Color Box Thin Border"=2905, "Color Ramp"=3022, "Combo Box"=3304, "Combo Box 1"=21604, "Combo Box Constant"=2088, "Complex Conjugate"=1048, "Complex To Polar"=1045, "Complex To Re/Im"=1044, "Compound Arithmetic"=2200, "Compressor"=3832, "Concatenate Strings"=2040, "Conditional Disable Structure"=2064, "Constructor Node"=3904, "Control Help Window"=1353, "Control Online Help"=1355, "Control Refnum"=3419, "Convert Unit"=2059, "Conveyer"=3827, "Copy"=1416, "Cosecant"=1204, "Cosine"=1201, "Cotangent"=1205, "Create User Event"=2073, "Current VI's Menubar"=9000, "Current VI's Path"=1426, "DAQmx Analog Trigger Source"=21774, "DAQmx Analog Trigger Source 1"=21951, "DAQmx Analog Trigger Source 2"=3336, "DAQmx Analog Trigger Source Constant"=2119, "DAQmx Device Name"=21950, "DAQmx Device Name 1"=21773, "DAQmx Device Name 2"=3318, "DAQmx Device Name Constant"=2093, "DAQmx Global Channel"=21770, "DAQmx Global Channel 1"=21957, "DAQmx Global Channel 2"=3443, "DAQmx Global Channel Constant"=3430, "DAQmx Physical Channel"=21954, "DAQmx Physical Channel 1"=3335, "DAQmx Physical Channel 2"=21777, "DAQmx Physical Channel Constant"=2118, "DAQmx Scale Name"=21775, "DAQmx Scale Name 1"=3317, "DAQmx Scale Name 2"=21952, "DAQmx Scale Name Constant"=2116, "DAQmx Switch"=3337, "DAQmx Switch 1"=21776, "DAQmx Switch 2"=21953, "DAQmx Switch Constant"=2121, "DAQmx Task Name"=21778, "DAQmx Task Name 1"=21959, "DAQmx Task Name 2"=3442, "DAQmx Task Name Constant"=3434, "DAQmx Terminal"=21781, "DAQmx Terminal 1"=3319, "DAQmx Terminal 2"=21955, "DAQmx Terminal Constant"=2117, "Data Log File Refnum"=3402, "DataSocket Close"=1085, "DataSocket Open"=1084, "DataSocket Read"=1086, "DataSocket Refnum"=3417, "DataSocket Write"=1087, "Database Variant To Data"=8004, "Date/Time To Seconds"=1308, "Decimal Digit?"=1119, "Decimal String To Number"=1184, "Decimate 1D Array"=2046, "Decrement"=1058, "Default Directory"=1427, "Delete"=1417, "Delete From Array"=3912, "Delete Menu Items"=9004, "Delete Variant Attribute"=8206, "Delete Waveform Attribute"=8209, "Dequeue Element"=9113, "Destroy User Event"=2075, "DevClear"=1961, "DevClearList"=1962, "Device Control/Status"=1433, "Device Refnum"=3405, "Diagram Disable Structure"=2054, "Dial"=3050, "Dial 1"=21732, "Dialog Button"=3130, "Dialog Checkbox"=3132, "Dialog Chiseled Line"=3632, "Dialog Colored Rectangle"=3625, "Dialog Combo Box"=21917, "Dialog Horizontal Pointer Slide"=21902, "Dialog Horizontal Progress Bar"=21910, "Dialog Horizontal Slide"=21904, "Dialog Label"=21961, "Dialog Listbox"=21921, "Dialog Listbox 1"=2105, "Dialog Multicolumn Listbox"=21220, "Dialog Multiple Selection Multicolumn Listbox"=21221, "Dialog Numeric"=21919, "Dialog Path Control"=21922, "Dialog Pict Ring"=21925, "Dialog Radio Button"=3133, "Dialog Radio Buttons"=22002, "Dialog Recessed Frame"=3624, "Dialog Ring"=3060, "Dialog Spin Control"=21900, "Dialog String"=21920, "Dialog Tab Control"=3331, "Dialog Table"=21225, "Dialog Tree"=21794, "Dialog Vertical Pointer Slide"=21901, "Dialog Vertical Progress Bar"=21909, "Dialog Vertical Slide"=21903, "Digital Data"=3210, "Digital Data 1"=21216, "Digital Waveform Graph"=3511, "Digital Waveform Graph 1"=3502, "Digital Waveform Graph 2"=21718, "Divide"=1053, "Dlg CheckBox"=21924, "Dlg Horiz Scrollbar"=21905, "Dlg Numeric"=2100, "Dlg Numeric 2"=3006, "Dlg String"=2110, "Dlg Vert Scrollbar"=21906, "Down Arrow"=3824, "Down Bow Valve"=3707, "Down Bow Valve 1"=3807, "Down Bow Valve 2"=21767, "Down Rect Valve"=3706, "Down Rect Valve 1"=21766, "Down Rect Valve 2"=3806, "Down Tee"=3718, "Down Tee 1"=3818, "EOF"=1410, "Elementary Charge (C)"=2027, "Empty Path Constant"=2033, "Empty String Constant"=2013, "Empty String/Path?"=1112, "Enable Menu Tracking"=9002, "EnableLocal"=1963, "EnableRemote"=1964, "End of Line Constant"=2035, "Enqueue Element"=9111, "Enqueue Element At Opposite End"=9129, "Enum"=21605, "Enum 1"=3023, "Enum Constant"=2090, "Equal To 0?"=1113, "Equal?"=1102, "Error Ring Constant"=2039, "Event Callback Refnum"=3435, "Event Structure"=2052, "Exchanger"=3828, "Exclusive Or"=1063, "Exponential"=1211, "Exponential (Arg) -1"=1222, "Expression Node"=2201, "False Constant"=2006, "Feedback Node"=2353, "FieldPoint IO Point"=3439, "FieldPoint IO Point 1"=21784, "FieldPoint IO Point Constant"=3440, "File Dialog"=8081, "File Path Control"=21730, "File Path Control 1"=3203, "File Path Indicator"=21731, "File Path Indicator 1"=3204, "File/Directory Info"=1413, "FindLstn"=1965, "FindRQS"=1966, "First Call?"=1083, "Flat Box"=3602, "Flat Circle"=3605, "Flat Down Triangle"=3623, "Flat Frame"=3608, "Flat Left Triangle"=3620, "Flat Right Triangle"=3621, "Flat Round Button"=3102, "Flat Rounded Box"=3611, "Flat Sequence Structure"=2069, "Flat Square Button"=3103, "Flat Up Triangle"=3622, "Flatten To String"=1160, "Flatten To XML"=8400, "Flattened String To Variant"=8202, "Flush File"=1406, "Flush Queue"=9114, "For Loop"=2002, "Format Date/Time String"=8100, "Format Into File"=2083, "Format Into String"=2081, "Format Value"=1512, "Formula Node"=2004, "Fract/Exp String To Number"=1187, "Framed Color Box"=21019, "Framed Color Box 1"=3008, "Free Label"=2321, "Furnace"=3829, "GPIB Clear"=1954, "GPIB Initialization"=1957, "GPIB Misc"=1956, "GPIB Read"=1951, "GPIB Serial Poll"=1955, "GPIB Status"=1959, "GPIB Trigger"=1953, "GPIB Wait"=1958, "GPIB Write"=1950, "Gauge"=21009, "Gauge 1"=3040, "Generate Front Panel Activity"=1329, "Generate Occurrence"=1700, "Generate User Event"=2074, "Generic Refnum"=3428, "Generic Refnum By Reference Flatten"=3453, "Generic Refnum Deep Copy"=3447, "Generic Refnum Name"=21745, "Generic Refnum Tag"=3429, "Generic Refnum Tag By Reference Flatten"=3454, "Generic Refnum Tag Flatten"=21747, "Get Date/Time In Seconds"=1303, "Get Date/Time String"=1600, "Get Help Window Status"=1354, "Get Menu Item Info"=9005, "Get Menu Selection"=9001, "Get Menu Short Cut Info"=9007, "Get Notifier Status"=9103, "Get Queue Status"=9110, "Get Variant Attribute"=8205, "Get Waveform Attribute"=8208, "Get Waveform Components"=2067, "Global Variable"=2060, "Gravitational Constant (N m2/kg2)"=2029, "Greater Or Equal To 0?"=1114, "Greater Or Equal?"=1103, "Greater Than 0?"=1117, "Greater?"=1110, "Handle Peek"=1604, "Handle Poke"=1605, "Hex Digit?"=1123, "Hexadecimal String To Number"=1185, "HiQ-Script"=9021, "Hopper"=3072, "Hopper 1"=21754, "Horiz Line"=3821, "Horiz Pipe"=3710, "Horiz Pipe 1"=3810, "Horizontal Button Box"=3636, "Horizontal Fill Slide"=21100, "Horizontal Fill Slide 1"=3012, "Horizontal Graduated Bar"=21106, "Horizontal Pointer Slide"=3011, "Horizontal Pointer Slide 1"=21101, "Horizontal Progress Bar"=21102, "Horizontal Slide"=3010, "Horizontal Slide Switch"=3114, "Horizontal Smooth Box"=3633, "Horizontal Switch"=3108, "Horizontal Tank"=3071, "Horizontal Toggle Switch"=3110, "Horizontal Toggle Switch 1"=21700, "Hyperbolic Cosine"=1215, "Hyperbolic Sine"=1214, "Hyperbolic Tangent"=1216, "IMAQ Session"=3415, "IP To String"=1710, "IVI Delete Session"=8103, "IVI Logical Name"=3414, "IVI Logical Name 1"=21736, "IVI Logical Name Constant"=3420, "IVI New Session"=8102, "Implies"=1080, "In Range and Coerce"=1127, "Increment"=1057, "Index & Bundle Cluster Array"=2056, "Index Array"=2042, "Index String Array"=1531, "Initialize Array"=2053, "Insert Into Array"=3911, "Insert Menu Items"=9003, "Intensity Chart"=3509, "Intensity Chart 1"=21719, "Intensity Graph"=3510, "Intensity Graph 1"=21720, "Interleave 1D Arrays"=2045, "Interpolate 1D Array"=1905, "Inverse Cosine"=1207, "Inverse Hyperbolic Cosine"=1218, "Inverse Hyperbolic Sine"=1217, "Inverse Hyperbolic Tangent"=1219, "Inverse Sine"=1206, "Inverse Tangent"=1208, "Inverse Tangent (2 Input)"=1228, "Invoke Node"=3900, "IrDA Close Connection"=9144, "IrDA Create Listener"=9140, "IrDA Discover"=9141, "IrDA Network Connection Refnum"=3450, "IrDA Open Connection"=9142, "IrDA Read"=9145, "IrDA Wait On Listener"=9143, "IrDA Write"=9146, "Join Numbers"=1171, "Knob"=21000, "Knob 1"=3005, "LED Button"=3116, "Label"=21960, "Labeled Oblong Button"=3125, "Labeled Rectangular Button"=3124, "Labeled Round Button"=3122, "Labeled Square Button"=3123, "Left Arrow"=3826, "Left Bow Valve"=3701, "Left Bow Valve 1"=3801, "Left Bow Valve 2"=21761, "Left Down Elbow"=3811, "Left Down Elbow 1"=3711, "Left Pump"=3813, "Left Pump 1"=3713, "Left Rect Valve"=3700, "Left Rect Valve 1"=21760, "Left Rect Valve 2"=3800, "Left Tee"=3809, "Left Tee 1"=3709, "Left Up Elbow"=3708, "Left Up Elbow 1"=3808, "Less Or Equal To 0?"=1115, "Less Or Equal?"=1104, "Less Than 0?"=1118, "Less?"=1111, "Lexical Class"=1126, "Line Feed Constant"=2011, "List Directory"=1418, "Listbox"=21210, "Listbox 1"=3206, "Listbox Symbol Ring Constant"=2038, "Local Variable"=2061, "Lock Range"=1411, "Logarithm Base 10"=1210, "Logarithm Base 2"=1225, "Logarithm Base X"=1224, "Logical Shift"=1081, "Lowered Rounded Box"=3638, "MATLAB Script"=9020, "MakeAddr"=1967, "Mantissa & Exponent"=1150, "Match First String"=1532, "Match Pattern"=1535, "Match True/False String"=1533, "Max & Min"=1108, "Menu Refnum"=3413, "Menu Ring"=3018, "Menu Ring 1"=21600, "Menu-Popup Ring"=3017, "Merge Signals"=2350, "Meter"=21008, "Meter 1"=3030, "Molar Gas Constant (J/(mol K))"=2032, "Motion Resource"=3448, "Motion Resource 1"=21787, "Motion Resource Constant"=3449, "Motor"=3720, "Motor 1"=3820, "Move"=1415, "Multicolumn Listbox"=21204, "Multicolumn Listbox 1"=21205, "Multicolumn Listbox 2"=3307, "Multicolumn Listbox 3"=21214, "Multicolumn Listbox 4"=21215, "Multiple Selection Listbox"=21211, "Multiple Selection Listbox 1"=3207, "Multiple Selection Listbox 2"=3208, "Multiple Selection Listbox 3"=21201, "Multiple Selection Multicolumn Listbox"=3308, "Multiply"=1052, "Multiply Array Elements"=1904, "Natural Logarithm"=1209, "Natural Logarithm (Arg +1)"=1221, "Natural Logarithm Base"=2020, "Natural Logarithm Of 10"=2023, "Natural Logarithm Of 2"=2024, "Natural Logarithm Of Pi"=2018, "Negate"=1069, "Negative Infinity"=2019, "New Directory"=1402, "New File"=1404, "New VI"=8014, "New VI Object"=8015, "Not"=1064, "Not A Number/Path/Refnum?"=1128, "Not A Path Constant"=2034, "Not And"=1071, "Not Equal To 0?"=1116, "Not Equal?"=1105, "Not Exclusive Or"=1073, "Not Or"=1072, "Not a Refnum Constant"=2036, "Not a Tag"=2037, "Number To Boolean Array"=1814, "Number To Decimal String"=1180, "Number To Engineering String"=1183, "Number To Exponential String"=1505, "Number To Fractional String"=1506, "Number To Hexadecimal String"=1181, "Number To Octal String"=1182, "Numeric Constant"=2005, "Numeric Control"=21003, "Numeric Control 1"=3000, "Numeric Indicator"=21004, "Numeric Indicator 1"=3001, "OK Button"=21738, "OLE Variant"=3150, "Obtain Notifier"=9101, "Obtain Queue"=9108, "Occurrence Refnum"=3406, "Octal Digit?"=1129, "Octal String To Number"=1186, "Old VISA Open"=1921, "One Button Dialog"=1340, "Open Application Reference"=8012, "Open Device"=1430, "Open File"=1403, "Open File (New)"=8050, "Open Tank"=21752, "Open Tank 1"=3074, "Open VI Object Reference"=8013, "Open VI Reference"=8010, "Or"=1062, "Or Array Elements"=1910, "PPoll"=1969, "PPollConfig"=1970, "PPollUnconfig"=1971, "PassControl"=1968, "Path Constant"=2009, "Path To String"=1077, "Path Type"=1421, "Path to Array of Strings"=1423, "Pi"=2014, "Pi Divided By 2"=2016, "Pi Multiplied By 2"=2015, "Pick Line"=1510, "Pict Ring"=21602, "Pict Ring 1"=3015, "Picture"=3508, "PixMap"=3505, "PixMap (Do not touch it!!)"=3507, "Planck Constant (J/Hz)"=2026, "Platform Flat Square Button"=3134, "Plug-In Control"=21820, "Polar To Complex"=1047, "Positive Infinity"=2025, "Power Of 10"=1212, "Power Of 2"=1223, "Power Of X"=1213, "Pressure Tank"=3075, "Pressure Tank 1"=21753, "Preview Queue Element"=9112, "Printable?"=1124, "Property Node"=1920, "Pulldown Menu Ring"=3061, "Push Button"=21001, "Quit LabVIEW"=1352, "Quotient & Remainder"=1056, "Radio Buttons"=22001, "Raised Box"=3637, "Raised Box 1"=3600, "Raised Circle"=3603, "Raised Down Triangle"=3615, "Raised Frame"=3606, "Raised Left Triangle"=3612, "Raised Right Triangle"=3613, "Raised Rounded Box"=3609, "Raised Up Triangle"=3614, "Random Number (0-1)"=1070, "RcvRespMsg"=1972, "Re/Im To Complex"=1046, "Read Binary File"=8051, "Read Device"=1432, "Read File"=1407, "ReadStatus"=1973, "Receive"=1974, "ReceiveSetup"=1975, "Recessed Box"=3601, "Recessed Circle"=3604, "Recessed Down Triangle"=3619, "Recessed Frame"=3607, "Recessed Left Triangle"=3616, "Recessed Menu Ring"=3019, "Recessed Right Triangle"=3617, "Recessed Rounded Box"=3610, "Recessed Up Triangle"=3618, "Reciprocal"=1059, "Reciprocal Of Pi"=2017, "Reciprocal Of e"=2021, "Rectangular Stop Button"=3128, "Refnum to Path"=1424, "Refnum to Session"=2306, "Register Event Callback"=2078, "Register For Events"=2065, "Register Session"=2319, "Release Notifier"=9102, "Release Queue"=9109, "Replace Array Subset"=3910, "Replace Substring"=3913, "Request Deallocation"=1610, "ResetSys"=1976, "Reshape Array"=2055, "Reverse 1D Array"=1900, "Reverse String"=1537, "Right Arrow"=3825, "Right Bow Valve"=21765, "Right Bow Valve 1"=3705, "Right Bow Valve 2"=3805, "Right Down Elbow"=3817, "Right Down Elbow 1"=3717, "Right Pump"=3719, "Right Pump 1"=3819, "Right Rect Valve"=3804, "Right Rect Valve 1"=3704, "Right Rect Valve 2"=21764, "Right Tee"=3715, "Right Tee 1"=3815, "Right Up Elbow"=3814, "Right Up Elbow 1"=3714, "Ring Constant"=2008, "Rocker"=21002, "Rotary Feeder"=3830, "Rotate"=1082, "Rotate 1D Array"=1906, "Rotate Left With Carry"=1606, "Rotate Right With Carry"=1607, "Rotate String"=1536, "Round Button"=3100, "Round LED"=21012, "Round LED 1"=3120, "Round Light"=3104, "Round Push Button"=3112, "Round Push Button 2"=3118, "Round Radio Button"=3106, "Round Stop Button"=3127, "Round To +Infinity"=1076, "Round To -Infinity"=1075, "Round To Nearest"=1055, "Rydberg Constant (/m)"=2031, "Scale By Power Of 2"=1074, "Scan From File"=2082, "Scan From String"=2080, "Scan String For Tokens"=8101, "Scan Value"=1534, "Search 1D Array"=1901, "Search and Replace String"=3914, "Search/Split String"=1538, "Secant"=1203, "Seconds To Date/Time"=1309, "Seek"=1409, "Select"=1516, "Send"=1977, "Send Notification"=9104, "SendCmds"=1978, "SendDataBytes"=1979, "SendIFC"=1980, "SendLLO"=1982, "SendList"=1981, "SendSetup"=1983, "Session to Refnum"=2307, "Set Menu Item Info"=9006, "Set Occurrence"=1702, "Set Variant Attribute"=8204, "Set Waveform Attribute"=8207, "SetRWLS"=1984, "SetTimeOut"=1985, "Sign"=1049, "Simple Horizontal Slide"=3003, "Simple Numeric"=2900, "Simple Numeric 1"=3029, "Simple String"=2115, "Simple Vertical Slide"=3002, "Simulation Loop"=2099, "Sinc"=1227, "Sine"=1200, "Sine & Cosine"=1220, "Single Selection Listbox"=21200, "Size Handle"=1603, "Slide Switch"=21011, "Sort 1D Array"=1120, "Speed Of Light In Vacuum (m/sec)"=2028, "Split 1D Array"=1908, "Split Button"=21020, "Split Number"=1170, "Split Signals"=2351, "Spreadsheet String To Array"=1539, "Square Button"=3101, "Square LED"=3121, "Square LED 1"=21013, "Square Light"=3105, "Square Push Button"=3113, "Square Push Button 2"=3119, "Square Radio Button"=3107, "Square Root"=1060, "Stacked Sequence Structure"=2000, "Standard ListBox"=3202, "State Diagram"=2051, "Static VI Reference"=2084, "Stop"=1350, "Stop Button"=21230, "String Constant"=2007, "String Control"=3200, "String Control 1"=21701, "String Indicator"=3201, "String Indicator 1"=21702, "String Length"=1502, "String Subset"=1503, "String To Byte Array"=1608, "String To IP"=1711, "String To Path"=1078, "String to Tag"=1830, "Strip Path"=1420, "SubPanel"=21810, "SubPanel (Classic)"=21811, "Subtract"=1051, "Swap Bytes"=1162, "Swap Vector Element"=1912, "Swap Words"=1163, "TCP Close Connection"=1713, "TCP Create Listener"=1717, "TCP Flattened Read"=1718, "TCP Flattened Write"=1719, "TCP Flex Read"=1720, "TCP Flex Write"=1721, "TCP Network Connection Refnum"=3407, "TCP Open Connection"=1715, "TCP Read"=1716, "TCP Wait On Listener"=1712, "TCP Write"=1714, "Tab Constant"=2012, "Tab Control"=3332, "Tab Control 1"=3330, "Table"=3301, "Table 1"=21202, "Table 2"=21212, "Tag Attribute Ring"=2063, "Tag Constant"=2089, "Tag Control"=21742, "Tag Control 1"=3302, "Tag Indicator"=21743, "Tag Indicator 1"=3303, "Tag to String"=1831, "Tangent"=1202, "Tank"=3020, "Tank 1"=21006, "Temporary Directory"=1435, "TestSRQ"=1986, "TestSys"=1987, "Text & Pict Ring"=21603, "Text & Pict Ring 1"=3016, "Text Button"=21015, "Text Ring"=21601, "Text Ring 1"=3014, "Thermometer"=21007, "Thermometer 1"=3021, "Thick Chiseled Line"=3630, "Thick Line"=3629, "Thick Line with Arrow"=3631, "Thick Lowered Box"=3635, "Thin Chiseled Line"=3627, "Thin Line"=3626, "Thin Line with Arrow"=3628, "Threshold 1D Array"=1909, "Tick Count (ms)"=1300, "Time Stamp Constant"=2068, "Time Stamp Control"=5555, "Time Stamp Control 1"=21913, "Time Stamp Indicator"=5556, "Time Stamp Indicator 1"=21914, "Timed Loop"=5570, "To Byte Integer"=1140, "To Double Precision Complex"=1152, "To Double Precision Float"=1147, "To Extended Precision Complex"=1154, "To Extended Precision Float"=1149, "To Long Integer"=1142, "To Lower Case"=1189, "To More Generic Class"=8017, "To More Specific Class"=8016, "To OLE Variant"=8002, "To Quad Integer"=1155, "To Single Precision Complex"=1151, "To Single Precision Float"=1146, "To Time Stamp"=5560, "To Unsigned Byte Integer"=1143, "To Unsigned Long Integer"=1145, "To Unsigned Quad Integer"=1156, "To Unsigned Word Integer"=1144, "To Upper Case"=1188, "To Variant"=8201, "To Word Integer"=1141, "Traditional DAQ Channel"=21733, "Traditional DAQ Channel 1"=3320, "Traditional DAQ Channel Constant"=2085, "Transpose 2D Array"=1902, "Tree"=21793, "Trigger"=1988, "TriggerList"=1989, "Two Button Dialog"=1341, "Type Cast"=1166, "Type and Creator"=1434, "UDP Close"=1726, "UDP Multicast Open"=1727, "UDP Network Connection Refnum"=3418, "UDP Open"=1723, "UDP Read"=1724, "UDP Write"=1725, "Unbundle"=2048, "Unbundle By Name"=2058, "Unflatten From String"=1161, "Unflatten From XML"=8401, "Uniform Dbl Waveform"=3312, "Uniform Int16 Waveform"=3313, "Unregister For Events"=2076, "Unregister Session"=2320, "Up Arrow"=3823, "Up Bow Valve"=3703, "Up Bow Valve 1"=21763, "Up Bow Valve 2"=3803, "Up Rect Valve"=21762, "Up Rect Valve 1"=3702, "Up Rect Valve 2"=3802, "Up Tee"=3812, "Up Tee 1"=3712, "User Item"=3506, "VI Library"=1425, "VI Refnum"=3422, "VISA Assert Interrupt Signal"=2309, "VISA Assert Trigger"=1929, "VISA Assert Utility Signal"=2310, "VISA Clear"=1927, "VISA Close"=1922, "VISA Disable Event"=1940, "VISA Discard Events"=1941, "VISA Enable Event"=1942, "VISA Find Resource"=1923, "VISA Flush I/O Buffer"=2302, "VISA GPIB Command"=2315, "VISA GPIB Control ATN"=2316, "VISA GPIB Control REN"=2304, "VISA GPIB Pass Control"=2317, "VISA GPIB Send IFC"=2318, "VISA In 16"=1930, "VISA In 32"=1944, "VISA In 8"=1936, "VISA Lock"=1993, "VISA Map Address"=1932, "VISA Map Trigger"=2311, "VISA Memory Allocation"=1997, "VISA Memory Free"=1998, "VISA Move"=2303, "VISA Move In 16"=1948, "VISA Move In 32"=1991, "VISA Move In 8"=1946, "VISA Move Out 16"=1949, "VISA Move Out 32"=1992, "VISA Move Out 8"=1947, "VISA Open"=2308, "VISA Out 16"=1931, "VISA Out 32"=1945, "VISA Out 8"=1937, "VISA Peek 16"=1934, "VISA Peek 32"=1995, "VISA Peek 8"=1938, "VISA Poke 16"=1935, "VISA Poke 32"=1996, "VISA Poke 8"=1939, "VISA Read"=1925, "VISA Read STB"=1928, "VISA Read To File"=2313, "VISA Refnum to Session"=2300, "VISA Resource Name"=21737, "VISA Resource Name Constant"=3421, "VISA Set I/O Buffer Size"=2301, "VISA Status Description"=1924, "VISA USB Control In"=2086, "VISA USB Control Out"=2087, "VISA Unlock"=1994, "VISA Unmap Address"=1933, "VISA Unmap Trigger"=2312, "VISA VXI Cmd or Query"=2305, "VISA Wait on Event"=1943, "VISA Write"=1926, "VISA Write From File"=2314, "VISA resource name"=3409, "Variant"=3310, "Variant To Data"=8003, "Variant To Flattened String"=8203, "Vert Line"=3822, "Vert Pipe"=3716, "Vert Pipe 1"=3816, "Vert Rocker"=21740, "Vertical Fill Slide"=21014, "Vertical Fill Slide 1"=3009, "Vertical Graduated Bar"=21107, "Vertical Pointer Slide"=21017, "Vertical Pointer Slide 1"=3007, "Vertical Progress Bar"=21104, "Vertical Slide"=3004, "Vertical Slide Switch"=21741, "Vertical Slide Switch 1"=3115, "Vertical Smooth Box"=3634, "Vertical Switch"=3109, "Vertical Toggle Switch"=21005, "Vertical Toggle Switch 1"=3111, "Volume Info"=1414, "Wait (ms)"=1302, "Wait For Activity"=1722, "Wait For Front Panel Activity"=1328, "Wait Until Next ms Multiple"=1327, "Wait for GPIB RQS"=1952, "Wait on Notification"=9105, "Wait on Notification from Multiple"=9106, "Wait on Occurrence"=1701, "WaitSRQ"=1990, "Waveform Chart"=3501, "Waveform Chart 1"=21717, "Waveform Chart 2"=21010, "Waveform Graph"=21703, "Waveform Graph 1"=3504, "While Loop"=2003, "While Loop 1"=2352, "White Space?"=1125, "Write Device"=1431, "Write File"=1408, "XY Graph"=3500, "XY Graph 1"=21716, "Xmath Script"=9022]
                  # "Insert a Dummy Attirbute"
                  n829 = New VI Object(vi object class=w1938, owner refnum=w1936, style=w1939, position/next to=T16 {"Horizontal"=0, "Vertical"=0} ("relative position/next to refnum"), 8:w1937) -> (object refnum=w1934:refnum<vi>, 0:w1933:errorcluster)  [unwired: 3 in]
                  n830 = property class="Boolean"(reference=w1934, error in=w1933, "Label.Text"="None") -> (reference out=w1931:refnum<vi>, error out=w1930:errorcluster)
                  n831 = Close Reference(reference=w1931, error in (no error)=w1930) -> (error out=w1929:errorcluster)
                }
              }
              n832 = Close Reference(reference=w1909, error in (no error)=w1902) -> ()  [unwired: 1 out]
              n833 = Close Reference(reference=w1904, error in (no error)=w1902) -> ()  [unwired: 1 out]
              n834 = Close Reference(reference=w1901, error in (no error)=w1902) -> ()  [unwired: 1 out]
              n835 = Close Reference(reference=w1906, error in (no error)=w1902) -> (error out=w1898:errorcluster)
              n836 = call <resource>:"ConvertGoop3ToGoop4_ClearErrors.vi"("error in (no error)"=w1898) -> ("error out"=w1897:errorcluster)  [unwired: 9 in, 1 out]
            }
            frame True {
            }
          }
        }
      }
      frame "MakeVIsProtected" {
        n837 = Unbundle By Name(w1961) -> ("AppRef"=w1957:refnum<vi>, "Classes"=w1958:T2[])
        n838 = for {
          tunnel: w1958 -> [w1971] mode=indexing
          shift-right: [w1964] -> w1959
          shift-left: w1960 -> [w1967]
          tunnel: w1957 -> [_]
          n839 = Unbundle By Name(w1971) -> ("ClassRef"=w1968:refnum<vi>)
          n840 = invoke class="LVClassLibrary" method="Get All Descendents"(reference=w1968, error in=w1967) -> (reference out=w1966:refnum<vi>, error out=w1970:errorcluster, "All Descendents"=w1963:refnum<vi>[])  [unwired: 5 in, 4 out]
          n841 = for {
            tunnel: w1963 -> [w1980] mode=indexing
            shift-right: [w1974] -> w1969
            shift-left: w1970 -> [w1978]
            tunnel: w1966 -> [w1975]
            tunnel: string[] ["GetAttributes", "New\\2Evi$", "GetClassAttributes"] -> [w1973]
            n842 = property class="ProjectItem"(reference=w1980, error in=w1978) -> (reference out=w1977:refnum<vi>, error out=w1979:errorcluster, "Name"=w1976:string)
            n843 = for {
              tunnel: w1976 -> [w1984]
              tunnel: [w1982] -> w1972
              tunnel: w1973 -> [w1981] mode=indexing
              stop <- w1982 stop-if-true
              n844 = Match Pattern(string=w1984, regular expression=w1981) -> (offset past match=w1983:i32)  [unwired: 1 in, 3 out]
              n845 = Greater Or Equal To 0?(x=w1983) -> (x >= 0?=w1982:bool)
            }
            n846 = case shown="True" w1972 {
              tunnel: w1977 -> [_ w1989]
              tunnel: w1979 -> [w1985 w1987]
              tunnel: w1975 -> [_ w1990]
              tunnel: [w1985 w1986] -> w1974
              frame False {
              }
              frame True {
                n847 = invoke class="LVClassLibrary" method="Set Source Scope"(reference=w1990, error in=w1987, "SourceRef"=w1989, "Scope"=T17."protected" ("scope")) -> (error out=w1986:errorcluster)  [unwired: 1 in, 4 out]
              }
            }
          }
          n848 = invoke class="LVClassLibrary" method="Save"(reference=w1966, error in=w1969) -> (error out=w1965:errorcluster)  [unwired: 2 in, 3 out]
          n849 = Close Reference(reference=w1963, error in (no error)=w1965) -> (error out=w1964:errorcluster)
        }
        n850 = call <resource>:"ConvertGoop3ToGoop4_UpdateProgressList.vi"("String"="Make VIs Protected") -> ()  [unwired: 10 in, 1 out]
      }
      frame "UpdateNewViCallers" {
        n851 = Unbundle By Name(w1996) -> ("Classes"=w1997:T2[])
        n852 = call <resource>:"ConvertGoop3ToGoop4_UpdateProgressList.vi"("String"="FindGetAttributeVIs") -> ("error out"=w1991:errorcluster)  [unwired: 10 in]
        n853 = for {
          tunnel: w1997 -> [w2002] mode=indexing
          shift-right: [w2000] -> w1994
          shift-left: w1995 -> [w1999]
          tunnel: w1991 -> [_]
          n854 = Unbundle By Name(w2002) -> ("ClassRef"=w2001:refnum<vi>)
          n855 = invoke class="LVClassLibrary" method="Get All Descendents"(reference=w2001, error in=w1999, "Type"="VI") -> (error out=w1998:errorcluster, "All Descendents"=w2003:refnum<vi>[])  [unwired: 4 in, 5 out]
          n856 = for {
            tunnel: w2003 -> [w2014] mode=indexing
            shift-right: [w2009] -> w2000
            shift-left: w1998 -> [w2010]
            n857 = property class="ProjectItem"(reference=w2014, error in=w2010) -> (reference out=w2013:refnum<vi>, error out=w2011:errorcluster, "Reference"=w2012:refnum<vi>, "Name"=w2008:string)
            n858 = Match Pattern(string=w2008, regular expression="GetObjectStatus.vi$") -> (offset past match=w2006:i32)  [unwired: 1 in, 3 out]
            n859 = Greater Or Equal To 0?(x=w2006) -> (x >= 0?=w2005:bool)
            n860 = Close Reference(reference=w2013) -> ()  [unwired: 1 in, 1 out]
            n861 = case shown="True" w2005 {
              tunnel: w2012 -> [w2021 w2045]
              tunnel: w2011 -> [w2020 w2044]
              tunnel: [w2017 w2041] -> w2009
              frame False {
                n862 = invoke class="VI" method="Get VI Dependencies"(reference=w2021, error in=w2020, "Include Standard VIs?"=TRUE) -> (reference out=w2018:refnum<vi>, error out=w2019:errorcluster, "Dependency Names"=w2023:string[])  [unwired: 16 in, 16 out]
                n863 = for {
                  tunnel: w2023 -> [w2026] mode=indexing
                  tunnel: "New\\2Evi$" -> [w2025]
                  tunnel: [w2024] -> w2016
                  stop <- w2024 stop-if-true
                  n864 = Match Pattern(string=w2026, regular expression=w2025) -> (offset past match=w2027:i32)  [unwired: 1 in, 3 out]
                  n865 = Greater Or Equal To 0?(x=w2027) -> (x >= 0?=w2024:bool)
                }
                n866 = case shown="True" w2016 {
                  tunnel: w2019 -> [w2029 w2035]
                  tunnel: w2018 -> [w2030 w2033]
                  tunnel: [w2028 w2031] -> w2017
                  frame False {
                    n867 = Close Reference(reference=w2030, error in (no error)=w2029) -> (error out=w2028:errorcluster)
                  }
                  frame True {
                    n868 = call <resource>:"ConvertGoop3ToGoop4_Log.vi"("error in (no error)"=w2035, "Object"=w2033) -> ("error out"=w2034:errorcluster)  [unwired: 7 in, 2 out]
                    n869 = call <resource>:"ConvertGoop3ToGoop4_UpdateNewVICallers.vi"("error in (no error)"=w2034, "InsertAlwaysCopy"=FALSE, "ViRef"=w2033) -> ("error out"=w2039:errorcluster, "ViRefOut"=w2040:refnum<vi>)  [unwired: 7 in]
                    n870 = invoke class="VI" method="Save.Instrument"(reference=w2040, error in=w2039) -> (reference out=w2038:refnum<vi>, error out=w2037:errorcluster)  [unwired: 4 in, 4 out]
                    n871 = Close Reference(reference=w2038, error in (no error)=w2037) -> (error out=w2032:errorcluster)
                    n872 = call <resource>:"ConvertGoop3ToGoop4_ClearErrors.vi"("error in (no error)"=w2032) -> ("error out"=w2031:errorcluster)  [unwired: 9 in, 1 out]
                  }
                }
              }
              frame True {
                n873 = invoke class="VI" method="Save.Instrument"(reference=w2045, error in=w2044) -> (reference out=w2042:refnum<vi>, error out=w2043:errorcluster)  [unwired: 4 in, 4 out]
                n874 = Close Reference(reference=w2042, error in (no error)=w2043) -> (error out=w2041:errorcluster)
              }
            }
          }
        }
      }
      frame "UpdateDestory" {
        n875 = Unbundle By Name(w2052) -> ("Classes"=w2049:T2[])
        n876 = call <resource>:"ConvertGoop3ToGoop4_UpdateProgressList.vi"("String"="Update Destory") -> ("error out"=w2046:errorcluster)  [unwired: 10 in]
        n877 = for {
          tunnel: w2049 -> [w2062] mode=indexing
          shift-right: [w2055] -> w2050
          shift-left: w2051 -> [w2058]
          tunnel: w2046 -> [_]
          n878 = Unbundle By Name(w2062) -> ("ClassRef"=w2059:refnum<vi>)
          n879 = invoke class="LVClassLibrary" method="Get All Descendents"(reference=w2059, error in=w2058) -> (reference out=w2057:refnum<vi>, error out=w2061:errorcluster, "All Descendents"=w2054:refnum<vi>[])  [unwired: 5 in, 4 out]
          n880 = for {
            tunnel: w2054 -> [w2070] mode=indexing
            shift-right: [w2064] -> w2060
            shift-left: w2061 -> [w2069]
            tunnel: w2057 -> [_]
            tunnel: string[] ["Destroy.vi$", "CleanUp.vi$"] -> [w2067]
            stop <- w2066 stop-if-true
            n881 = property class="ProjectItem"(reference=w2070, error in=w2069) -> (reference out=w2063:refnum<vi>, error out=w2065:errorcluster, "Name"=w2068:string)
            n882 = for {
              tunnel: w2068 -> [w2086]
              tunnel: [w2084] -> w2066
              tunnel: w2067 -> [w2083] mode=indexing
              stop <- w2084 stop-if-true
              n883 = Match Pattern(string=w2086, regular expression=w2083) -> (offset past match=w2085:i32)  [unwired: 1 in, 3 out]
              n884 = Greater Or Equal To 0?(x=w2085) -> (x >= 0?=w2084:bool)
            }
            n885 = case shown="True" w2066 {
              tunnel: w2065 -> [w2071 w2081]
              tunnel: [w2071 w2072] -> w2064
              tunnel: w2063 -> [_ w2082]
              frame False {
              }
              frame True {
                n886 = property class="ProjectItem"(reference=w2082, error in=w2081) -> (error out=w2076:errorcluster, "Reference"=w2074:refnum<vi>)  [unwired: 1 out]
                n887 = call <resource>:"ConvertGoop3ToGoop4_Log.vi"("error in (no error)"=w2076, "Object"=w2074) -> ("error out"=w2075:errorcluster)  [unwired: 7 in, 2 out]
                n888 = call <resource>:"ConvertGoop3ToGoop4_UpDateDestroy.vi"("error in (no error)"=w2075, "ViRefIn"=w2074) -> ("error out"=w2079:errorcluster, "ViRefOut"=w2080:refnum<vi>)  [unwired: 8 in]
                n889 = invoke class="VI" method="Save.Instrument"(reference=w2080, error in=w2079) -> (reference out=w2077:refnum<vi>, error out=w2078:errorcluster)  [unwired: 4 in, 4 out]
                n890 = Close Reference(reference=w2077, error in (no error)=w2078) -> (error out=w2073:errorcluster)
                n891 = call <resource>:"ConvertGoop3ToGoop4_ClearErrors.vi"("error in (no error)"=w2073) -> ("error out"=w2072:errorcluster)  [unwired: 9 in, 1 out]
              }
            }
          }
          n892 = invoke class="LVClassLibrary" method="Save"(reference=w2057, error in=w2060) -> (error out=w2056:errorcluster)  [unwired: 2 in, 3 out]
          n893 = Close Reference(reference=w2054, error in (no error)=w2056) -> (error out=w2055:errorcluster)
        }
      }
      frame "DeleteNotUsedClassItems" {
        n894 = Unbundle By Name(w2089) -> ("Classes"=w2095:T2[])
        n895 = for {
          tunnel: w2095 -> [w2101] mode=indexing
          shift-right: [w2103] -> w2092
          shift-left: w2093 -> [w2106]
          shift-right: [w2096] -> w2087
          shift-left: path[] [] -> [w2097]
          n896 = Unbundle By Name(w2101) -> ("ClassName"=w2100:string, "UsingClassAttributes"=w2098:bool)
          n897 = Unbundle By Name(w2101) -> ("ClassRef"=w2102:refnum<vi>)
          n898 = invoke class="LVClassLibrary" method="Get All Descendents"(reference=w2102, error in=w2106, "Type"="VI") -> (error out=w2105:errorcluster, "All Descendents"=w2107:refnum<vi>[])  [unwired: 4 in, 5 out]
          n899 = case shown="False" w2098 {
            tunnel: [string[] ["GetAttributesToModify\\2Evi$", "SetModifiedAttributes\\2Evi$", "Delete\\2Evi$", "GOOPKernel\\2Evi$", "GetClassAttributesToModify\\2Evi$", "SetModifiedClassAttributes\\2Evi$", "CastToMoreSpecific\\2Evi$"] ("file names") string[] ["GetAttributesToModify\\2Evi$", "SetModifiedAttributes\\2Evi$", "Delete\\2Evi$", "GOOPKernel\\2Evi$", "GetClassAttributesToModify\\2Evi$", "SetModifiedClassAttributes\\2Evi$", "CastToMoreSpecific\\2Evi$", "GetClassAttributes\\2Evi$", "ClassAttributes\\2Ectl$"] ("file names")] -> w2099
            frame True {
            }
            frame False {
            }
          }
          n900 = for {
            tunnel: w2107 -> [w2123] mode=indexing
            shift-right: [w2120] -> w2104
            shift-left: w2105 -> [w2121]
            tunnel: w2100 -> [w2117]
            tunnel: w2099 -> [w2116]
            shift-right: [w2112] -> w2096
            shift-left: w2097 -> [w2111]
            n901 = property class="ProjectItem"(reference=w2123, error in=w2121) -> (reference out=w2118:refnum<vi>, error out=w2122:errorcluster, "Reference"=w2115:refnum<vi>, "Path"=w2114:path)
            n902 = Strip Path(path=w2114) -> (name=w2113:string)  [unwired: 1 out]
            n903 = for {
              tunnel: [w2124] -> w2119
              tunnel: w2113 -> [w2126]
              tunnel: w2116 -> [w2125] mode=indexing
              stop <- w2124 stop-if-true
              n904 = Match Pattern(string=w2126, regular expression=w2125) -> (offset past match=w2127:i32)  [unwired: 1 in, 3 out]
              n905 = Greater Or Equal To 0?(x=w2127) -> (x >= 0?=w2124:bool)
            }
            n906 = case shown="True" w2119 {
              tunnel: w2118 -> [w2131 w2142]
              tunnel: w2122 -> [w2130 w2144]
              tunnel: [w2130 w2140] -> w2120
              tunnel: w2115 -> [w2129 w2151]
              tunnel: w2114 -> [_ w2150]
              tunnel: w2117 -> [_ _]
              tunnel: [w2128 w2137] -> w2112
              tunnel: w2111 -> [w2128 w2136]
              frame False {
                n907 = Close Reference(reference=w2131) -> ()  [unwired: 1 in, 1 out]
                n908 = Close Reference(reference=w2129) -> ()  [unwired: 1 in, 1 out]
              }
              frame True {
                n909 = call <resource>:"ConvertGoop3ToGoop4_Log.vi"("error in (no error)"=w2144, "Object"=w2142) -> ("error out"=w2143:errorcluster)  [unwired: 7 in, 2 out]
                n910 = Strip Path(path=w2150) -> (stripped path=w2146:path, name=w2148:string)
                n911 = Concatenate Strings("-DeleteMe-" ("string"), w2148) -> (w2147:string)
                n912 = Build Path(base path=w2146, name or relative path=w2147) -> (appended path=w2138:path)
                n913 = invoke class="VI" method="Save.Instrument"(reference=w2151, error in=w2143, "Path to saved file"=w2138) -> (reference out=w2145:refnum<vi>, error out=w2135:errorcluster)  [unwired: 3 in, 4 out]
                n914 = call <resource>:"CommonVIs_Wait.vi"("error in"=w2135) -> ("error out"=w2134:errorcluster)  [unwired: 9 in]
                n915 = invoke class="ProjectItem" method="Delete"(reference=w2142, error in=w2134) -> (error out=w2149:errorcluster)  [unwired: 1 in, 2 out]
                n916 = call <vilib>:"Clear Errors.vi"("error in (no error)"=w2149) -> ("error out"=w2141:errorcluster)  [unwired: 5 in, 1 out]
                n917 = Delete(path (use dialog)=w2150, error in=w2141) -> ()  [unwired: 3 in, 3 out]
                n918 = Delete(path (use dialog)=w2138, error in=w2141) -> ()  [unwired: 3 in, 3 out]
                n919 = invoke class="VI" method="FP.Close"(reference=w2145, error in=w2141) -> (reference out=w2133:refnum<vi>, error out=w2132:errorcluster)  [unwired: 1 in, 1 out]
                n920 = Build Array (concatenate)(w2136, w2138) -> (w2137:path[])
                n921 = call <resource>:"ConvertGoop3ToGoop4_ClearErrors.vi"("error in (no error)"=w2141) -> ("error out"=w2140:errorcluster)  [unwired: 9 in, 1 out]
                n922 = Close Reference(reference=w2133, error in (no error)=w2132) -> ()  [unwired: 1 out]
              }
            }
          }
          n923 = invoke class="LVClassLibrary" method="Save"(reference=w2102, error in=w2104) -> (error out=w2103:errorcluster)  [unwired: 2 in, 3 out]
        }
        n924 = call <resource>:"ConvertGoop3ToGoop4_UpdateProgressList.vi"("String"="Deleting Project files") -> ()  [unwired: 10 in, 1 out]
        n925 = Bundle By Name(cluster=w2089, "DeleteTheseFiles"=w2087) -> (w2088:T7)
      }
      frame "DeleteSomeProjectFiles" {
        n926 = Unbundle By Name(w2157) -> ("Classes"=w2158:T2[])
        n927 = local read "ApplyDebuggingSupport"() -> (w2155:bool)
        n928 = for {
          tunnel: w2158 -> [w2161] mode=indexing
          shift-right: [w2163] -> w2154
          shift-left: w2156 -> [w2167]
          tunnel: w2155 -> [w2165]
          # "ObjectReference.ctl"
          n929 = Unbundle By Name(w2161) -> ("ClassRef"=w2162:refnum<vi>)
          n930 = Unbundle By Name(w2161) -> ("ClassName"=w2160:string, "ObjectStatusUsed"=w2159:bool)
          n931 = invoke class="LVClassLibrary" method="Get All Descendents"(reference=w2162, error in=w2167, "Type"="VI") -> (error out=w2166:errorcluster, "All Descendents"=w2168:refnum<vi>[])  [unwired: 4 in, 5 out]
          n932 = for {
            tunnel: w2168 -> [w2186] mode=indexing
            shift-right: [w2183] -> w2164
            shift-left: w2166 -> [w2184]
            tunnel: w2165 -> [w2179]
            tunnel: w2160 -> [w2172]
            tunnel: w2159 -> [w2170]
            n933 = property class="ProjectItem"(reference=w2186, error in=w2184) -> (reference out=w2180:refnum<vi>, error out=w2185:errorcluster, "Name"=w2176:string, "Reference"=w2178:refnum<vi>, "Path"=w2173:path)
            n934 = Match Pattern(string=w2176, regular expression="GetObjectStatus.vi$") -> (offset past match=w2181:i32)  [unwired: 1 in, 3 out]
            n935 = Match Pattern(string=w2176, regular expression="ObjectReference.ctl$") -> (offset past match=w2177:i32)  [unwired: 1 in, 3 out]
            n936 = Greater Or Equal To 0?(x=w2181) -> (x >= 0?=w2171:bool)
            n937 = Greater Or Equal To 0?(x=w2177) -> (x >= 0?=w2174:bool)
            n938 = case shown="False" w2171 {
              tunnel: w2180 -> [w2193 w2221]
              tunnel: w2185 -> [w2191 w2220]
              tunnel: [w2190 w2219] -> w2183
              tunnel: w2179 -> [_ w2216]
              tunnel: w2178 -> [w2189 w2218]
              tunnel: w2174 -> [w2192 _]
              tunnel: w2173 -> [w2188 w2217]
              tunnel: w2172 -> [w2187 _]
              tunnel: w2170 -> [_ w2214]
              frame False {
                n939 = case shown="True" w2192 {
                  tunnel: w2193 -> [w2195 w2213]
                  tunnel: w2191 -> [w2194 w2207]
                  tunnel: [w2194 w2204] -> w2190
                  tunnel: w2189 -> [w2196 w2206]
                  tunnel: w2188 -> [_ w2212]
                  tunnel: w2187 -> [_ w2211]
                  frame False {
                    n940 = Close Reference(reference=w2195) -> ()  [unwired: 1 in, 1 out]
                    n941 = Close Reference(reference=w2196) -> ()  [unwired: 1 in, 1 out]
                  }
                  frame True {
                    n942 = Strip Path(path=w2212) -> (stripped path=w2208:path, name=w2210:string)
                    n943 = Concatenate Strings(w2211, w2210) -> (w2209:string)
                    n944 = Build Path(base path=w2208, name or relative path=w2209) -> (appended path=w2203:path)
                    n945 = invoke class="VI" method="Save.Instrument"(reference=w2206, error in=w2207, "Path to saved file"=w2203) -> (reference out=w2205:refnum<vi>, error out=w2198:errorcluster)  [unwired: 3 in, 4 out]
                    n946 = call <resource>:"CommonVIs_Wait.vi"("error in"=w2198) -> ("error out"=w2197:errorcluster)  [unwired: 9 in]
                    n947 = invoke class="ProjectItem" method="Delete"(reference=w2213, error in=w2197) -> (reference out=w2200:refnum<vi>, error out=w2199:errorcluster)  [unwired: 1 in, 1 out]
                    n948 = Close Reference(reference=w2200, error in (no error)=w2199) -> ()  [unwired: 1 out]
                    n949 = call <vilib>:"Clear Errors.vi"("error in (no error)"=w2199) -> ("error out"=w2204:errorcluster)  [unwired: 5 in, 1 out]
                    n950 = Delete(path (use dialog)=w2212, error in=w2204) -> ()  [unwired: 3 in, 3 out]
                    n951 = Delete(path (use dialog)=w2203, error in=w2204) -> ()  [unwired: 3 in, 3 out]
                    n952 = invoke class="VI" method="FP.Close"(reference=w2205, error in=w2204) -> (reference out=w2201:refnum<vi>, error out=w2202:errorcluster)  [unwired: 1 in, 1 out]
                    n953 = Close Reference(reference=w2201, error in (no error)=w2202) -> ()  [unwired: 1 out]
                  }
                }
              }
              frame True {
                n954 = Compound Arithmetic op=OR(w2216, w2214) -> (w2215:bool)
                n955 = case shown="False" w2215 {
                  tunnel: w2221 -> [w2230 w2232]
                  tunnel: w2220 -> [w2229 w2233]
                  tunnel: [w2226 w2233] -> w2219
                  tunnel: w2218 -> [w2228 w2231]
                  tunnel: w2217 -> [w2227 _]
                  frame False {
                    n956 = invoke class="ProjectItem" method="Delete"(reference=w2230, error in=w2229) -> (reference out=w2222:refnum<vi>, error out=w2223:errorcluster)  [unwired: 1 in, 1 out]
                    n957 = Close Reference(reference=w2222, error in (no error)=w2223) -> ()  [unwired: 1 out]
                    n958 = call <vilib>:"Clear Errors.vi"("error in (no error)"=w2223) -> ("error out"=w2226:errorcluster)  [unwired: 5 in, 1 out]
                    n959 = Delete(path (use dialog)=w2227, error in=w2226) -> ()  [unwired: 3 in, 3 out]
                    n960 = invoke class="VI" method="FP.Close"(reference=w2228, error in=w2226) -> (reference out=w2224:refnum<vi>, error out=w2225:errorcluster)  [unwired: 1 in, 1 out]
                    n961 = Close Reference(reference=w2224, error in (no error)=w2225) -> ()  [unwired: 1 out]
                  }
                  frame True {
                    n962 = Close Reference(reference=w2232) -> ()  [unwired: 1 in, 1 out]
                    n963 = Close Reference(reference=w2231) -> ()  [unwired: 1 in, 1 out]
                  }
                }
              }
            }
          }
          n964 = invoke class="LVClassLibrary" method="Save"(reference=w2162, error in=w2164) -> (error out=w2163:errorcluster)  [unwired: 2 in, 3 out]
        }
        n965 = call <resource>:"ConvertGoop3ToGoop4_UpdateProgressList.vi"("String"="Deleting Project files") -> ()  [unwired: 10 in, 1 out]
      }
      frame "OpenProject" {
        n966 = Unbundle By Name(w2234) -> ("ProjectRef"=w2242:refnum<vi>)
        n967 = invoke class="Project" method="Open Window"(reference=w2242, error in=w2241) -> (reference out=w2239:refnum<vi>, error out=w2238:errorcluster)  [unwired: 1 in, 1 out]
        n968 = invoke class="Project" method="Save"(reference=w2239, error in=w2238) -> (error out=w2236:errorcluster)  [unwired: 2 in, 3 out]
        n969 = Unbundle By Name(w2234) -> ("Classes"=w2237:T2[])
        n970 = for {
          tunnel: w2237 -> [w2254] mode=indexing
          shift-right: [w2243] -> w2235
          shift-left: w2236 -> [w2252]
          n971 = Unbundle By Name(w2254) -> ("ClassRef"=w2253:refnum<vi>, "GetAttViRefs"=w2251:refnum<vi>[], "ViRefs"=w2250:refnum<vi>[])
          n972 = invoke class="LVClassLibrary" method="Save"(reference=w2253, error in=w2252) -> (reference out=w2249:refnum<vi>, error out=w2248:errorcluster)  [unwired: 2 in, 2 out]
          n973 = Close Reference(reference=w2251) -> ()  [unwired: 1 in, 1 out]
          n974 = Close Reference(reference=w2250) -> ()  [unwired: 1 in, 1 out]
          n975 = invoke class="LVClassLibrary" method="Get All Descendents"(reference=w2249, error in=w2248, "Type"="VI") -> (error out=w2244:errorcluster, "All Descendents"=w2245:refnum<vi>[])  [unwired: 4 in, 5 out]
          n976 = for {
            tunnel: w2245 -> [w2258] mode=indexing
            tunnel: [w2255] -> w2246 mode=indexing
            n977 = property class="ProjectItem"(reference=w2258) -> (reference out=w2255:refnum<vi>, "Reference"=w2257:refnum<vi>)  [unwired: 1 in, 1 out]
            n978 = invoke class="VI" method="Save.Instrument"(reference=w2257) -> (reference out=w2256:refnum<vi>)  [unwired: 5 in, 5 out]
            n979 = Close Reference(reference=w2256) -> ()  [unwired: 1 in, 1 out]
          }
          n980 = Close Reference(reference=w2246) -> ()  [unwired: 1 in, 1 out]
          n981 = Close Reference(reference=w2245, error in (no error)=w2244) -> (error out=w2243:errorcluster)
        }
      }
      frame "Done" {
        n982 = Unbundle By Name(w2268) -> ("error"=w2267:errorcluster)
        n983 = Select(t="Error occurred", s=w2267, f="Done") -> (s? t:f=w2263:string)
        n984 = Build Array(w2263) -> (w2262:string[])
        n985 = property on="Done" class="Bool"("Visible"=TRUE, "Strings [4]"=w2262) -> ()  [unwired: 2 in, 2 out]
        n986 = property on="Tab" class="TabCtl (strict)"("Value"=T1."Converting" ("Tab")) -> ()  [unwired: 2 in, 2 out]
        n987 = Enqueue Element(queue=w2259, element=TRUE) -> ()  [unwired: 2 in, 3 out]
      }
      frame "CheckForBrokenVIs" {
        n988 = Unbundle By Name(w2280) -> ("Classes"=w2281:T2[])
        n989 = call <resource>:"ConvertGoop3ToGoop4_UpdateProgressList.vi"("error in (no error)"=w2273, "String"="Check For broken VIs") -> ("error out"=w2274:errorcluster)  [unwired: 9 in]
        n990 = for {
          tunnel: w2281 -> [w2290] mode=indexing
          tunnel: [w2289] -> w2275 mode=indexing
          tunnel: [w2286] -> w2277 mode=indexing
          tunnel: w2274 -> [_]
          n991 = Unbundle By Name(w2290) -> ("ClassRef"=w2288:refnum<vi>)
          n992 = invoke class="LVClassLibrary" method="Get All Descendents"(reference=w2288, "Type"="VI") -> ("All Descendents"=w2291:refnum<vi>[])  [unwired: 5 in, 6 out]
          n993 = for {
            tunnel: w2291 -> [w2300] mode=indexing
            shift-right: [w2293] -> w2285
            shift-left: string[] [] -> [w2298]
            n994 = property class="ProjectItem" props=["Reference", "Name"](reference=w2300) -> (reference out=w2299:refnum<vi>, "Reference"=w2294:refnum<vi>)  [unwired: 1 in, 2 out]
            n995 = Close Reference(reference=w2299) -> ()  [unwired: 1 in, 1 out]
            n996 = property class="VI"(reference=w2294) -> (reference out=w2297:refnum<vi>, "Exec.State"=w2296:T20, "Name"=w2295:string)  [unwired: 1 in, 1 out]
            n997 = case shown="\"Idle\", Default" w2296 {
              tunnel: w2295 -> [w2303 _]
              tunnel: [w2301 w2304] -> _
              tunnel: w2298 -> [w2302 w2304]
              tunnel: [w2301 w2304] -> w2293
              frame "Bad" {
                n998 = Build Array (concatenate)(w2302, w2303) -> (w2301:string[])
              }
              frame "Idle", Default {
              }
            }
            n999 = Close Reference(reference=w2297) -> ()  [unwired: 1 in, 1 out]
          }
          n1000 = Bundle By Name(cluster=w2290, "BrokenVIs"=w2285) -> (w2289:T2)
          n1001 = Empty Array?(array=w2285) -> (empty?=w2286:bool)
        }
        n1002 = And Array Elements(Boolean array=w2277) -> (logical AND=w2272:bool)
        n1003 = case shown="True" w2272 {
          tunnel: ["BrokenVIEndResult" "Idle"] -> w2276
          frame False {
          }
          frame True {
            w2283 = "Done"
            n1004 = property class="VI"("Front Panel.Title"=w2283) -> ()  [unwired: 2 in, 2 out]
            n1005 = call <resource>:"ConvertGoop3ToGoop4_UpdateProgressList.vi"("String"=w2283) -> ()  [unwired: 10 in, 1 out]
          }
        }
        n1006 = Bundle By Name(cluster=w2280, "Classes"=w2275, "Log"=FALSE) -> (w2279:T7)
      }
      frame "BrokenVIEndResult" {
        n1007 = call <resource>:"ConvertGoop3ToGoop4_ClearErrors.vi"() -> ("Errors"=w2308:string[])  [unwired: 10 in, 1 out]
        n1008 = Unbundle By Name(w2306) -> ("Classes"=w2313:T2[])
        n1009 = Unbundle By Name(w2306) -> ("AppRef"=w2305:refnum<vi>)
        n1010 = for {
          tunnel: w2313 -> [w2318] mode=indexing
          shift-right: [w2316] -> w2311
          shift-left: string[] [] -> [w2315]
          n1011 = Unbundle By Name(w2318) -> ("BrokenVIs"=w2317:string[])
          n1012 = Build Array (concatenate)(w2315, w2317) -> (w2316:string[])
        }
        n1013 = call <resource>:"ConvertGoop3ToGoop4_ShowBrokenVIs.vi"("BrokenVIs"=w2311, "AppRef"=w2305, "ErrorsVIs"=w2308) -> ()  [unwired: 1 in]
        n1014 = stacked-sequence {
          frame #0 {
            n1015 = property class="VI"("Front Panel.Title"="Done" ("Front Panel Window:Title")) -> ()  [unwired: 2 in, 2 out]
          }
        }
        n1016 = call <resource>:"ConvertGoop3ToGoop4_UpdateProgressList.vi"("String"="Done (broken VIs found)") -> ()  [unwired: 10 in, 1 out]
      }
      frame "----------------------------------------------" {
      }
      frame "CloseProjectAndExit" {
        n1017 = Unbundle By Name(w2327) -> ("ProjectRef"=w2328:refnum<vi>, "My Computer"=w2323:refnum<vi>, "AppRef"=w2322:refnum<vi>)
        n1018 = Close Reference(reference=w2322) -> ()  [unwired: 1 in, 1 out]
        n1019 = Close Reference(reference=w2323) -> ()  [unwired: 1 in, 1 out]
        n1020 = invoke class="Project" method="Close Window"(reference=w2328) -> (reference out=w2325:refnum<vi>, error out=w2324:errorcluster)  [unwired: 2 in, 1 out]
        n1021 = Close Reference(reference=w2325, error in (no error)=w2324) -> ()  [unwired: 1 out]
      }
      frame "CloseRefs", "Error", Default {
        n1022 = case shown="Error" w2331 {
          selector: w2331 -> [w2358 w2363]
          tunnel: [w2358 w2363] -> w2330
          frame No Error {
          }
          frame Error {
            n1023 = Unbundle By Name(w2363) -> ("code"=w2362:i32, "source"=w2361:string)
            n1024 = Format Into String(format string="%d:%s", w2362, w2361) -> (resulting string=w2359:string)  [unwired: 2 in, 1 out]
            n1025 = call <resource>:"ConvertGoop3ToGoop4_Log.vi"("Object"=w2359) -> ()  [unwired: 8 in, 3 out]
          }
        }
        n1026 = call <resource>:"GDSError_LogErrorInformation.vi"("State"=w2353, "LocalVariableData"=w2351, "error in (no error)"=w2330) -> ("error out"=w2344:errorcluster)  [unwired: 16 in]
        n1027 = Unbundle By Name(w2351) -> ("Classes"=w2356:T2[])
        n1028 = Bundle By Name(cluster=w2351, "error"=w2344) -> (w2343:T7)
        n1029 = case shown="\"Error\"" w2354 {
          tunnel: w2353 -> [_ w2376]
          tunnel: w2330 -> [_ w2380]
          tunnel: ["Closing references" w2378] -> w2334
          frame "False", Default {
          }
          frame "Error" {
            w2381 = T29 0 items=["no dialog", "OK message", "continue or stop message", "OK message + warnings", "continue/stop + warnings"] ("type of dialog (OK msg:1)")
            n1030 = call <resource>:"ConvertGoop3ToGoop4_Log.vi"("Action(Enter)"=ConvertGoop3ToGoop4_LogType."Read") -> ("LastItem"=w2375:string)  [unwired: 8 in, 2 out]
            n1031 = call <vilib>:"General Error Handler.vi"("type of dialog (OK msg:1)"=w2381, "error in (no error)"=w2380) -> ("message"=w2379:string)  [unwired: 9 in, 4 out]
            n1032 = Format Into String(format string="Error occurred in \"%s\"\nVI:%s\n%s", w2376, w2375, w2379) -> (resulting string=w2378:string)  [unwired: 2 in, 1 out]
          }
        }
        n1033 = call <resource>:"ConvertGoop3ToGoop4_UpdateProgressList.vi"("String"=w2334) -> ("error out"=w2335:errorcluster)  [unwired: 10 in]
        n1034 = stacked-sequence {
          tunnel: w2335 -> [w2372]
          tunnel: [w2372] -> w2341
          frame #0 {
            n1035 = Wait (ms)(milliseconds to wait=u32 5) -> ()  [unwired: 1 out]
          }
        }
        n1036 = for {
          tunnel: w2356 -> [w2386] mode=indexing
          shift-right: [w2385] -> w2355
          shift-left: errorcluster {"status"=FALSE, "code"=0, "source"=""} ("error out") -> [w2383]
          tunnel: [w2384] -> w2339 mode=indexing
          tunnel: w2341 -> [_]
          n1037 = Unbundle By Name(w2386) -> ("ClassRef"=w2384:refnum<vi>)
          n1038 = invoke class="LVClassLibrary" method="Save"(reference=w2384, error in=w2383) -> (error out=w2385:errorcluster)  [unwired: 2 in, 3 out]
        }
        n1039 = disable-structure shown="Disabled" {
          disable-tunnel: w2355 -> [w2366 w2371]
          disable-tunnel: [w2365 w2371] -> w2340
          disable-tunnel: w2339 -> [w2364 _]
          frame Disabled {
            n1040 = for {
              shift-right: [w2369] -> w2365
              shift-left: w2366 -> [w2370]
              tunnel: w2364 -> [w2368] mode=indexing
              n1041 = call <resource>:"GDSLvClass_SaveEverythingInClass.vi"("ClassRefIn"=w2368, "ForceResaving(False)"=TRUE, "error in"=w2370) -> ("error out"=w2369:errorcluster)  [unwired: 15 in, 1 out]
            }
          }
          frame Enabled {
          }
        }
        n1042 = Enqueue Element(queue=w2333, element=TRUE) -> ()  [unwired: 2 in, 3 out]
        n1043 = Unbundle By Name(w2343) -> ("AppRef"=w2345:refnum<vi>, "My Computer"=w2342:refnum<vi>, "ProjectRef"=w2349:refnum<vi>, "CopyClassesRef"=w2338:refnum<vi>[])
        n1044 = invoke class="Project" method="Save"(reference=w2349, error in=w2340) -> (reference out=w2347:refnum<vi>, error out=w2336:errorcluster)  [unwired: 2 in, 2 out]
        n1045 = Close Reference(reference=w2342, error in (no error)=w2336) -> (error out=w2348:errorcluster)
        n1046 = Close Reference(reference=w2347, error in (no error)=w2348) -> (error out=w2346:errorcluster)
        n1047 = Close Reference(reference=w2339, error in (no error)=w2336) -> (error out=w2337:errorcluster)
        n1048 = Close Reference(reference=w2345, error in (no error)=w2346) -> ()  [unwired: 1 out]
        n1049 = Close Reference(reference=w2338, error in (no error)=w2337) -> ()  [unwired: 1 out]
      }
    }
    n1050 = Equal?(x=w59, y="Exit") -> (x = y?=w62:bool)
    n1051 = Select(t="Error", s=w51, f=w59) -> (s? t:f=w63:string)
    "State" <- w44
  }
  n1052 = Dequeue Element(queue=w19, error in (no error)=w4) -> (queue out=w16:refnum<queue>, error out=w20:errorcluster)  [unwired: 1 in, 2 out]
  n1053 = case shown="No Error" w20 {
    selector: w20 -> [w2389 _]
    tunnel: w16 -> [w2388 _]
    frame No Error {
      n1054 = Get Date/Time In Seconds() -> (seconds since 1Jan1904=w2387:timestamp)
      n1055 = while {
        tunnel: w2387 -> [w2406]
        tunnel: w2389 -> [w2396]
        tunnel: w2388 -> [w2390]
        stop <- w2391 continue-if-true
        n1056 = Dequeue Element(queue=w2390, timeout in ms (-1)=1000, error in (no error)=w2396) -> (timed out?=w2393:bool, error out=w2394:errorcluster)  [unwired: 2 out]
        n1057 = Unbundle By Name(w2394) -> ("status"=w2392:bool)
        n1058 = Compound Arithmetic op=AND(w2393, invert w2392) -> (w2391:bool)
        n1059 = Get Date/Time In Seconds() -> (seconds since 1Jan1904=w2407:timestamp)
        n1060 = Subtract(x=w2407, y=w2406) -> (x-y=w2405:dbl)
        n1061 = Quotient & Remainder(x=w2405, y=3600.0) -> (x-y*floor(x/y)=w2403:dbl, floor(x/y)=w2401:dbl)
        n1062 = Quotient & Remainder(x=w2403, y=60.0) -> (x-y*floor(x/y)=w2399:dbl, floor(x/y)=w2400:dbl)
        n1063 = Format Into String(format string="%02d:%02d:%02d", w2401, w2400, w2399) -> (resulting string=→"Timer":string)  [unwired: 2 in, 1 out]
      }
    }
    frame Error {
    }
  }
  n1064 = disable-structure shown="Disabled" {
    frame Disabled {
      n1065 = call <resource>:"ConvertGoop3ToGoop4_ClearErrors.vi"() -> ()  [unwired: 10 in, 2 out]
    }
    frame Enabled {
    }
  }
  n1066 = Unbundle By Name(w32) -> ("error"=w30:errorcluster, "DeleteTheseFiles"=w11:path[])
  n1067 = Release Queue(queue=w18) -> ()  [unwired: 2 in, 3 out]
  n1068 = call <resource>:"GDSError_ReportError.vi"("error in (no error)"=w30) -> ("error out"=w2:errorcluster)  [unwired: 18 in]
  "error out" <- w2
  n1069 = for {
    tunnel: w11 -> [w2409] mode=indexing
    tunnel: [w2408] -> w1
    n1070 = Delete(path (use dialog)=w2409) -> (error out=w2408:errorcluster)  [unwired: 4 in, 2 out]
  }
  n1071 = stacked-sequence {
    tunnel: w25 -> [w2416]
    tunnel: w2 -> [_]
    tunnel: w1 -> [_]
    frame #0 {
      n1072 = property on="Tab" class="TabCtl (strict)"("Value"=T1."SelectDir" ("Tab")) -> (error out=w2411:errorcluster)  [unwired: 2 in, 1 out]
      n1073 = property on="Progress" class="LstBox (strict)"(error in=w2411, "Top Row"=0) -> (error out=w2410:errorcluster)  [unwired: 1 in, 1 out]
      n1074 = property class="VI"(reference=w2416, error in=w2410, "Front Panel.Open"=FALSE ("Front Panel Window:Open")) -> (reference out=w2415:refnum<vi>, error out=w2417:errorcluster)
      n1075 = Close Reference(reference=w2415, error in (no error)=w2417) -> ()  [unwired: 1 out]
    }
  }
